vi "LS Durability One Hour Main (RT).vi"() -> ()   [LabVIEW 2013]
uses:
  Type Defs/App Config.ctl
  Type Defs/Controller Names.ctl
  SubVIs/Data Logger/Data Log Init.ctl
  Controls/Alarm Config.ctl
  Controls/Alarm Definition.ctl
  Controls/Alarm Profile Config.ctl
  Type Defs/Controller List.ctl
  Controls/Tank CMDs.ctl
  Controls/Controller Config.ctl
  Controls/Pump Data.ctl
  Controls/Tank Data.ctl
  Controls/HMI Cluster.ctl
  Controls/HMI Header.ctl
  Controls/HMI Tog Buttons.ctl
  Controls/HMI Mom Buttons.ctl
  Type Defs/LS Data.ctl
  Type Defs/Sequence States.ctl
  Controls/App Global Mode.ctl
  Controls/RPi HMI Mode.ctl
  Controls/Email Mode.ctl
  Type Defs/Pump Data Mode.ctl
  SubVIs/Watlow Modbus/Modbus Mode.ctl
  SubVIs/Watlow Modbus/Modbus Variable.ctl
  Controls/HMI Global Mode.ctl
  <vilib>/FPGAPlugInAG/sbRIO-9626/niLvFpga_Open_sbRIO-9626.vi
  <vilib>/Utility/error.llb/Error Cluster From Error Code.vi
  <vilib>/rvi/errors/niLvFpgaAdjustHostInterfaceError.vi
  <vilib>/Utility/file.llb/Write To Spreadsheet File (string).vi
  <vilib>/rvi/interface/nirviOpenFPGA/nirviOpenFPGA.xnode
  Controls/FPGA_OneHour_Reference.ctl
  FPGA Bitfiles/LSDurabilityMain_Alternate.lvbitx
  <vilib>/rvi/interface/nirviReadWriteControl/nirviReadWriteControl.xnode
  <vilib>/Utility/config.llb/NI_LVConfig.lvlib
  Controls/Power Supply Global Mode.ctl
  SubVIs/Data Logger/Data Logger Mode.ctl
  SubVIs/Data Logger/Data Log Start.ctl
  <vilib>/rvi/errors/niLvFpgaMergeErrorWithErrorCode.vi
  NiFpgaLv.dll
panel:
  in  "Data File Name:":string
  in  "pb.Run Profile":bool
  in  "Bank 2":T1={"7"=TRUE, "8"=TRUE, "9"=TRUE, "10"=TRUE, "11"=TRUE, "12"=TRUE}
  in  "Bank 1":T2={"1"=TRUE, "2"=TRUE, "3"=TRUE, "4"=TRUE, "5"=TRUE, "6"=TRUE} caption="Present"
  out "Email Alarms Disabled":bool
  out "Recording":bool
  in  "Disable Alarm Email":bool
  in  "Temp Tolerance":dbl=3.0 min=0.0 max=999999.0 step=1.0
  in  "Thermocouple":enum16{"2 TC/2 Tanks", "1 TC/1 Tank"}(ring)
  out "ADC Errors":i32
  in  "pb.Tare Pressure":bool
  in  "Data Log Enabled":bool=TRUE
  in  "RPMhyst":fxp<+,25,6>=1.0
  in  "pb.FuelChange":bool
  in  "Controller Type:":T3
  in  "Target Pressure:":dbl
  in  "Target Voltage:":dbl
  in  "Tank 1 Fuel Type:":string
  in  "Tank 2 Fuel Type:":string
  in  "Stagger Time (ms):":i32
  out "Current Step:":i32=2
  out "Step Time Left:":dbl=0.21101045608520508
  out "Cycles Completed:":u32=17
  in  "pb.Cycle Reset":bool
  in  "Serial Numbers":T4
  out "Read Inputs (ms)":u32
  out "Update Screen (ms)":u32
  out "Run Step (ms)":u32
  in  "Fuel Change Tab":enum32{"Page 1", "Page 2"}(tab)
  in  "pb.Fuel Change OK":bool
  in  "Reset Tab":enum32{"Page 1", "Page 2"}(tab)
  in  "pb.Reset OK":bool
  in  "pb.Reset Cancel":bool
  in  "Save As Tab":enum32{"Page 1", "Page 2"}(tab)
  in  "New Profile Name:":string
  in  "pb.Save As OK":bool
  in  "pb.Save As Cancel":bool
  in  "Alarm Tab":enum32{"Page 1", "Page 2"}(tab)
  out "Alarm Message":string
  in  "pb.Alarm OK":bool
  in  "Set Time Tab":enum32{"Page 1", "Page 2"}(tab)
  in  "pb.Set Time OK":bool
  in  "pb.Set Time Cancel":bool
  in  "New Time":dbl format="%<%H:%M:%S>t"
  in  "Pump Timers Tab":enum32{"Page 1", "Page 2"}(tab)=enum."Page 2"
  in  "Stop Time Enable":bool
  in  "Stop Time:":dbl format="%<%H:%M:%S>t"
  in  "pb.Time Reset All":bool
  out "Elapsed Time:":dbl[](array[numeric]) format="%<%H:%M:%S>t"
  in  "pb.Resets":bool[](array[boolean])=[FALSE, FALSE, FALSE, FALSE, FALSE, FALSE]
  in  "pb.Sets":bool[](array[boolean])=[FALSE, FALSE, FALSE, FALSE, FALSE, FALSE]
  in  "LS Serial Numbers":T5 caption="Serial Numbers"
  out "CPU Usage:":dbl=7.74131899555212 format="%.1f"
  in  "Live Data Tab":enum32{"Page 1", "Page 2", "Page 3"}(tab)=enum."Page 2"
  in  "Controller\nCMD":dbl[](array[numeric])=[0.0, 0.0, 0.0, 0.0, 0.0, 0.0] format="%#.2f"
  out "Speed":dbl[](array[numeric]) caption="Speed\n(RPM)" format="%#.0f"
  out "ControllerCurrent":dbl[](array[numeric])=[0.015201568603515625, 0.00335693359375, 0.003021240234375, 0.12260055541992188, 0.06085968017578125, 0.052234649658203125] caption="Controller\nCurrent\n(DC)" format="%.1f"
  out "PumpCurrent":dbl[](array[numeric])=[0.015201568603515625, 0.00335693359375, 0.003021240234375, 0.12260055541992188, 0.06085968017578125, 0.052234649658203125] caption="Pump\nCurrent\n(RMS)" format="%.1f"
  out "Flow":dbl[](array[numeric])=[0.0, 0.0, 0.0, 0.125, 0.0625, 0.0625] caption="Flow\n(L/H)" format="%#.0f"
  out "Pressure":dbl[](array[numeric])=[0.015201568603515625, 0.00335693359375, 0.003021240234375, 0.12260055541992188, 0.06085968017578125, 0.052234649658203125] caption="Pressure\n(kPa)" format="%#.0f"
  out "Ave. Speed":dbl=7.74131899555212 format="%.1f"
  out "Voltages":dbl[](array[numeric])=[0.015201568603515625, 0.00335693359375, 0.003021240234375, 0.12260055541992188, 0.06085968017578125, 0.052234649658203125] caption="Pump\nVoltage\n(V)" format="%.1f"
  in  "Reset Anomalies":bool
  in  "Reset Total Cycles":bool
  out "Anomalies (Last Cycle)":i32[](array[numeric]) caption="Anomalies\n(Last Cycle)" format="%#.0f"
  out "Anomalies/Cycle":i32[](array[numeric]) caption="Anomalies/\nCycle" format="%#.0f"
  out "Cycles":u32[](array[numeric]) format="%#.0f"
  out "Anomalies Total":i32[](array[numeric]) caption="Anomalies\nTotal" format="%#.0f"
  out "Steps":u32[](array[numeric]) format="%#.0f"
  out "Total Cycles":u32[](array[numeric]) caption="Total\nCycles" format="%#.0f"
  in  "Reset Opens":bool
  out "Opens":i32[](array[numeric]) format="%#.0f"
  in  "App Config":T6={"Location"="Tanks 162-163", "Profiles Path"=path "c:/Profiles", "Current Profile"="", "CA Number"="", "Cycles Completed"=0, "Controller Type:"=enum."Kuhnke", "Stagger Time (ms)"=0, "Tank 1 Fuel"="", "Tank 2 Fuel"="", "Serial Numbers"={"Position 1 SN"="", "Position 2 SN"="", "Poaition 3 SN"="", "Position 4 SN"="", "Position 5 SN"="", "Position 6 SN"=""}, "Pumps Present"={"Pump 1"=FALSE, "Pump 2"=FALSE, "Pump 3"=FALSE, "Pump 4"=FALSE, "Pump 5"=FALSE, "Pump 6"=FALSE}, "VoltCtrlRef"="", "VoltageSelect"=FALSE, "Watlow Present"=TRUE, "Temp 1"=0.0, "Temp 2"=0.0, "V_Run PI?"=FALSE, "Voltage Limits"={"V_Step"=1e-05, "V_CmdMax"=0.0, "V_CmdMin"=0.0}, "Voltage Far PI"={"V_FarSlew"=10.0, "V_FarKp"=0.0, "V_FarKi"=0.0}, "Voltage Mid PI"={"V_MidSlew"=10.0, "V_MidKp"=0.0, "V_MidKi"=0.0}, "Voltage Close PI"={"V_CloseSlew"=10.0, "V_CloseKp"=0.0, "V_CloseKi"=0.0}, "Voltage Scale"={"V_FFm"=0.0, "V_FFb"=0.0}, "Voltage Cutoffs"={"V_MidCutoff"=0.0, "V_CloseCutoff"=0.0}, "Pressure Scale"={"Pres_FFm"=1e-05, "Pres_FFb"=0.0}, "Temp Format"=0, "Temp Tolerance"=0.0, "Target Voltage"=0.0, "Target Pressure"=0.0, "Data Log Init"={"Data Path"=path "u:/Data", "Data Log Rate (S/s)"=1, "AKLH Rate (Hours/S)"=0.1, "Sync Time Offset (min)"=180, "IP Last 3"=0, "WebDAV IP"="10.31.176.36"}, "Email Handler IP"="10.30.189.34", "ADC Check"=FALSE, "3 Pump Tank"=TRUE, "Cycle Threshold:"=3.0, "Cycle Pts to Avg:"=3, "Anomaly Threshold:"=3.0, "Normal Steps:"=3, "Step Threshold:"=3.0} {"Step Threshold:" min=0.0 max=999999.0 step=1.0; "Normal Steps:" max=999999 step=1; "Anomaly Threshold:" min=0.0 max=999999.0 step=1.0; "Cycle Pts to Avg:" max=999999 step=1; "Cycle Threshold:" min=0.0 max=999999.0 step=1.0}
  in  "Monitoring Tab":enum32{"Page 1", "Page 2"}(tab)
  out "Avg Press:":dbl=7.74131899555212
  in  "pb.E Stop":bool
  in  "Ignition Relay":T8
  in  "Power Relay":T8
  out "Temp2":dbl caption="Tank 2 Temp (C):" format="%.1f"
  out "Temp1":dbl caption="Tank 1 Temp (C):" format="%.1f"
  out "PS Actual (V):":dbl format="%.2f"
  in  "Power Supply Cmd:":dbl min=0.0 max=20.0 format="%#.2f"
  in  "PressureCMD":dbl caption="Pressure Cmd:" min=0.0 max=825.0 format="%#.2f"
  in  "Pumps Present":T8={"Pump 1"=TRUE, "Pump 2"=TRUE, "Pump 3"=TRUE, "Pump 4"=TRUE, "Pump 5"=TRUE, "Pump 6"=TRUE}
  in  "Tank 1 Temp Cmd:":dbl caption="deg C"
  in  "Tank 2 Temp Cmd:":dbl caption="deg C"
  in  "Title Tab":enum32{"Page 1", "Page 2"}(tab)
  in  "Title":string="LS Durability ONE HOUR Test, v1.4"
  out "Time/Date":string
  in  "Login":bool
  in  "pb.Stop Profile":bool
  in  "Main Tab":T9(tab)
  in  "Recording\nFrequency (Hz): 2":i32=2000
  in  "Recording\nDuration (s): 2":i32=3600
  in  "Record Constant":bool
  in  "Detection Mode:":u16(ring) items=["Anomalies", "Opens"]
  in  "Record During Profile":bool
  in  "Recording\nFrequency (Hz):":i32=1000
  in  "Recording\nDuration (s):":i32=10
  in  "Interval Between\nRecordings (s):":i32=600
  in  "LS Power (Freq):":dbl=4.1 min=0.1
  in  "LS Power (Duty):":dbl=1.64
  in  "Bank 2 Power State:":u16(ring) items=["0 - Off", "1 - On", "2 - Pulsing"]
  in  "Bank 1 Power State:":u16(ring) items=["0 - Off", "1 - On", "2 - Pulsing"]
  in  "CA Number:":string
  in  "Profile Name:":string(combo)="test"
  in  "pb.Save As":bool
  out "Location:":string
  in  "Profile:":string[][](table)=[["1", "2.0", "0.0", "0.0", "0.0", "67.6", "67.6", "67.6"], ["2", "1.0", "0.0", "0.0", "0.0", "10.0", "10.0", "10.0"]]
  out "Step:":i32=1
  out "Time:":i32=1
  out "Recording":bool
  out "Waveform Chart":dbl(graph)
  in  "Pause":bool
  in  "Position":i32=1 min=1 max=12 step=1
  in  "Subtract Noise":bool
  in  "Anomaly Threshold:":dbl=3.0 min=0.0 max=999999.0 step=1.0
  in  "Normal Steps:":u32=3 max=999999 step=1
  in  "Step Threshold:":dbl=3.0 min=0.0 max=999999.0 step=1.0
  in  "Cycle Pts to Avg:":i32=3 min=0 max=999999 step=1
  in  "Cycle Threshold:":dbl=3.0 min=0.0 max=999999.0 step=1.0
  in  "Note Tab":enum32{"Page 1", "Page 2"}(tab)
  in  "Stop Profile Note":string
  in  "pb.Note OK":bool
  in  "pb.Note Cancel":bool
  in  "Second Step Check":bool
  in  "Alarm Config":T10
  in  "WebDAV Push":bool
  in  "Concat Data":bool
  in  "Cutoffs":cluster{"Mid Range":dbl, "Close Range":dbl} {"Close Range" min=-100000.0 max=100000.0 step=1e-05 format="%#.5f"; "Mid Range" min=-100000.0 max=100000.0 step=1e-05 format="%#.5f"}
  in  "Mid PI":cluster{"Slew Rate":dbl, "Kp":dbl, "Ki":dbl}={"Slew Rate"=10.0, "Kp"=0.0, "Ki"=0.0} {"Ki" min=-100000.0 max=100000.0 step=1e-05 format="%#.5f"; "Kp" min=-100000.0 max=100000.0 step=1e-05 format="%#.5f"; "Slew Rate" min=0.0 max=1000000.0 step=0.01 format="%#.5f"}
  in  "Close PI":cluster{"Slew Rate":dbl, "Kp":dbl, "Ki":dbl}={"Slew Rate"=10.0, "Kp"=0.0, "Ki"=0.0} {"Ki" min=-100000.0 max=100000.0 step=1e-05 format="%#.5f"; "Kp" min=-100000.0 max=100000.0 step=1e-05 format="%#.5f"; "Slew Rate" min=0.0 max=1000000.0 step=0.01 format="%#.5f"}
  in  "Pressure Scale":cluster{"M":dbl, "B":dbl}={"M"=1e-05, "B"=0.0} {"B" min=-100000.0 max=100000.0 step=1e-05 format="%#.5f"; "M" min=-100000.0 max=100000.0 step=1e-05 format="%#.5f"}
  in  "Closed Loop Voltage":bool
  in  "Voltage Limits":cluster{"Step":dbl, "Max":dbl, "Min":dbl}={"Step"=1e-05, "Max"=0.0, "Min"=0.0} {"Min" min=0.0 max=10.0 step=1e-05 format="%#.5f"; "Max" min=0.0 max=10.0 step=1e-05 format="%#.5f"; "Step" min=0.0 max=100.0 step=1e-05 format="%#.5f"}
  in  "Far PI":cluster{"Slew Rate":dbl, "Kp":dbl, "Ki":dbl}={"Slew Rate"=10.0, "Kp"=0.0, "Ki"=0.0} {"Ki" min=-100000.0 max=100000.0 step=1e-05 format="%#.5f"; "Kp" min=-100000.0 max=100000.0 step=1e-05 format="%#.5f"; "Slew Rate" min=0.0 max=1000000.0 step=0.01 format="%#.5f"}
  in  "Voltage Scale":cluster{"M":dbl, "B":dbl} {"B" min=-100000.0 max=100000.0 step=1e-05 format="%#.5f"; "M" min=-100000.0 max=100000.0 step=1e-05 format="%#.5f"}
  # "Fuel Change was logged."
  # "Are you sure you want to reset?"
  # "Enter a new elapsed time."
  # "Pump Timers"
  # "Live Data"
  # "Level Sensor Monitor"
  # "Level Sensor Monitor"
  # "Manual Control"
  # "V"
  # "kPa"
  # "degC"
  # "degC"
  # "Data file note as to reason for stopping profile:"
  # "Voltage Control"
  # "Pressure Control"
  # "Data Server"
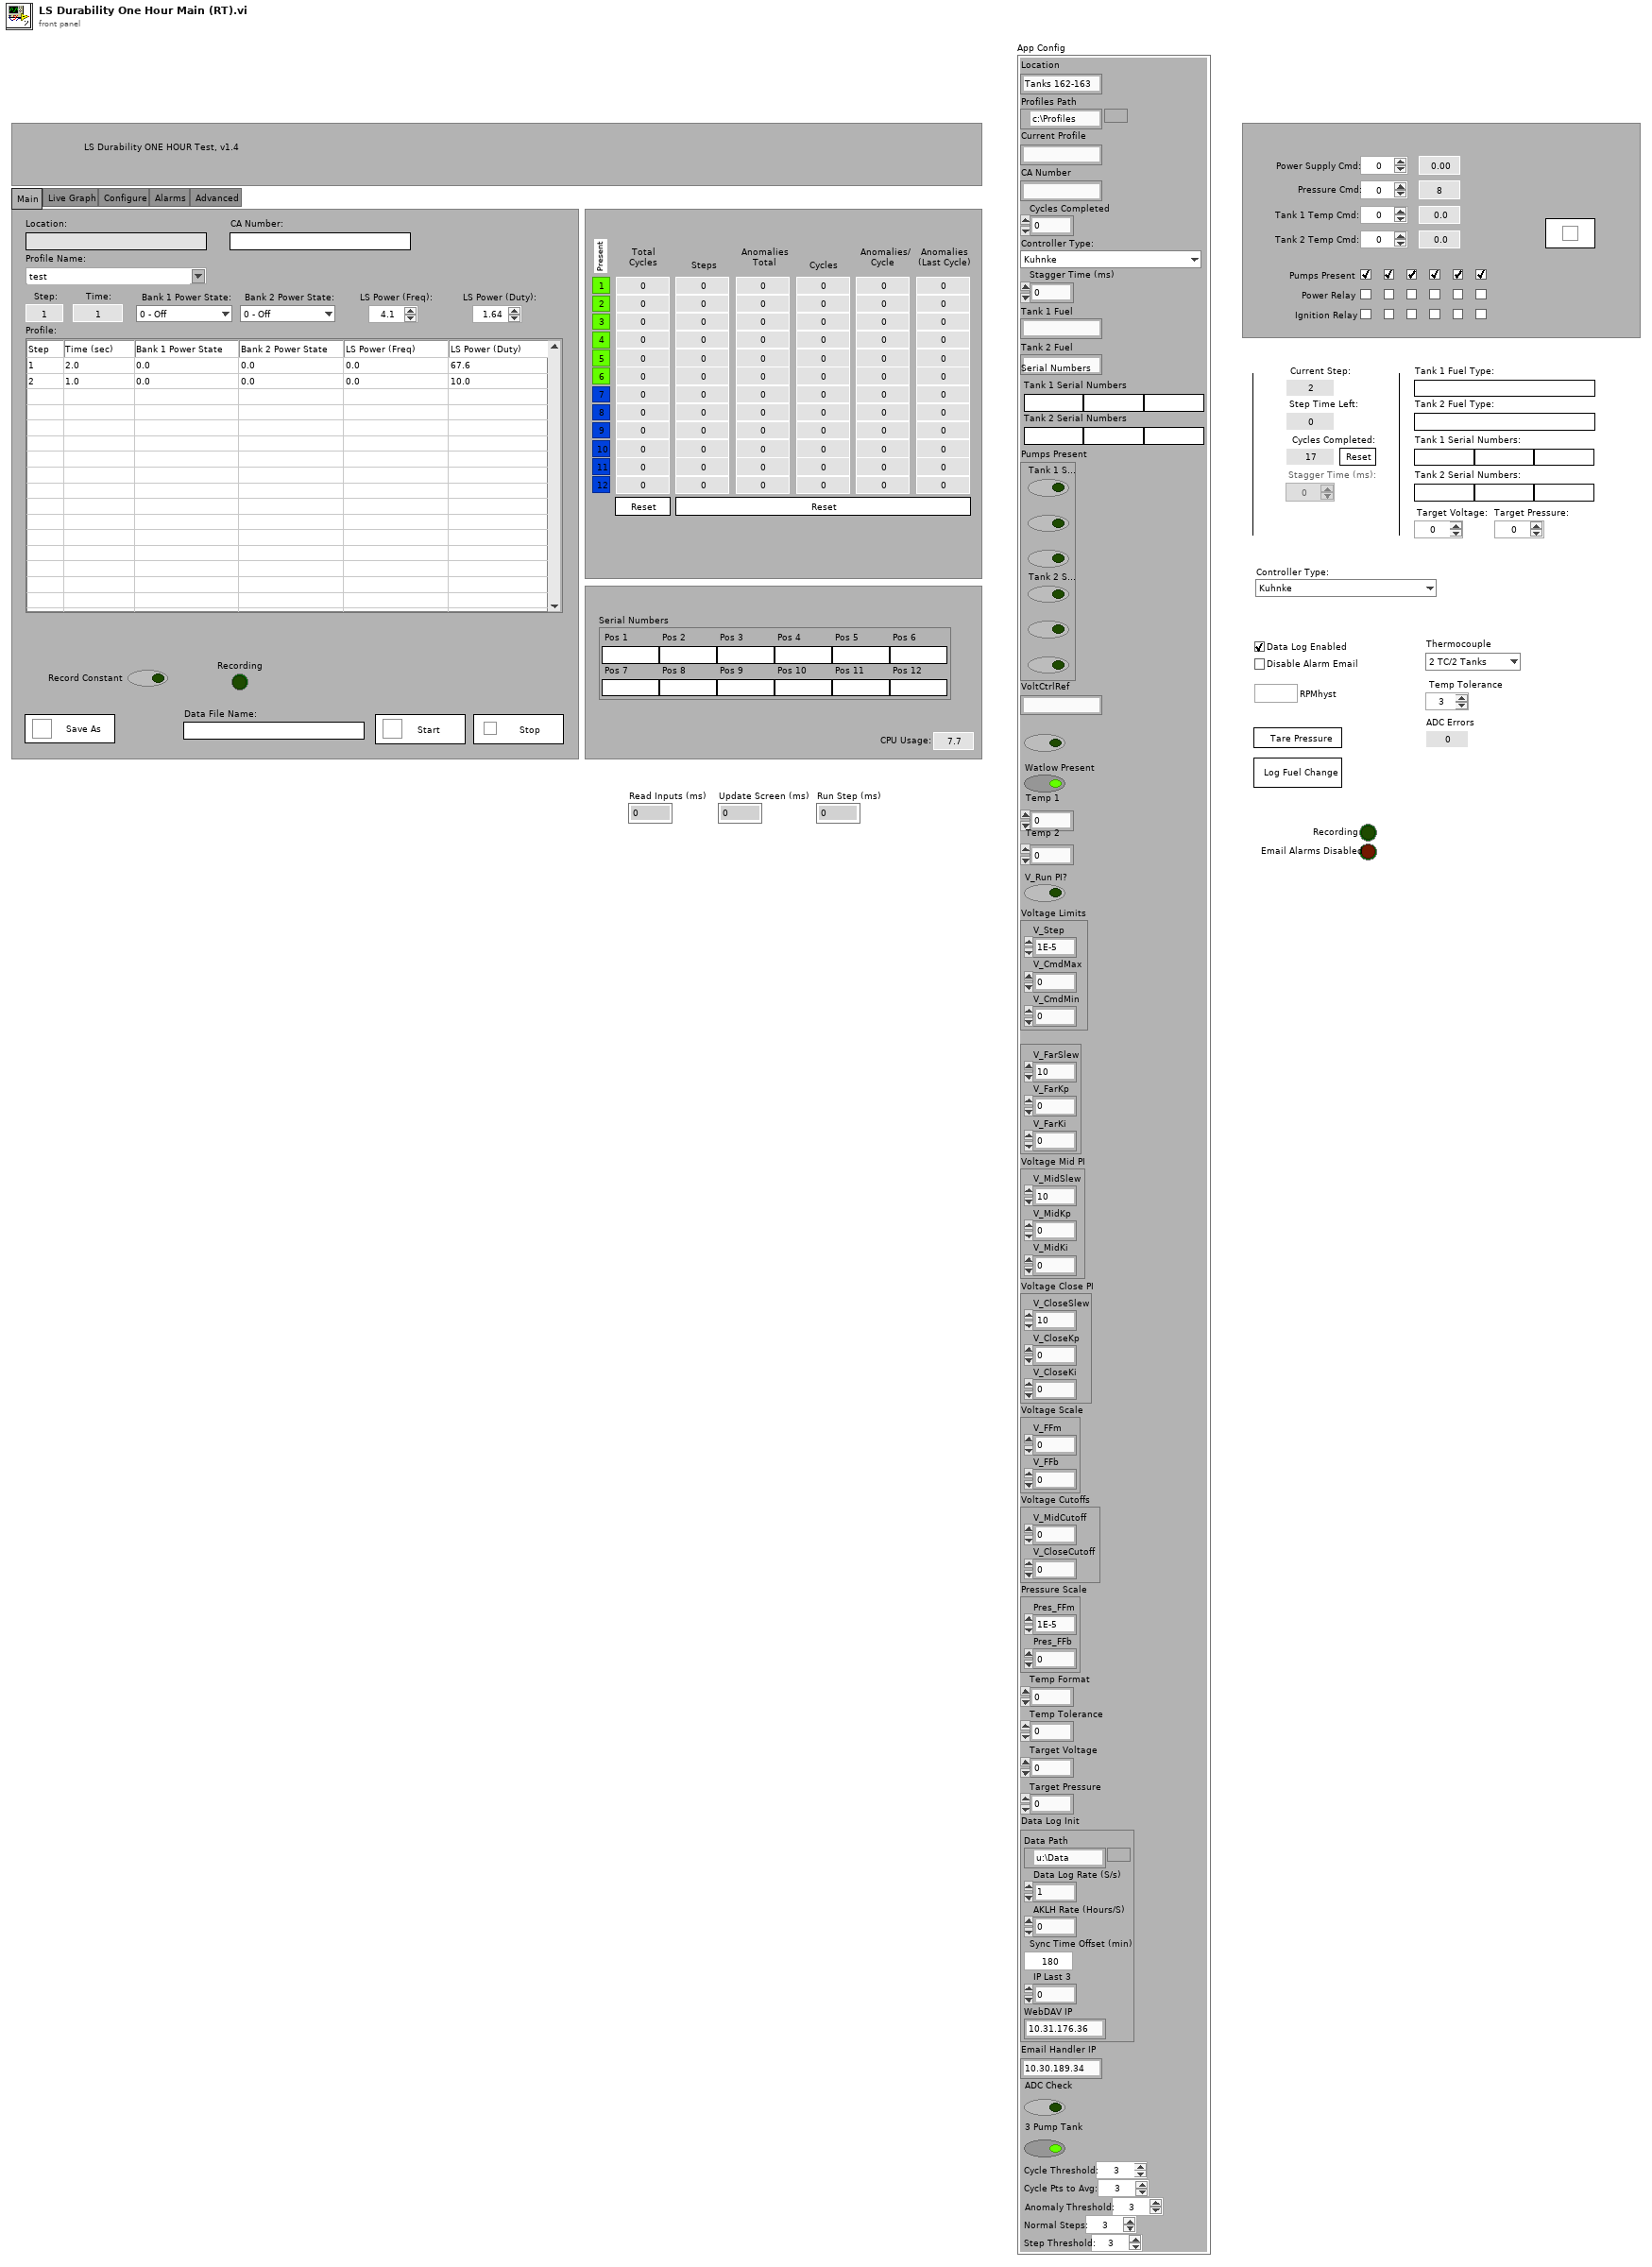
[diagram p1: front panel]
types:
  T1 = cluster{"7":bool, "8":bool, "9":bool, "10":bool, "11":bool, "12":bool}
  T2 = cluster{"1":bool, "2":bool, "3":bool, "4":bool, "5":bool, "6":bool}
  T3 = typedef "Controller Names.ctl" = enum16{"Kuhnke", "Helbako BLDC", "Conti", "Hella BLDC OL PWM", "Hella BLDC Turbine OL PWM", "Hella BLDC Pressure", "Helbako (old)", "TI PWM", "PSA", "Hella Gas", "Hella Diesel", "8 Comm", "10 Comm", "8 Comm Hella", "10 Comm Hella", "8 Comm Omron", "10 Comm Omron", "8 Comm Nissan", "10 Comm Nissan"}
  T4 = cluster{"Position 1 SN":string, "Position 2 SN":string, "Position 3 SN":string, "Position 4 SN":string, "Position 5 SN":string, "Position 6 SN":string}
  T5 = cluster{"Pos 1":string, "Pos 2":string, "Pos 3":string, "Pos 4":string, "Pos 5":string, "Pos 6":string, "Pos 7":string, "Pos 8":string, "Pos 9":string, "Pos 10":string, "Pos 11":string, "Pos 12":string}
  T6 = typedef "App Config.ctl" = cluster{"Location":string, "Profiles Path":path, "Current Profile":string, "CA Number":string, "Cycles Completed":u32, "Controller Type:":T3, "Stagger Time (ms)":i32, "Tank 1 Fuel":string, "Tank 2 Fuel":string, "Serial Numbers":cluster{"Position 1 SN":string, "Position 2 SN":string, "Poaition 3 SN":string, "Position 4 SN":string, "Position 5 SN":string, "Position 6 SN":string}, "Pumps Present":cluster{"Pump 1":bool, "Pump 2":bool, "Pump 3":bool, "Pump 4":bool, "Pump 5":bool, "Pump 6":bool}, "VoltCtrlRef":string, "VoltageSelect":bool, "Watlow Present":bool, "Temp 1":dbl, "Temp 2":dbl, "V_Run PI?":bool, "Voltage Limits":cluster{"V_Step":dbl, "V_CmdMax":dbl, "V_CmdMin":dbl}, "Voltage Far PI":cluster{"V_FarSlew":dbl, "V_FarKp":dbl, "V_FarKi":dbl}, "Voltage Mid PI":cluster{"V_MidSlew":dbl, "V_MidKp":dbl, "V_MidKi":dbl}, "Voltage Close PI":cluster{"V_CloseSlew":dbl, "V_CloseKp":dbl, "V_CloseKi":dbl}, "Voltage Scale":cluster{"V_FFm":dbl, "V_FFb":dbl}, "Voltage Cutoffs":cluster{"V_MidCutoff":dbl, "V_CloseCutoff":dbl}, "Pressure Scale":cluster{"Pres_FFm":dbl, "Pres_FFb":dbl}, "Temp Format":i32, "Temp Tolerance":dbl, "Target Voltage":dbl, "Target Pressure":dbl, "Data Log Init":T7, "Email Handler IP":string, "ADC Check":bool, "3 Pump Tank":bool, "Cycle Threshold:":dbl, "Cycle Pts to Avg:":i32, "Anomaly Threshold:":dbl, "Normal Steps:":u32, "Step Threshold:":dbl}
  T7 = typedef "Data Log Init.ctl" = cluster{"Data Path":path, "Data Log Rate (S/s)":u32, "AKLH Rate (Hours/S)":dbl, "Sync Time Offset (min)":i32, "IP Last 3":i32, "WebDAV IP":string}
  T8 = cluster{"Pump 1":bool, "Pump 2":bool, "Pump 3":bool, "Pump 4":bool, "Pump 5":bool, "Pump 6":bool}
  T9 = enum32{"Main", "Live Graph", "Configure", "Alarms", "Advanced"}
  T10 = typedef "Alarm Config.ctl" = cluster{"Alarms:":T11[], "Profile Sync:":T12}
  T11 = typedef "Alarm Definition.ctl" = cluster{"Description:":string, "Enabled:":bool, "Data Index:":i32, "Data Type:":string, "Low Limit:":dbl, "High Limit:":dbl, "Trip Time:":u32, "Profile Sync:":bool}
  T12 = typedef "Alarm Profile Config.ctl" = cluster{"Trip Time:":u32, "Consecutive Trips:":i32}
  T13 = cluster{"LS Power (Freq):":dbl, "LS Power (Duty):":dbl, "Bank 1 Present":cluster{"1":bool, "2":bool, "3":bool, "4":bool, "5":bool, "6":bool}, "Bank 2 Present":cluster{"7":bool, "8":bool, "9":bool, "10":bool, "11":bool, "12":bool}, "Data File Name:":string, "Record Bursts":bool, "RecInterval(s)":i32, "RecDuration(s)":i32, "RecFrequeny (Hz)":i32, "DetectionMode":i32, "Serial Numbers":string[], "Record Constant":bool, "2nd Step Check":bool, "Bias Resistances":dbl[], "Voltage(T)/Resistance(F)":bool}
  T14 = cluster{"LS Power (Freq):":dbl, "LS Power (Duty):":dbl, "Bank 1 Present":cluster{"1":bool, "2":bool, "3":bool, "4":bool, "5":bool, "6":bool}, "Bank 2 Present":cluster{"7":bool, "8":bool, "9":bool, "10":bool, "11":bool, "12":bool}, "Data File Name:":string, "Record Bursts":bool, "RecInterval(s)":i32, "RecDuration(s)":i32, "RecFrequeny (Hz)":i32, "DetectionMode":i32, "Serial Numbers":string[], "Record Constant":bool, "2nd Step Check":bool}
  T15 = typedef "Sequence States.ctl" = enum16{"Main", "Init Files", "Init", "Unused", "Save As", "Start Profile", "Check Step Time", "Alarm", "Alarm Dismiss", "Run Step", "Stop Profile", "Cycle Reset", "Time Reset", "Time Reset All", "Time Set", "Tare CTs", "Save Profile", "Open Profile", "Get Profiles", "Update Screen", "Update Controls", "Save App Config", "Write Outputs", "Disable Background", "Enable Background", "Get/Release Control", "Log Fuel Change", "Fuel Change Popup", "Read Inputs", "Remote Timer Reset", "Controller Change", "Get Alarms", "Init Alarms", "Save Alarms", "Voltage Selection", "Set Watlow Temp 1", "Set Watlow Temp 2", "Get Pressure", "Write Tare Pressure", "Adjust Controls", "Reinit ADC", "Write Initial Times", "Write Pumps Present", "HMI Command", "Save Pump Times", "Check Pump Stop Time", "Save LS App Config", "Init Data File", "Reset LS Cycles", "Reset Anomalies", "Reset Opens", "Save LS Data", "Save LS Test Data", "Check Serial Numbers", "Main Tab", "Allow Data Note"}
  T16 = typedef "LS Data.ctl" = cluster{"Total Cycles":u32[], "Steps":u32[], "Anomalies Total":i32[], "Cycles":u32[], "Anomalies/Cycle":i32[], "Anomalies (Last Cycle)":i32[], "Opens":i32[]}
  T17 = typedef "HMI Cluster.ctl" = cluster{"Error":errorcluster, "COM Ref":refnum<visa-resource-name>, "Pump Data":T18, "Tank Data":cluster{"PS Actual (V):":dbl, "Temp1":dbl, "Temp2":dbl}, "Power Relays":cluster{"Pump 1":bool, "Pump 2":bool, "Pump 3":bool, "Pump 4":bool, "Pump 5":bool, "Pump 6":bool}, "Pump CMDs":dbl[], "HMI Header":T19, "Tank CMDs":T20, "HMI Tog Buttons":T21, "In Test":bool, "HMI Command":bool, "HMI Mom Buttons":T22, "Controller Config":T23, "Alarm":bool, "Alarm Message 1":string, "Alarm Message 2":string, "Recording":bool, "Serial Numbers":string[], "Pumps Present":bool[]}
  T18 = typedef "Pump Data.ctl" = cluster{"Voltages":dbl[], "PumpCurrent":dbl[], "Speed":dbl[], "ControllerCurrent":dbl[], "Pressure":dbl[], "Flow":dbl[], "Elapsed Time (Display)":dbl[], "Avg Pressure":dbl, "Avg Speed":dbl, "Elapsed Time":dbl[]}
  T19 = typedef "HMI Header.ctl" = cluster{"Line 1":string, "Line 2":string, "Line 3":string, "Line 4":string}
  T20 = typedef "Tank CMDs.ctl" = cluster{"PS CMD":dbl, "Press CMD":dbl, "Temp 1 CMD":dbl, "Temp 2 CMD":dbl}
  T21 = typedef "HMI Tog Buttons.ctl" = cluster{"Start Test":bool, "Toggle Spare 1":bool, "Toggle Spare 2":bool, "Toggle Spare 3":bool, "Toggle Spare 4":bool, "Toggle Spare 5":bool}
  T22 = typedef "HMI Mom Buttons.ctl" = cluster{"Stop":bool, "Reset Timers":bool, "Log Fuel Change":bool, "Alarm Dismiss":bool}
  T23 = typedef "Controller Config.ctl" = cluster{"Controller Name":T3, "CommSeg":i32, "PWM?":bool, "Frequency":i32, "Low Command":dbl, "High Command":dbl, "Stop Command":dbl, "Command Step":dbl, "Solenoid Stop?":bool, "Controller?":bool, "Invert PWM":bool}
  T24 = typedef "Tank Data.ctl" = cluster{"PS Actual (V):":dbl, "Temp1":dbl, "Temp2":dbl}
  T25 = typedef "Controller List.ctl" = cluster{"Controller Name":T3, "CommSeg":i32, "PWM?":bool, "Frequency":i32, "Low Command":dbl, "High Command":dbl, "Stop Command":dbl, "Command Step":dbl, "Solenoid Stop?":bool, "Controller?":bool, "Invert PWM":bool}[]
  T26 = cluster{"Error":errorcluster, "Profile":string[][], "App Config":T6, "Profiles":string[], "Current Step":i32, "Step Time Left":dbl, "Run Profile":bool, "Step Start Time":dbl, "Step Time":dbl, " # of Steps":i32, "Screen Timer":u32, "Last Profile Time":dbl, "Controller CMDs":dbl[], "Client?":bool, "pb.Run Profile":bool, "pb.Resets":bool[], "pb.Sets":bool[], "Initial Times":dbl[], "Pressure Offsets":dbl[], "Login":bool, "Stagger Counter":i32, "New Step":bool, "Inputs Timer":u32, "Tank Data":T24, "Voltage Enable":bool, "Power Relay":cluster{"Pump 1":bool, "Pump 2":bool, "Pump 3":bool, "Pump 4":bool, "Pump 5":bool, "Pump 6":bool}, "Ignition Relay":cluster{"Pump 1":bool, "Pump 2":bool, "Pump 3":bool, "Pump 4":bool, "Pump 5":bool, "Pump 6":bool}, "Controller List":T25, "Alarm Config":T10, "Alarm Config Path":path, "Trip Counters":i32[], "Previous Times":u32[], "Alarm Message 1":string, "Alarm Message 2":string, "Prev ON Times":u32[], "CalArray":dbl[][], "Tank CMDs":T20, "Controller Config":T23, "Fuel Log Path":path, "Pump Data":T18, "Alarm Latch":bool, "Time/Date":string, "Recording":bool, "HMI":T17, "WebDAV Push":bool, "Email Alarms Disabled":bool, "Concat Data":bool, "LS Data":T16, "Main Tab":enum32{"Main", "Live Graph", "Configure", "Alarms", "Advanced"}, "LS App Config":cluster{"LS Power (Freq):":dbl, "LS Power (Duty):":dbl, "Bank 1 Present":cluster{"1":bool, "2":bool, "3":bool, "4":bool, "5":bool, "6":bool}, "Bank 2 Present":cluster{"7":bool, "8":bool, "9":bool, "10":bool, "11":bool, "12":bool}, "Data File Name:":string, "Record Bursts":bool, "RecInterval(s)":i32, "RecDuration(s)":i32, "RecFrequeny (Hz)":i32, "DetectionMode":i32, "Serial Numbers":string[], "Record Constant":bool, "2nd Step Check":bool, "Bias Resistances":dbl[], "Voltage(T)/Resistance(F)":bool}, "Bank 1 State:":u16, "Bank 2 State:":u16, "LS Data Filepath":path, "Initial LS Data":T16, "day of month":i32}
  T27 = typedef "FPGA_OneHour_Reference.ctl" = refnum<k20>
  T28 = typedef "App Global Mode.ctl" = enum16{"Read", "Write Client", "Write Login"}
  T29 = typedef "Data Logger Mode.ctl" = enum16{"Init", "Main", "Start", "Stop"}
  T30 = cluster{"Running?":bool, "Profile Record":bool, "RecordInterval":i32, "RecordDuration":i32, "RecordFreq":i32, "Data Filepath":path, "Hr Record":bool, "Serial Numbers":string[]}
  T31 = enum8{"Enabled", "Disabled", "Disabled and Grayed Out"}
  T32 = enum16{"open", "replace", "create", "open or create", "replace or create", "replace or create with confirmation"}
  T33 = typedef "Data Log Start.ctl" = cluster{"App Config":T6, "Profile":string[][], "Controller Type":string, "Tank CMDs":T20}
  T34 = typedef "Power Supply Global Mode.ctl" = enum16{"Write Setpoint", "Write FreezePID", "Read"}
  T35 = typedef "RPi HMI Mode.ctl" = enum16{"Init", "Write Data", "Read from RPi", "Write to RPi"}
  T36 = typedef "Email Mode.ctl" = enum16{"Trigger Email", "Send Email"}
  T37 = typedef "Pump Data Mode.ctl" = enum16{"Read", "Write Data", "Write Cal", "Write Watlow Data", "Write Pressure Offsets", "Write Initial Times", "Write Pumps Present"}
  T38 = typedef "Modbus Variable.ctl" = enum16{"Temperature", "Setpoint"}
  T39 = typedef "Modbus Mode.ctl" = enum16{"Init", "Tank 1 Write", "Tank 2 Write", "Tank 1 Read", "Tank 2 Read"}
  T40 = typedef "HMI Global Mode.ctl" = enum16{"Read", "Write Cluster", "Reset Cmd"}
  T41 = cluster{"Position 1 SN":string, "Position 2 SN":string, "Poaition 3 SN":string, "Position 4 SN":string, "Position 5 SN":string, "Position 6 SN":string}
  T42 = cluster{"V_Step":dbl, "V_CmdMax":dbl, "V_CmdMin":dbl}
  T43 = cluster{"V_FarSlew":dbl, "V_FarKp":dbl, "V_FarKi":dbl}
  T44 = cluster{"V_MidSlew":dbl, "V_MidKp":dbl, "V_MidKi":dbl}
  T45 = cluster{"V_CloseSlew":dbl, "V_CloseKp":dbl, "V_CloseKi":dbl}
  T46 = typedef "LVDateTimeRec.ctl" = cluster{"fractional second":dbl, "second":i32, "minute":i32, "hour":i32, "day of month":i32, "month":i32, "year":i32, "day of week":i32, "day of year":i32, "DST":i32}
  T47 = typedef "NI_LVConfig.lvlib/Config Data RefNum.ctl" = refnum<k1>
  T48 = typedef "FPGA_Reference.ctl" = refnum<k20>
  T49 = cluster{"Serial Numbers[0]":string, "Serial Numbers[1]":string, "Serial Numbers[2]":string, "Serial Numbers[3]":string, "Serial Numbers[4]":string, "Serial Numbers[5]":string, "Serial Numbers[6]":string, "Serial Numbers[7]":string, "Serial Numbers[8]":string, "Serial Numbers[9]":string, "Serial Numbers[10]":string, "Serial Numbers[11]":string}
  T50 = cluster{"Controller Name":T3, "CommSeg":i32, "PWM?":bool, "Frequency":i32, "Low Command":dbl, "High Command":dbl, "Stop Command":dbl, "Command Step":dbl, "Solenoid Stop?":bool, "Controller?":bool, "Invert PWM":bool}
  T51 = cluster{"[0]":bool, "[1]":bool, "[2]":bool, "[3]":bool, "[4]":bool, "[5]":bool}
  T52 = cluster{"[0]":string, "[1]":string, "[2]":string, "[3]":string, "[4]":string, "[5]":string, "[6]":string, "[7]":string, "[8]":string, "[9]":string, "[10]":string, "[11]":string}
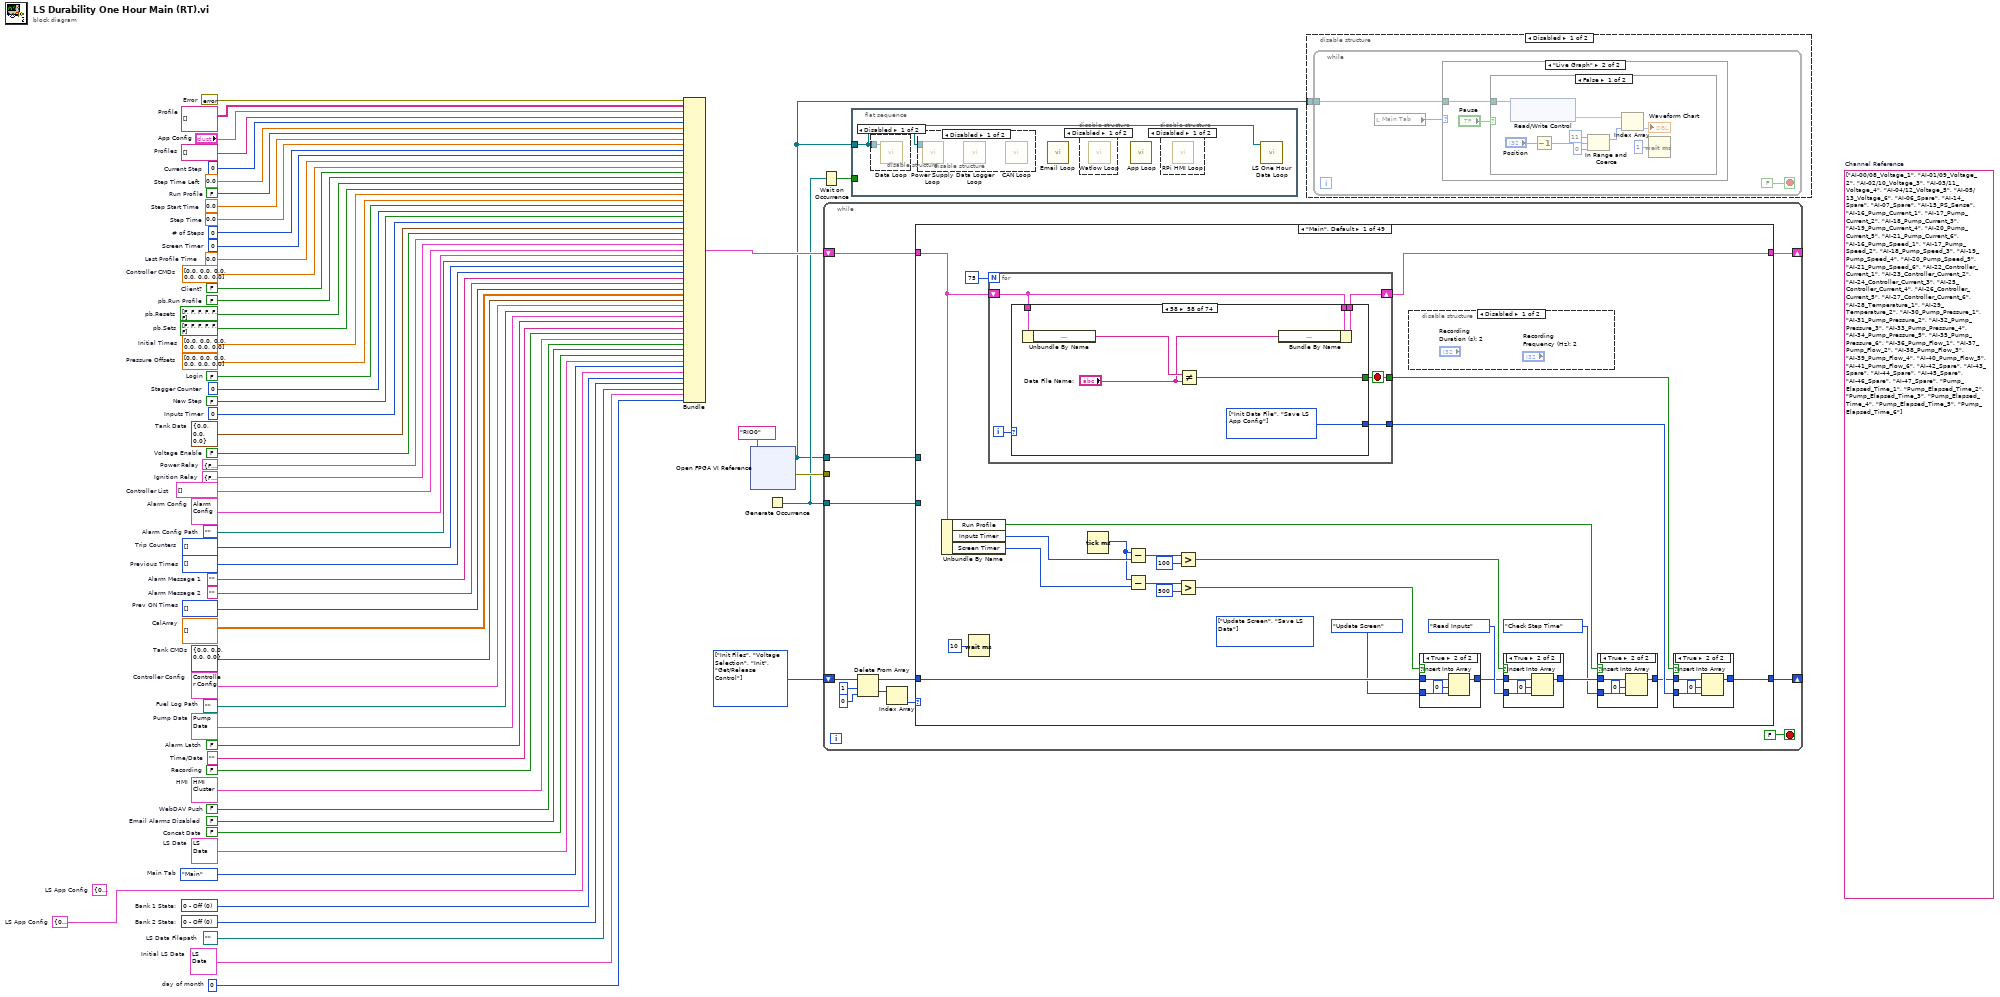
[diagram p0: block diagram]
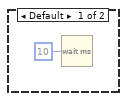
[diagram p2: hidden frame]
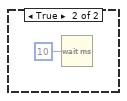
[diagram p3: hidden frame]
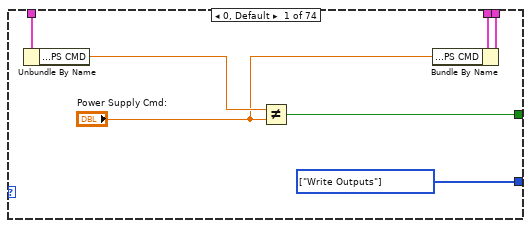
[diagram p14: hidden frame]
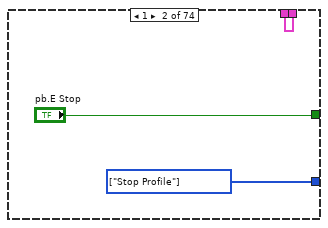
[diagram p15: hidden frame]
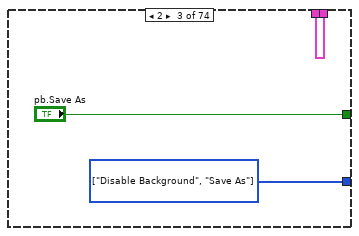
[diagram p16: hidden frame]
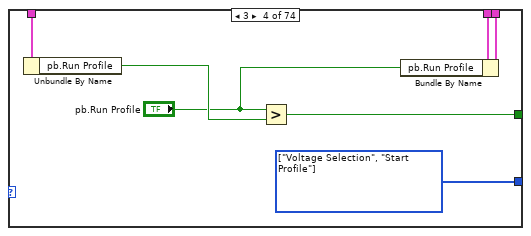
[diagram p17: hidden frame]
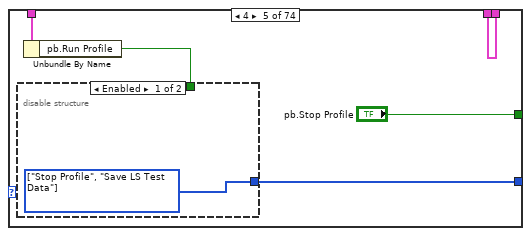
[diagram p18: hidden frame]
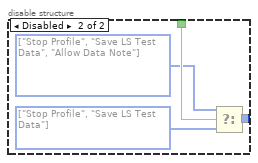
[diagram p19: hidden frame]
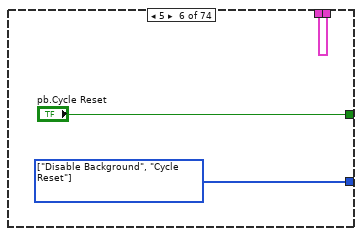
[diagram p20: hidden frame]
diagram:
  w1 = T13 {"LS Power (Freq):"=0.0, "LS Power (Duty):"=0.0, "Bank 1 Present"={"1"=TRUE, "2"=TRUE, "3"=TRUE, "4"=TRUE, "5"=TRUE, "6"=TRUE}, "Bank 2 Present"={"7"=TRUE, "8"=TRUE, "9"=TRUE, "10"=TRUE, "11"=TRUE, "12"=TRUE}, "Data File Name:"="", "Record Bursts"=FALSE, "RecInterval(s)"=600, "RecDuration(s)"=10, "RecFrequeny (Hz)"=1000, "DetectionMode"=0, "Serial Numbers"=["", "", "", "", "", "", "", "", "", "", "", ""], "Record Constant"=FALSE, "2nd Step Check"=FALSE, "Bias Resistances"=[681.0, 681.0, 681.0, 681.0, 681.0, 681.0, 681.0, 681.0, 681.0, 681.0, 681.0, 681.0], "Voltage(T)/Resistance(F)"=TRUE}  # LS App Config
  (unwired) T14 {"LS Power (Freq):"=0.0, "LS Power (Duty):"=0.0, "Bank 1 Present"={"1"=TRUE, "2"=TRUE, "3"=TRUE, "4"=TRUE, "5"=TRUE, "6"=TRUE}, "Bank 2 Present"={"7"=TRUE, "8"=TRUE, "9"=TRUE, "10"=TRUE, "11"=TRUE, "12"=TRUE}, "Data File Name:"="", "Record Bursts"=FALSE, "RecInterval(s)"=600, "RecDuration(s)"=10, "RecFrequeny (Hz)"=1000, "DetectionMode"=0, "Serial Numbers"=["", "", "", "", "", "", "", "", "", "", "", ""], "Record Constant"=FALSE, "2nd Step Check"=FALSE}  # LS App Config
  w2 = 0  # day of month
  (unwired) string[] ["AI-00/08_Voltage_1", "AI-01/09_Voltage_2", "AI-02/10_Voltage_3", "AI-03/11_Voltage_4", "AI-04/12_Voltage_5", "AI-05/13_Voltage_6", "AI-06_Spare", "AI-14_Spare", "AI-07_Spare", "AI-15_PS_Sense", "AI-16_Pump_Current_1", "AI-17_Pump_Current_2", "AI-18_Pump_Current_3", "AI-19_Pump_Current_4", "AI-20_Pump_Current_5", "AI-21_Pump_Current_6", "AI-16_Pump_Speed_1", "AI-17_Pump_Speed_2", "AI-18_Pump_Speed_3", "AI-19_Pump_Speed_4", "AI-20_Pump_Speed_5", "AI-21_Pump_Speed_6", "AI-22_Controller_Current_1", "AI-23_Controller_Current_2", "AI-24_Controller_Current_3", "AI-25_Controller_Current_4", "AI-26_Controller_Current_5", "AI-27_Controller_Current_6", "AI-28_Temperature_1", "AI-29_Temperature_2", "AI-30_Pump_Pressure_1", "AI-31_Pump_Pressure_2", "AI-32_Pump_Pressure_3", "AI-33_Pump_Pressure_4", "AI-34_Pump_Pressure_5", "AI-35_Pump_Pressure_6", "AI-36_Pump_Flow_1", "AI-37_Pump_Flow_2", "AI-38_Pump_Flow_3", "AI-39_Pump_Flow_4", "AI-40_Pump_Flow_5", "AI-41_Pump_Flow_6", "AI-42_Spare", "AI-43_Spare", "AI-44_Spare", "AI-45_Spare", "AI-46_Spare", "AI-47_Spare", "Pump_Elapsed_Time_1", "Pump_Elapsed_Time_2", "Pump_Elapsed_Time_3", "Pump_Elapsed_Time_4", "Pump_Elapsed_Time_5", "Pump_Elapsed_Time_6"]  # Channel Reference
  w8 = T15[] [enum."Init Files", enum."Voltage Selection", enum."Init", enum."Get/Release Control"] items=["Main", "Init Files", "Init", "Unused", "Save As", "Start Profile", "Check Step Time", "Alarm", "Alarm Dismiss", "Run Step", "Stop Profile", "Cycle Reset", "Time Reset", "Time Reset All", "Time Set", "Tare CTs", "Save Profile", "Open Profile", "Get Profiles", "Update Screen", "Update Controls", "Save App Config", "Write Outputs", "Disable Background", "Enable Background", "Get/Release Control", "Log Fuel Change", "Fuel Change Popup", "Read Inputs", "Remote Timer Reset", "Controller Change", "Get Alarms", "Init Alarms", "Save Alarms", "Voltage Selection", "Set Watlow Temp 1", "Set Watlow Temp 2", "Get Pressure", "Write Tare Pressure", "Adjust Controls", "Reinit ADC", "Write Initial Times", "Write Pumps Present", "HMI Command", "Save Pump Times", "Check Pump Stop Time", "Save LS App Config", "Init Data File", "Reset LS Cycles", "Reset Anomalies", "Reset Opens", "Save LS Data", "Save LS Test Data", "Check Serial Numbers", "Main Tab", "Allow Data Note"]
  w9 = T16 {"Total Cycles"=[0, 0, 0, 0, 0, 0, 0, 0, 0, 0, 0, 0], "Steps"=[0, 0, 0, 0, 0, 0, 0, 0, 0, 0, 0, 0], "Anomalies Total"=[0, 0, 0, 0, 0, 0, 0, 0, 0, 0, 0, 0], "Cycles"=[0, 0, 0, 0, 0, 0, 0, 0, 0, 0, 0, 0], "Anomalies/Cycle"=[0, 0, 0, 0, 0, 0, 0, 0, 0, 0, 0, 0], "Anomalies (Last Cycle)"=[0, 0, 0, 0, 0, 0, 0, 0, 0, 0, 0, 0], "Opens"=[0, 0, 0, 0, 0, 0, 0, 0, 0, 0, 0, 0]}  # Initial LS Data
  w10 = path ""  # LS Data Filepath
  w12 = u16 0 items=["0 - Off", "1 - On", "2 - Pulsing"]  # Bank 1 State:
  w11 = u16 0 items=["0 - Off", "1 - On", "2 - Pulsing"]  # Bank 2 State:
  w13 = T9."Main"  # Main Tab
  w14 = T16 {"Total Cycles"=[0, 0, 0, 0, 0, 0, 0, 0, 0, 0, 0, 0], "Steps"=[0, 0, 0, 0, 0, 0, 0, 0, 0, 0, 0, 0], "Anomalies Total"=[0, 0, 0, 0, 0, 0, 0, 0, 0, 0, 0, 0], "Cycles"=[0, 0, 0, 0, 0, 0, 0, 0, 0, 0, 0, 0], "Anomalies/Cycle"=[0, 0, 0, 0, 0, 0, 0, 0, 0, 0, 0, 0], "Anomalies (Last Cycle)"=[0, 0, 0, 0, 0, 0, 0, 0, 0, 0, 0, 0], "Opens"=[]}  # LS Data
  w15 = FALSE  # Concat Data
  w16 = FALSE  # Email Alarms Disabled
  w17 = FALSE  # WebDAV Push
  w18 = T17 {"Error"={"status"=FALSE, "code"=0, "source"=""}, "COM Ref"="", "Pump Data"={"Voltages"=[], "PumpCurrent"=[], "Speed"=[], "ControllerCurrent"=[], "Pressure"=[], "Flow"=[], "Elapsed Time (Display)"=[], "Avg Pressure"=0.0, "Avg Speed"=0.0, "Elapsed Time"=[]}, "Tank Data"={"PS Actual (V):"=0.0, "Temp1"=0.0, "Temp2"=0.0}, "Power Relays"={"Pump 1"=FALSE, "Pump 2"=FALSE, "Pump 3"=FALSE, "Pump 4"=FALSE, "Pump 5"=FALSE, "Pump 6"=FALSE}, "Pump CMDs"=[], "HMI Header"={"Line 1"="", "Line 2"="", "Line 3"="", "Line 4"=""}, "Tank CMDs"={"PS CMD"=0.0, "Press CMD"=0.0, "Temp 1 CMD"=0.0, "Temp 2 CMD"=0.0}, "HMI Tog Buttons"={"Start Test"=FALSE, "Toggle Spare 1"=FALSE, "Toggle Spare 2"=FALSE, "Toggle Spare 3"=FALSE, "Toggle Spare 4"=FALSE, "Toggle Spare 5"=FALSE}, "In Test"=FALSE, "HMI Command"=FALSE, "HMI Mom Buttons"={"Stop"=FALSE, "Reset Timers"=FALSE, "Log Fuel Change"=FALSE, "Alarm Dismiss"=FALSE}, "Controller Config"={"Controller Name"=enum."Kuhnke", "CommSeg"=0, "PWM?"=FALSE, "Frequency"=0, "Low Command"=0.0, "High Command"=0.0, "Stop Command"=0.0, "Command Step"=0.0, "Solenoid Stop?"=FALSE, "Controller?"=FALSE, "Invert PWM"=FALSE}, "Alarm"=FALSE, "Alarm Message 1"="", "Alarm Message 2"="", "Recording"=FALSE, "Serial Numbers"=[], "Pumps Present"=[]}  # HMI
  w19 = T24 {"PS Actual (V):"=0.0, "Temp1"=0.0, "Temp2"=0.0}  # Tank Data
  w20 = FALSE  # Recording
  w21 = ""  # Time/Date
  w22 = ""  # Alarm Message 2
  w23 = FALSE  # Alarm Latch
  w24 = T18 {"Voltages"=[0.015201568603515625, 0.00335693359375, 0.003021240234375, 0.12260055541992188, 0.06085968017578125, 0.052234649658203125], "PumpCurrent"=[0.015201568603515625, 0.00335693359375, 0.003021240234375, 0.12260055541992188, 0.06085968017578125, 0.052234649658203125], "Speed"=[0.0, 0.0, 0.0, 0.0, 0.0, 0.0], "ControllerCurrent"=[0.015201568603515625, 0.00335693359375, 0.003021240234375, 0.12260055541992188, 0.06085968017578125, 0.052234649658203125], "Pressure"=[0.015201568603515625, 0.00335693359375, 0.003021240234375, 0.12260055541992188, 0.06085968017578125, 0.052234649658203125], "Flow"=[0.0, 0.0, 0.0, 0.125, 0.0625, 0.0625], "Elapsed Time (Display)"=[7.1, 7.1, 7.1, 458133.45, 458138.85000000003, 458126.75], "Avg Pressure"=0.0, "Avg Speed"=0.0, "Elapsed Time"=[]}  # Pump Data
  w25 = path ""  # Fuel Log Path
  w26 = T23 {"Controller Name"=enum."Kuhnke", "CommSeg"=0, "PWM?"=FALSE, "Frequency"=0, "Low Command"=0.0, "High Command"=0.0, "Stop Command"=0.0, "Command Step"=0.0, "Solenoid Stop?"=FALSE, "Controller?"=FALSE, "Invert PWM"=FALSE}  # Controller Config
  w27 = T20 {"PS CMD"=0.0, "Press CMD"=0.0, "Temp 1 CMD"=0.0, "Temp 2 CMD"=0.0}  # Tank CMDs
  w28 = dbl[][] []  # CalArray
  w29 = u32[] []  # Prev ON Times
  w30 = ""  # Alarm Message 1
  w31 = u32[] []  # Previous Times
  w32 = i32[] []  # Trip Counters
  w33 = path ""  # Alarm Config Path
  w34 = T10 {"Alarms:"=[{"Description:"="", "Enabled:"=FALSE, "Data Index:"=0, "Data Type:"="", "Low Limit:"=0.0, "High Limit:"=0.0, "Trip Time:"=0, "Profile Sync:"=FALSE}, {"Description:"="", "Enabled:"=FALSE, "Data Index:"=0, "Data Type:"="", "Low Limit:"=0.0, "High Limit:"=0.0, "Trip Time:"=0, "Profile Sync:"=FALSE}, {"Description:"="", "Enabled:"=FALSE, "Data Index:"=0, "Data Type:"="", "Low Limit:"=0.0, "High Limit:"=0.0, "Trip Time:"=0, "Profile Sync:"=FALSE}, {"Description:"="", "Enabled:"=FALSE, "Data Index:"=0, "Data Type:"="", "Low Limit:"=0.0, "High Limit:"=0.0, "Trip Time:"=0, "Profile Sync:"=FALSE}, {"Description:"="", "Enabled:"=FALSE, "Data Index:"=0, "Data Type:"="", "Low Limit:"=0.0, "High Limit:"=0.0, "Trip Time:"=0, "Profile Sync:"=FALSE}, {"Description:"="", "Enabled:"=FALSE, "Data Index:"=0, "Data Type:"="", "Low Limit:"=0.0, "High Limit:"=0.0, "Trip Time:"=0, "Profile Sync:"=FALSE}, {"Description:"="", "Enabled:"=FALSE, "Data Index:"=0, "Data Type:"="", "Low Limit:"=0.0, "High Limit:"=0.0, "Trip Time:"=0, "Profile Sync:"=FALSE}, {"Description:"="", "Enabled:"=FALSE, "Data Index:"=0, "Data Type:"="", "Low Limit:"=0.0, "High Limit:"=0.0, "Trip Time:"=0, "Profile Sync:"=FALSE}], "Profile Sync:"={"Trip Time:"=0, "Consecutive Trips:"=0}}  # Alarm Config
  w35 = T25 []  # Controller List
  w36 = T8 {"Pump 1"=FALSE, "Pump 2"=FALSE, "Pump 3"=FALSE, "Pump 4"=FALSE, "Pump 5"=FALSE, "Pump 6"=FALSE}  # Ignition Relay
  w37 = T8 {"Pump 1"=FALSE, "Pump 2"=FALSE, "Pump 3"=FALSE, "Pump 4"=FALSE, "Pump 5"=FALSE, "Pump 6"=FALSE}  # Power Relay
  w38 = FALSE  # Voltage Enable
  w39 = u32 0  # Inputs Timer
  w40 = dbl[] [0.0, 0.0, 0.0, 0.0, 0.0, 0.0]  # Pressure Offsets
  w42 = FALSE  # New Step
  w43 = 0  # Stagger Counter
  w44 = FALSE  # Login
  w45 = dbl[] [0.0, 0.0, 0.0, 0.0, 0.0, 0.0]  # Initial Times
  w46 = bool[] [FALSE, FALSE, FALSE, FALSE, FALSE, FALSE]  # pb.Sets
  w47 = bool[] [FALSE, FALSE, FALSE, FALSE, FALSE, FALSE]  # pb.Resets
  w48 = FALSE  # pb.Run Profile
  w49 = FALSE  # Client?
  w50 = dbl[] [0.0, 0.0, 0.0, 0.0, 0.0, 0.0]  # Controller CMDs
  w51 = 0.0  # Last Profile Time
  w52 = u32 0  # Screen Timer
  w53 = 0  # # of Steps
  w54 = 0.0  # Step Time
  w55 = 0.0  # Step Start Time
  w56 = FALSE  # Run Profile
  w58 = 0  # Current Step
  w57 = 0.0  # Step Time Left
  w59 = string[] []  # Profiles
  w61 = string[][] []  # Profile
  w62 = errorcluster {"status"=FALSE, "code"=0, "source"=""}  # Error
  n1 = Bundle("Error"=w62, "Profile"=w61, "App Config"="App Config", "Profiles"=w59, "Current Step"=w58, "Step Time Left"=w57, "Run Profile"=w56, "Step Start Time"=w55, "Step Time"=w54, "# of Steps"=w53, "Screen Timer"=w52, "Last Profile Time"=w51, "Controller CMDs"=w50, "Client?"=w49, "pb.Run Profile"=w48, "pb.Resets"=w47, "pb.Sets"=w46, "Initial Times"=w45, "Pressure Offsets"=w40, "Login"=w44, "Stagger Counter"=w43, "New Step"=w42, "Inputs Timer"=w39, "Tank Data"=w19, "Voltage Enable"=w38, "Power Relay"=w37, "Ignition Relay"=w36, "Controller List"=w35, "Alarm Config"=w34, "Alarm Config Path"=w33, "Trip Counters"=w32, "Previous Times"=w31, "Alarm Message 1"=w30, "Alarm Message 2"=w22, "Prev ON Times"=w29, "CalArray"=w28, "Tank CMDs"=w27, "Controller Config"=w26, "Fuel Log Path"=w25, "Pump Data"=w24, "Alarm Latch"=w23, "Time/Date"=w21, "Recording"=w20, "HMI"=w18, "WebDAV Push"=w17, "Email Alarms Disabled"=w16, "Concat Data"=w15, "LS Data"=w14, "Main Tab"=w13, "LS App Config"=w1, "Bank 1 State:"=w12, "Bank 2 State:"=w11, "LS Data Filepath"=w10, "Initial LS Data"=w9, "day of month"=w2) -> (w41:T26)  [unwired: 1 in]
  n2 = xnode "Open FPGA VI Reference"("resource name"=tag "RIO0") -> ("FPGA VI Reference Out"=w3:T27, "error out"=w7:errorcluster)  [unwired: 1 in]
  n3 = Generate Occurrence() -> (w5:refnum<k4>)
  n4 = Wait on Occurrence(2:w5) -> (0:w4:bool)  [unwired: 2 in]
  n5 = while {
    shift-right: [w71] -> _
    shift-left: w8 -> [w69]
    shift-right: [w72] -> _
    shift-left: w41 -> [w73]
    tunnel: w3 -> [w70]
    tunnel: w5 -> [w64]
    tunnel: w7 -> [_]
    stop <- FALSE stop-if-true
    n6 = Delete From Array(array=w69, length=1, index=0 ("length")) -> (deleted portion=w65:T15[], array with subset deleted=w68:T15[])
    n7 = Index Array(array=w65) -> (element=w63:T15)  [unwired: 1 in]
    n8 = case shown="\"Main\", Default" w63 {
      selector: w63 -> [_ _ _ _ _ _ _ _ _ _ _ _ _ _ _ _ _ _ _ _ _ _ _ _ _ w1529 _ _ _ _ _ _ _ _ _ w1787 _ _ _ _ _ _ _ _ _ _ _ _ _]
      tunnel: [w79 w689 w821 w859 w866 w888 w908 w916 w931 w945 w980 w1018 w1066 w1128 w1222 w1280 w1341 w1376 w1400 w1421 w1445 w1474 w1504 w1512 w1517 w1532 w1604 w1630 w1642 w1679 w1691 w1702 w1705 w1715 w1772 w1792 w1810 w1824 w1833 w1842 w1850 w1855 w1872 w1900 w1945 w1959 w2018 w2025 w2033] -> w72
      tunnel: w73 -> [w98 w690 w820 w859 w867 w889 w908 w917 w932 w946 w958 w1019 w1067 w1129 w1247 w1281 w1341 w1376 w1406 w1422 w1445 w1474 w1504 w1512 w1517 w1530 w1604 w1631 w1641 w1677 w1691 w1702 w1705 w1716 w1772 w1792 w1809 w1824 w1833 w1842 w1850 w1856 w1873 w1901 w1945 w1959 w2019 w2025 w2033]
      tunnel: [w92 w673 w804 w858 w863 w892 w909 w910 w921 w941 w973 w996 w1045 w1115 w1217 w1305 w1354 w1372 w1409 w1416 w1446 w1473 w1505 w1511 w1515 w1527 w1610 w1632 w1636 w1673 w1690 w1701 w1706 w1713 w1771 w1793 w1813 w1825 w1834 w1841 w1845 w1864 w1869 w1902 w1944 w1955 w2017 w2026 w2038] -> w71
      tunnel: w70 -> [_ _ w758 _ _ _ _ _ _ _ _ _ _ w1086 w1198 _ _ _ _ _ _ _ _ _ w1516 w1531 _ _ w1640 w1678 _ _ _ w1717 _ _ _ _ _ w1836 _ _ _ _ _ _ _ _ _]
      tunnel: w68 -> [w86 w671 w807 w858 w862 w892 w909 w911 w922 w941 w974 w1000 w1062 w1116 w1232 w1304 w1353 w1373 w1410 w1417 w1446 w1473 w1505 w1511 w1515 w1528 w1611 w1633 w1637 w1672 w1690 w1701 w1707 w1714 w1771 w1793 w1814 w1825 w1834 w1841 w1846 w1865 w1881 w1902 w1944 w1955 w2017 w2026 w2039]
      tunnel: w64 -> [_ _ w816 _ _ _ _ _ _ _ _ _ _ _ _ _ _ _ _ _ _ _ _ _ _ _ _ _ _ _ _ _ _ _ _ _ _ _ _ _ _ _ _ _ _ _ _ _ _]
      frame "Main", Default {
        (unwired) T15[] [enum."Update Screen", enum."Save LS Data"] items=["Main", "Init Files", "Init", "Unused", "Save As", "Start Profile", "Check Step Time", "Alarm", "Alarm Dismiss", "Run Step", "Stop Profile", "Cycle Reset", "Time Reset", "Time Reset All", "Time Set", "Tare CTs", "Save Profile", "Open Profile", "Get Profiles", "Update Screen", "Update Controls", "Save App Config", "Write Outputs", "Disable Background", "Enable Background", "Get/Release Control", "Log Fuel Change", "Fuel Change Popup", "Read Inputs", "Remote Timer Reset", "Controller Change", "Get Alarms", "Init Alarms", "Save Alarms", "Voltage Selection", "Set Watlow Temp 1", "Set Watlow Temp 2", "Get Pressure", "Write Tare Pressure", "Adjust Controls", "Reinit ADC", "Write Initial Times", "Write Pumps Present", "HMI Command", "Save Pump Times", "Check Pump Stop Time", "Save LS App Config", "Init Data File", "Reset LS Cycles", "Reset Anomalies", "Reset Opens", "Save LS Data", "Save LS Test Data", "Check Serial Numbers", "Main Tab", "Allow Data Note"]
        n9 = Unbundle By Name(w98) -> ("Run Profile"=w78:bool, "Inputs Timer"=w85:u32, "Screen Timer"=w84:u32)
        n10 = Wait (ms)(milliseconds to wait=u32 10) -> ()  [unwired: 1 out]
        n11 = for {
          N: 75 -> [_]
          shift-right: [w123] -> w79
          shift-left: w98 -> [w122]
          tunnel: [w121] -> w94
          tunnel: [w120] -> w93
          i -> [w119]
          stop <- w120 stop-if-true
          n12 = case shown="58" w119 {
            tunnel: w122 -> [w130 w132 w134 w143 w148 w154 w162 w169 w177 w184 w192 w200 w208 w215 w218 w219 w227 w235 w242 w250 w251 w259 w266 w273 w281 w285 w291 w307 w315 w322 w326 w329 w336 w345 w354 w363 w372 w381 w390 w399 w407 w414 w421 w428 w431 w438 w444 w449 w456 w463 w470 w477 w491 w499 w506 w515 w524 w531 w538 w545 w552 w559 w566 w580 w587 w594 w597 w600 w603 w611 w618 w625 w631 w638]
            tunnel: [w129 w132 w134 w142 w148 w154 w161 w168 w176 w183 w191 w199 w207 w214 w218 w219 w226 w234 w241 w249 w251 w258 w265 w272 w280 w284 w290 w306 w314 w321 w326 w329 w335 w344 w353 w362 w371 w380 w389 w398 w406 w413 w420 w427 w431 w437 w443 w448 w455 w462 w469 w476 w490 w498 w505 w514 w523 w530 w537 w544 w551 w558 w565 w579 w586 w593 w597 w600 w603 w610 w617 w624 w631 w637] -> w123
            tunnel: w122 -> [w128 _ _ w141 w146 _ w159 w166 w175 w182 w190 w198 w206 w213 _ _ w224 w232 w239 w248 _ w257 w264 w271 w279 w286 w293 w308 w316 w323 _ _ w337 w346 w355 w364 w373 w382 w391 w400 w408 w415 w419 w426 _ w439 _ _ w454 w461 w468 w475 w492 w500 w507 w516 w525 w532 w539 w546 w553 w560 w567 w581 w588 w595 _ _ _ w609 w619 w626 _ w636]
            tunnel: [w127 w133 w135 w140 w144 w156 w157 w164 w172 w178 w189 w196 w202 w210 w217 w221 w223 w231 w238 w247 w253 w260 w267 w274 w278 w288 w298 w310 w317 w324 w327 w330 w332 w342 w347 w356 w365 w374 w383 w396 w404 w411 w422 w429 w433 w440 w445 w450 w457 w464 w471 w478 w487 w497 w504 w513 w522 w529 w536 w543 w550 w557 w564 w578 w585 w592 w598 w601 w604 w606 w614 w621 w629 w632] -> w121
            tunnel: [w124 "pb.E Stop" "pb.Save As" w137 "pb.Stop Profile" "pb.Cycle Reset" w160 w167 w173 w180 w185 w194 w204 w211 FALSE ("pb.Tare Pressure") "pb.Time Reset All" w225 w233 w240 w244 "pb.FuelChange" w254 w263 w268 w275 w287 w294 w309 w311 w318 "pb.Alarm OK" "pb.Tare Pressure" w333 w338 w348 w358 w367 w375 w385 w393 w403 w409 w417 w424 w430 w434 FALSE ("HMI Command") FALSE ("HMI Command") w453 w460 w467 w474 w486 w494 w502 w508 w518 w527 w534 w541 w548 w555 w562 w573 w582 w590 "Reset Total Cycles" "Reset Anomalies" "Reset Opens" w607 w616 w623 FALSE ("Reset Opens") w635] -> w120
            frame 0, Default {
              w127 = T15[] [enum."Write Outputs"] items=["Main", "Init Files", "Init", "Unused", "Save As", "Start Profile", "Check Step Time", "Alarm", "Alarm Dismiss", "Run Step", "Stop Profile", "Cycle Reset", "Time Reset", "Time Reset All", "Time Set", "Tare CTs", "Save Profile", "Open Profile", "Get Profiles", "Update Screen", "Update Controls", "Save App Config", "Write Outputs", "Disable Background", "Enable Background", "Get/Release Control", "Log Fuel Change", "Fuel Change Popup", "Read Inputs", "Remote Timer Reset", "Controller Change", "Get Alarms", "Init Alarms", "Save Alarms", "Voltage Selection", "Set Watlow Temp 1", "Set Watlow Temp 2", "Get Pressure", "Write Tare Pressure", "Adjust Controls", "Reinit ADC", "Write Initial Times", "Write Pumps Present", "HMI Command", "Save Pump Times", "Check Pump Stop Time", "Save LS App Config", "Init Data File", "Reset LS Cycles", "Reset Anomalies", "Reset Opens", "Save LS Data", "Save LS Test Data", "Check Serial Numbers", "Main Tab", "Allow Data Note"]
              n13 = Unbundle By Name(w128) -> ("Tank CMDs.PS CMD"=w126:dbl)
              n14 = Not Equal?(x=w126, y="Power Supply Cmd:") -> (x != y?=w124:bool)
              n15 = Bundle By Name(cluster=w130, "Tank CMDs.PS CMD"="Power Supply Cmd:") -> (w129:T26)
            }
            frame 1 {
              w133 = T15[] [enum."Stop Profile"] items=["Main", "Init Files", "Init", "Unused", "Save As", "Start Profile", "Check Step Time", "Alarm", "Alarm Dismiss", "Run Step", "Stop Profile", "Cycle Reset", "Time Reset", "Time Reset All", "Time Set", "Tare CTs", "Save Profile", "Open Profile", "Get Profiles", "Update Screen", "Update Controls", "Save App Config", "Write Outputs", "Disable Background", "Enable Background", "Get/Release Control", "Log Fuel Change", "Fuel Change Popup", "Read Inputs", "Remote Timer Reset", "Controller Change", "Get Alarms", "Init Alarms", "Save Alarms", "Voltage Selection", "Set Watlow Temp 1", "Set Watlow Temp 2", "Get Pressure", "Write Tare Pressure", "Adjust Controls", "Reinit ADC", "Write Initial Times", "Write Pumps Present", "HMI Command", "Save Pump Times", "Check Pump Stop Time", "Save LS App Config", "Init Data File", "Reset LS Cycles", "Reset Anomalies", "Reset Opens", "Save LS Data", "Save LS Test Data", "Check Serial Numbers", "Main Tab", "Allow Data Note"]
            }
            frame 2 {
              w135 = T15[] [enum."Disable Background", enum."Save As"] items=["Main", "Init Files", "Init", "Unused", "Save As", "Start Profile", "Check Step Time", "Alarm", "Alarm Dismiss", "Run Step", "Stop Profile", "Cycle Reset", "Time Reset", "Time Reset All", "Time Set", "Tare CTs", "Save Profile", "Open Profile", "Get Profiles", "Update Screen", "Update Controls", "Save App Config", "Write Outputs", "Disable Background", "Enable Background", "Get/Release Control", "Log Fuel Change", "Fuel Change Popup", "Read Inputs", "Remote Timer Reset", "Controller Change", "Get Alarms", "Init Alarms", "Save Alarms", "Voltage Selection", "Set Watlow Temp 1", "Set Watlow Temp 2", "Get Pressure", "Write Tare Pressure", "Adjust Controls", "Reinit ADC", "Write Initial Times", "Write Pumps Present", "HMI Command", "Save Pump Times", "Check Pump Stop Time", "Save LS App Config", "Init Data File", "Reset LS Cycles", "Reset Anomalies", "Reset Opens", "Save LS Data", "Save LS Test Data", "Check Serial Numbers", "Main Tab", "Allow Data Note"]
            }
            frame 3 {
              w140 = T15[] [enum."Voltage Selection", enum."Start Profile"] items=["Main", "Init Files", "Init", "Unused", "Save As", "Start Profile", "Check Step Time", "Alarm", "Alarm Dismiss", "Run Step", "Stop Profile", "Cycle Reset", "Time Reset", "Time Reset All", "Time Set", "Tare CTs", "Save Profile", "Open Profile", "Get Profiles", "Update Screen", "Update Controls", "Save App Config", "Write Outputs", "Disable Background", "Enable Background", "Get/Release Control", "Log Fuel Change", "Fuel Change Popup", "Read Inputs", "Remote Timer Reset", "Controller Change", "Get Alarms", "Init Alarms", "Save Alarms", "Voltage Selection", "Set Watlow Temp 1", "Set Watlow Temp 2", "Get Pressure", "Write Tare Pressure", "Adjust Controls", "Reinit ADC", "Write Initial Times", "Write Pumps Present", "HMI Command", "Save Pump Times", "Check Pump Stop Time", "Save LS App Config", "Init Data File", "Reset LS Cycles", "Reset Anomalies", "Reset Opens", "Save LS Data", "Save LS Test Data", "Check Serial Numbers", "Main Tab", "Allow Data Note"]
              n16 = Unbundle By Name(w141) -> ("pb.Run Profile"=w139:bool)
              n17 = Greater?(x="pb.Run Profile", y=w139) -> (0:w137:bool)
              n18 = Bundle By Name(cluster=w143, "pb.Run Profile"="pb.Run Profile") -> (w142:T26)
            }
            frame 4 {
              n19 = Unbundle By Name(w146) -> ("pb.Run Profile"=w145:bool)
              n20 = disable-structure shown="Enabled" {
                disable-tunnel: w145 -> [_ w153]
                disable-tunnel: [w149 w151] -> w144
                frame Enabled {
                  w149 = T15[] [enum."Stop Profile", enum."Save LS Test Data"] items=["Main", "Init Files", "Init", "Unused", "Save As", "Start Profile", "Check Step Time", "Alarm", "Alarm Dismiss", "Run Step", "Stop Profile", "Cycle Reset", "Time Reset", "Time Reset All", "Time Set", "Tare CTs", "Save Profile", "Open Profile", "Get Profiles", "Update Screen", "Update Controls", "Save App Config", "Write Outputs", "Disable Background", "Enable Background", "Get/Release Control", "Log Fuel Change", "Fuel Change Popup", "Read Inputs", "Remote Timer Reset", "Controller Change", "Get Alarms", "Init Alarms", "Save Alarms", "Voltage Selection", "Set Watlow Temp 1", "Set Watlow Temp 2", "Get Pressure", "Write Tare Pressure", "Adjust Controls", "Reinit ADC", "Write Initial Times", "Write Pumps Present", "HMI Command", "Save Pump Times", "Check Pump Stop Time", "Save LS App Config", "Init Data File", "Reset LS Cycles", "Reset Anomalies", "Reset Opens", "Save LS Data", "Save LS Test Data", "Check Serial Numbers", "Main Tab", "Allow Data Note"]
                }
                frame Disabled {
                  w150 = T15[] [enum."Stop Profile", enum."Save LS Test Data"] items=["Main", "Init Files", "Init", "Unused", "Save As", "Start Profile", "Check Step Time", "Alarm", "Alarm Dismiss", "Run Step", "Stop Profile", "Cycle Reset", "Time Reset", "Time Reset All", "Time Set", "Tare CTs", "Save Profile", "Open Profile", "Get Profiles", "Update Screen", "Update Controls", "Save App Config", "Write Outputs", "Disable Background", "Enable Background", "Get/Release Control", "Log Fuel Change", "Fuel Change Popup", "Read Inputs", "Remote Timer Reset", "Controller Change", "Get Alarms", "Init Alarms", "Save Alarms", "Voltage Selection", "Set Watlow Temp 1", "Set Watlow Temp 2", "Get Pressure", "Write Tare Pressure", "Adjust Controls", "Reinit ADC", "Write Initial Times", "Write Pumps Present", "HMI Command", "Save Pump Times", "Check Pump Stop Time", "Save LS App Config", "Init Data File", "Reset LS Cycles", "Reset Anomalies", "Reset Opens", "Save LS Data", "Save LS Test Data", "Check Serial Numbers", "Main Tab", "Allow Data Note"]
                  w152 = T15[] [enum."Stop Profile", enum."Save LS Test Data", enum."Allow Data Note"] items=["Main", "Init Files", "Init", "Unused", "Save As", "Start Profile", "Check Step Time", "Alarm", "Alarm Dismiss", "Run Step", "Stop Profile", "Cycle Reset", "Time Reset", "Time Reset All", "Time Set", "Tare CTs", "Save Profile", "Open Profile", "Get Profiles", "Update Screen", "Update Controls", "Save App Config", "Write Outputs", "Disable Background", "Enable Background", "Get/Release Control", "Log Fuel Change", "Fuel Change Popup", "Read Inputs", "Remote Timer Reset", "Controller Change", "Get Alarms", "Init Alarms", "Save Alarms", "Voltage Selection", "Set Watlow Temp 1", "Set Watlow Temp 2", "Get Pressure", "Write Tare Pressure", "Adjust Controls", "Reinit ADC", "Write Initial Times", "Write Pumps Present", "HMI Command", "Save Pump Times", "Check Pump Stop Time", "Save LS App Config", "Init Data File", "Reset LS Cycles", "Reset Anomalies", "Reset Opens", "Save LS Data", "Save LS Test Data", "Check Serial Numbers", "Main Tab", "Allow Data Note"]
                  n21 = Select(t=w152, s=w153, f=w150) -> (s? t:f=w151:T15[])
                }
              }
            }
            frame 5 {
              w156 = T15[] [enum."Disable Background", enum."Cycle Reset"] items=["Main", "Init Files", "Init", "Unused", "Save As", "Start Profile", "Check Step Time", "Alarm", "Alarm Dismiss", "Run Step", "Stop Profile", "Cycle Reset", "Time Reset", "Time Reset All", "Time Set", "Tare CTs", "Save Profile", "Open Profile", "Get Profiles", "Update Screen", "Update Controls", "Save App Config", "Write Outputs", "Disable Background", "Enable Background", "Get/Release Control", "Log Fuel Change", "Fuel Change Popup", "Read Inputs", "Remote Timer Reset", "Controller Change", "Get Alarms", "Init Alarms", "Save Alarms", "Voltage Selection", "Set Watlow Temp 1", "Set Watlow Temp 2", "Get Pressure", "Write Tare Pressure", "Adjust Controls", "Reinit ADC", "Write Initial Times", "Write Pumps Present", "HMI Command", "Save Pump Times", "Check Pump Stop Time", "Save LS App Config", "Init Data File", "Reset LS Cycles", "Reset Anomalies", "Reset Opens", "Save LS Data", "Save LS Test Data", "Check Serial Numbers", "Main Tab", "Allow Data Note"]
            }
            frame 6 {
              w157 = T15[] [enum."Disable Background", enum."Time Reset", enum."Update Controls"] items=["Main", "Init Files", "Init", "Unused", "Save As", "Start Profile", "Check Step Time", "Alarm", "Alarm Dismiss", "Run Step", "Stop Profile", "Cycle Reset", "Time Reset", "Time Reset All", "Time Set", "Tare CTs", "Save Profile", "Open Profile", "Get Profiles", "Update Screen", "Update Controls", "Save App Config", "Write Outputs", "Disable Background", "Enable Background", "Get/Release Control", "Log Fuel Change", "Fuel Change Popup", "Read Inputs", "Remote Timer Reset", "Controller Change", "Get Alarms", "Init Alarms", "Save Alarms", "Voltage Selection", "Set Watlow Temp 1", "Set Watlow Temp 2", "Get Pressure", "Write Tare Pressure", "Adjust Controls", "Reinit ADC", "Write Initial Times", "Write Pumps Present", "HMI Command", "Save Pump Times", "Check Pump Stop Time", "Save LS App Config", "Init Data File", "Reset LS Cycles", "Reset Anomalies", "Reset Opens", "Save LS Data", "Save LS Test Data", "Check Serial Numbers", "Main Tab", "Allow Data Note"]
              n22 = Unbundle By Name(w159) -> ("pb.Resets"=w163:bool[])
              n23 = Greater?(x="pb.Resets", y=w163) -> (0:w160:bool)
              n24 = Bundle By Name(cluster=w162, "pb.Resets"="pb.Resets") -> (w161:T26)
            }
            frame 7 {
              w164 = T15[] [enum."Disable Background", enum."Time Set", enum."Update Controls"] items=["Main", "Init Files", "Init", "Unused", "Save As", "Start Profile", "Check Step Time", "Alarm", "Alarm Dismiss", "Run Step", "Stop Profile", "Cycle Reset", "Time Reset", "Time Reset All", "Time Set", "Tare CTs", "Save Profile", "Open Profile", "Get Profiles", "Update Screen", "Update Controls", "Save App Config", "Write Outputs", "Disable Background", "Enable Background", "Get/Release Control", "Log Fuel Change", "Fuel Change Popup", "Read Inputs", "Remote Timer Reset", "Controller Change", "Get Alarms", "Init Alarms", "Save Alarms", "Voltage Selection", "Set Watlow Temp 1", "Set Watlow Temp 2", "Get Pressure", "Write Tare Pressure", "Adjust Controls", "Reinit ADC", "Write Initial Times", "Write Pumps Present", "HMI Command", "Save Pump Times", "Check Pump Stop Time", "Save LS App Config", "Init Data File", "Reset LS Cycles", "Reset Anomalies", "Reset Opens", "Save LS Data", "Save LS Test Data", "Check Serial Numbers", "Main Tab", "Allow Data Note"]
              n25 = Unbundle By Name(w166) -> ("pb.Sets"=w170:bool[])
              n26 = Greater?(x="pb.Sets", y=w170) -> (0:w167:bool)
              n27 = Bundle By Name(cluster=w169, "pb.Sets"="pb.Sets") -> (w168:T26)
            }
            frame 8 {
              w172 = T15[] [enum."Save Profile", enum."Update Controls"] items=["Main", "Init Files", "Init", "Unused", "Save As", "Start Profile", "Check Step Time", "Alarm", "Alarm Dismiss", "Run Step", "Stop Profile", "Cycle Reset", "Time Reset", "Time Reset All", "Time Set", "Tare CTs", "Save Profile", "Open Profile", "Get Profiles", "Update Screen", "Update Controls", "Save App Config", "Write Outputs", "Disable Background", "Enable Background", "Get/Release Control", "Log Fuel Change", "Fuel Change Popup", "Read Inputs", "Remote Timer Reset", "Controller Change", "Get Alarms", "Init Alarms", "Save Alarms", "Voltage Selection", "Set Watlow Temp 1", "Set Watlow Temp 2", "Get Pressure", "Write Tare Pressure", "Adjust Controls", "Reinit ADC", "Write Initial Times", "Write Pumps Present", "HMI Command", "Save Pump Times", "Check Pump Stop Time", "Save LS App Config", "Init Data File", "Reset LS Cycles", "Reset Anomalies", "Reset Opens", "Save LS Data", "Save LS Test Data", "Check Serial Numbers", "Main Tab", "Allow Data Note"]
              n28 = Unbundle By Name(w175) -> ("Profile"=w174:string[][])
              n29 = Not Equal?(x=w174, y="Profile:") -> (x != y?=w173:bool)
              n30 = Bundle By Name(cluster=w177, "Profile"="Profile:") -> (w176:T26)
            }
            frame 9 {
              w178 = T15[] [enum."Open Profile", enum."Update Controls"] items=["Main", "Init Files", "Init", "Unused", "Save As", "Start Profile", "Check Step Time", "Alarm", "Alarm Dismiss", "Run Step", "Stop Profile", "Cycle Reset", "Time Reset", "Time Reset All", "Time Set", "Tare CTs", "Save Profile", "Open Profile", "Get Profiles", "Update Screen", "Update Controls", "Save App Config", "Write Outputs", "Disable Background", "Enable Background", "Get/Release Control", "Log Fuel Change", "Fuel Change Popup", "Read Inputs", "Remote Timer Reset", "Controller Change", "Get Alarms", "Init Alarms", "Save Alarms", "Voltage Selection", "Set Watlow Temp 1", "Set Watlow Temp 2", "Get Pressure", "Write Tare Pressure", "Adjust Controls", "Reinit ADC", "Write Initial Times", "Write Pumps Present", "HMI Command", "Save Pump Times", "Check Pump Stop Time", "Save LS App Config", "Init Data File", "Reset LS Cycles", "Reset Anomalies", "Reset Opens", "Save LS Data", "Save LS Test Data", "Check Serial Numbers", "Main Tab", "Allow Data Note"]
              n31 = Unbundle By Name(w182) -> ("App Config.Current Profile"=w181:string)
              n32 = Not Equal?(x=w181, y="Profile Name:") -> (x != y?=w180:bool)
              n33 = Bundle By Name(cluster=w184, "App Config.Current Profile"="Profile Name:") -> (w183:T26)
            }
            frame 10 {
              w189 = T15[] [enum."Write Outputs"] items=["Main", "Init Files", "Init", "Unused", "Save As", "Start Profile", "Check Step Time", "Alarm", "Alarm Dismiss", "Run Step", "Stop Profile", "Cycle Reset", "Time Reset", "Time Reset All", "Time Set", "Tare CTs", "Save Profile", "Open Profile", "Get Profiles", "Update Screen", "Update Controls", "Save App Config", "Write Outputs", "Disable Background", "Enable Background", "Get/Release Control", "Log Fuel Change", "Fuel Change Popup", "Read Inputs", "Remote Timer Reset", "Controller Change", "Get Alarms", "Init Alarms", "Save Alarms", "Voltage Selection", "Set Watlow Temp 1", "Set Watlow Temp 2", "Get Pressure", "Write Tare Pressure", "Adjust Controls", "Reinit ADC", "Write Initial Times", "Write Pumps Present", "HMI Command", "Save Pump Times", "Check Pump Stop Time", "Save LS App Config", "Init Data File", "Reset LS Cycles", "Reset Anomalies", "Reset Opens", "Save LS Data", "Save LS Test Data", "Check Serial Numbers", "Main Tab", "Allow Data Note"]
              n34 = Unbundle By Name(w190) -> ("Controller CMDs"=w188:dbl[])
              n35 = Not Equal?(x="Controller\nCMD", y=w188) -> (x != y?=w186:bool[])
              n36 = Or Array Elements(Boolean array=w186) -> (logical OR=w185:bool)
              n37 = Bundle By Name(cluster=w192, "Controller CMDs"="Controller\nCMD") -> (w191:T26)
            }
            frame 11 {
              w196 = T15[] [enum."Get/Release Control"] items=["Main", "Init Files", "Init", "Unused", "Save As", "Start Profile", "Check Step Time", "Alarm", "Alarm Dismiss", "Run Step", "Stop Profile", "Cycle Reset", "Time Reset", "Time Reset All", "Time Set", "Tare CTs", "Save Profile", "Open Profile", "Get Profiles", "Update Screen", "Update Controls", "Save App Config", "Write Outputs", "Disable Background", "Enable Background", "Get/Release Control", "Log Fuel Change", "Fuel Change Popup", "Read Inputs", "Remote Timer Reset", "Controller Change", "Get Alarms", "Init Alarms", "Save Alarms", "Voltage Selection", "Set Watlow Temp 1", "Set Watlow Temp 2", "Get Pressure", "Write Tare Pressure", "Adjust Controls", "Reinit ADC", "Write Initial Times", "Write Pumps Present", "HMI Command", "Save Pump Times", "Check Pump Stop Time", "Save LS App Config", "Init Data File", "Reset LS Cycles", "Reset Anomalies", "Reset Opens", "Save LS Data", "Save LS Test Data", "Check Serial Numbers", "Main Tab", "Allow Data Note"]
              n38 = Unbundle By Name(w198) -> ("Client?"=w195:bool, "Profiles"=w197:string[])
              n39 = call "App Global.vi"() -> ("Client? OUT"=w193:bool)  [unwired: 9 in, 2 out]
              n40 = Greater?(x=w193, y=w195) -> (0:w194:bool)
              n41 = case shown="True" w194 {
                tunnel: w197 -> [_ w201]
                frame False {
                }
                frame True {
                  n42 = property on="Profile Name:" class="CmbBox"("Strings[]"=w201) -> ()  [unwired: 2 in, 2 out]
                }
              }
              n43 = Bundle By Name(cluster=w200, "Client?"=w193) -> (w199:T26)
            }
            frame 13 {
              w202 = T15[] [enum."Init Data File", enum."Save LS App Config", enum."Save App Config"] items=["Main", "Init Files", "Init", "Unused", "Save As", "Start Profile", "Check Step Time", "Alarm", "Alarm Dismiss", "Run Step", "Stop Profile", "Cycle Reset", "Time Reset", "Time Reset All", "Time Set", "Tare CTs", "Save Profile", "Open Profile", "Get Profiles", "Update Screen", "Update Controls", "Save App Config", "Write Outputs", "Disable Background", "Enable Background", "Get/Release Control", "Log Fuel Change", "Fuel Change Popup", "Read Inputs", "Remote Timer Reset", "Controller Change", "Get Alarms", "Init Alarms", "Save Alarms", "Voltage Selection", "Set Watlow Temp 1", "Set Watlow Temp 2", "Get Pressure", "Write Tare Pressure", "Adjust Controls", "Reinit ADC", "Write Initial Times", "Write Pumps Present", "HMI Command", "Save Pump Times", "Check Pump Stop Time", "Save LS App Config", "Init Data File", "Reset LS Cycles", "Reset Anomalies", "Reset Opens", "Save LS Data", "Save LS Test Data", "Check Serial Numbers", "Main Tab", "Allow Data Note"]
              n44 = Unbundle By Name(w206) -> ("App Config.CA Number"=w205:string)
              n45 = Not Equal?(x=w205, y="CA Number:") -> (x != y?=w204:bool)
              n46 = Bundle By Name(cluster=w208, "App Config.CA Number"="CA Number:") -> (w207:T26)
            }
            frame 14 {
              w210 = T15[] [enum."Save App Config", enum."Controller Change", enum."Write Outputs"] items=["Main", "Init Files", "Init", "Unused", "Save As", "Start Profile", "Check Step Time", "Alarm", "Alarm Dismiss", "Run Step", "Stop Profile", "Cycle Reset", "Time Reset", "Time Reset All", "Time Set", "Tare CTs", "Save Profile", "Open Profile", "Get Profiles", "Update Screen", "Update Controls", "Save App Config", "Write Outputs", "Disable Background", "Enable Background", "Get/Release Control", "Log Fuel Change", "Fuel Change Popup", "Read Inputs", "Remote Timer Reset", "Controller Change", "Get Alarms", "Init Alarms", "Save Alarms", "Voltage Selection", "Set Watlow Temp 1", "Set Watlow Temp 2", "Get Pressure", "Write Tare Pressure", "Adjust Controls", "Reinit ADC", "Write Initial Times", "Write Pumps Present", "HMI Command", "Save Pump Times", "Check Pump Stop Time", "Save LS App Config", "Init Data File", "Reset LS Cycles", "Reset Anomalies", "Reset Opens", "Save LS Data", "Save LS Test Data", "Check Serial Numbers", "Main Tab", "Allow Data Note"]
              n47 = Unbundle By Name(w213) -> ("App Config.Controller Type:"=w212:T3)
              n48 = Not Equal?(x=w212, y="Controller Type:") -> (x != y?=w211:bool)
              n49 = Bundle By Name(cluster=w215, "App Config.Controller Type:"="Controller Type:") -> (w214:T26)
            }
            frame 15 {
              w217 = T15[] [] items=["Main", "Init Files", "Init", "Unused", "Save As", "Start Profile", "Check Step Time", "Alarm", "Alarm Dismiss", "Run Step", "Stop Profile", "Cycle Reset", "Time Reset", "Time Reset All", "Time Set", "Tare CTs", "Save Profile", "Open Profile", "Get Profiles", "Update Screen", "Update Controls", "Save App Config", "Write Outputs", "Disable Background", "Enable Background", "Get/Release Control", "Log Fuel Change", "Fuel Change Popup", "Read Inputs", "Remote Timer Reset", "Controller Change", "Get Alarms", "Init Alarms", "Save Alarms", "Voltage Selection", "Set Watlow Temp 1", "Set Watlow Temp 2", "Get Pressure", "Write Tare Pressure", "Adjust Controls", "Reinit ADC", "Write Initial Times", "Write Pumps Present", "HMI Command", "Save Pump Times", "Check Pump Stop Time", "Save LS App Config", "Init Data File", "Reset LS Cycles", "Reset Anomalies", "Reset Opens", "Save LS Data", "Save LS Test Data", "Check Serial Numbers", "Main Tab", "Allow Data Note"]
            }
            frame 16 {
              w221 = T15[] [enum."Disable Background", enum."Time Reset All", enum."Update Controls"] items=["Main", "Init Files", "Init", "Unused", "Save As", "Start Profile", "Check Step Time", "Alarm", "Alarm Dismiss", "Run Step", "Stop Profile", "Cycle Reset", "Time Reset", "Time Reset All", "Time Set", "Tare CTs", "Save Profile", "Open Profile", "Get Profiles", "Update Screen", "Update Controls", "Save App Config", "Write Outputs", "Disable Background", "Enable Background", "Get/Release Control", "Log Fuel Change", "Fuel Change Popup", "Read Inputs", "Remote Timer Reset", "Controller Change", "Get Alarms", "Init Alarms", "Save Alarms", "Voltage Selection", "Set Watlow Temp 1", "Set Watlow Temp 2", "Get Pressure", "Write Tare Pressure", "Adjust Controls", "Reinit ADC", "Write Initial Times", "Write Pumps Present", "HMI Command", "Save Pump Times", "Check Pump Stop Time", "Save LS App Config", "Init Data File", "Reset LS Cycles", "Reset Anomalies", "Reset Opens", "Save LS Data", "Save LS Test Data", "Check Serial Numbers", "Main Tab", "Allow Data Note"]
            }
            frame 17 {
              w223 = T15[] [enum."Save App Config", enum."Write Pumps Present"] items=["Main", "Init Files", "Init", "Unused", "Save As", "Start Profile", "Check Step Time", "Alarm", "Alarm Dismiss", "Run Step", "Stop Profile", "Cycle Reset", "Time Reset", "Time Reset All", "Time Set", "Tare CTs", "Save Profile", "Open Profile", "Get Profiles", "Update Screen", "Update Controls", "Save App Config", "Write Outputs", "Disable Background", "Enable Background", "Get/Release Control", "Log Fuel Change", "Fuel Change Popup", "Read Inputs", "Remote Timer Reset", "Controller Change", "Get Alarms", "Init Alarms", "Save Alarms", "Voltage Selection", "Set Watlow Temp 1", "Set Watlow Temp 2", "Get Pressure", "Write Tare Pressure", "Adjust Controls", "Reinit ADC", "Write Initial Times", "Write Pumps Present", "HMI Command", "Save Pump Times", "Check Pump Stop Time", "Save LS App Config", "Init Data File", "Reset LS Cycles", "Reset Anomalies", "Reset Opens", "Save LS Data", "Save LS Test Data", "Check Serial Numbers", "Main Tab", "Allow Data Note"]
              n50 = Unbundle By Name(w224) -> ("App Config.Pumps Present"=w228:T8)
              n51 = Not Equal?(x="Pumps Present", y=w228) -> (x != y?=w225:bool)
              n52 = Bundle By Name(cluster=w227, "App Config.Pumps Present"="Pumps Present") -> (w226:T26)
            }
            frame 18 {
              w231 = T15[] [enum."Get/Release Control"] items=["Main", "Init Files", "Init", "Unused", "Save As", "Start Profile", "Check Step Time", "Alarm", "Alarm Dismiss", "Run Step", "Stop Profile", "Cycle Reset", "Time Reset", "Time Reset All", "Time Set", "Tare CTs", "Save Profile", "Open Profile", "Get Profiles", "Update Screen", "Update Controls", "Save App Config", "Write Outputs", "Disable Background", "Enable Background", "Get/Release Control", "Log Fuel Change", "Fuel Change Popup", "Read Inputs", "Remote Timer Reset", "Controller Change", "Get Alarms", "Init Alarms", "Save Alarms", "Voltage Selection", "Set Watlow Temp 1", "Set Watlow Temp 2", "Get Pressure", "Write Tare Pressure", "Adjust Controls", "Reinit ADC", "Write Initial Times", "Write Pumps Present", "HMI Command", "Save Pump Times", "Check Pump Stop Time", "Save LS App Config", "Init Data File", "Reset LS Cycles", "Reset Anomalies", "Reset Opens", "Save LS Data", "Save LS Test Data", "Check Serial Numbers", "Main Tab", "Allow Data Note"]
              n53 = Unbundle By Name(w232) -> ("Login"=w236:bool)
              n54 = call "App Global.vi"("Mode"=App_Global_Mode."Write Login", "Login"="Login") -> ()  [unwired: 7 in, 3 out]
              n55 = Not Equal?(x="Login", y=w236) -> (x != y?=w233:bool)
              n56 = Bundle By Name(cluster=w235, "Login"="Login") -> (w234:T26)
            }
            frame 19 {
              w238 = T15[] [enum."Save App Config"] items=["Main", "Init Files", "Init", "Unused", "Save As", "Start Profile", "Check Step Time", "Alarm", "Alarm Dismiss", "Run Step", "Stop Profile", "Cycle Reset", "Time Reset", "Time Reset All", "Time Set", "Tare CTs", "Save Profile", "Open Profile", "Get Profiles", "Update Screen", "Update Controls", "Save App Config", "Write Outputs", "Disable Background", "Enable Background", "Get/Release Control", "Log Fuel Change", "Fuel Change Popup", "Read Inputs", "Remote Timer Reset", "Controller Change", "Get Alarms", "Init Alarms", "Save Alarms", "Voltage Selection", "Set Watlow Temp 1", "Set Watlow Temp 2", "Get Pressure", "Write Tare Pressure", "Adjust Controls", "Reinit ADC", "Write Initial Times", "Write Pumps Present", "HMI Command", "Save Pump Times", "Check Pump Stop Time", "Save LS App Config", "Init Data File", "Reset LS Cycles", "Reset Anomalies", "Reset Opens", "Save LS Data", "Save LS Test Data", "Check Serial Numbers", "Main Tab", "Allow Data Note"]
              n57 = Unbundle By Name(w239) -> ("App Config.Stagger Time (ms)"=w243:i32)
              n58 = Not Equal?(x="Stagger Time (ms):", y=w243) -> (x != y?=w240:bool)
              n59 = Bundle By Name(cluster=w242, "App Config.Stagger Time (ms)"="Stagger Time (ms):") -> (w241:T26)
            }
            frame 20 {
              w247 = T15[] [enum."Write Outputs"] items=["Main", "Init Files", "Init", "Unused", "Save As", "Start Profile", "Check Step Time", "Alarm", "Alarm Dismiss", "Run Step", "Stop Profile", "Cycle Reset", "Time Reset", "Time Reset All", "Time Set", "Tare CTs", "Save Profile", "Open Profile", "Get Profiles", "Update Screen", "Update Controls", "Save App Config", "Write Outputs", "Disable Background", "Enable Background", "Get/Release Control", "Log Fuel Change", "Fuel Change Popup", "Read Inputs", "Remote Timer Reset", "Controller Change", "Get Alarms", "Init Alarms", "Save Alarms", "Voltage Selection", "Set Watlow Temp 1", "Set Watlow Temp 2", "Get Pressure", "Write Tare Pressure", "Adjust Controls", "Reinit ADC", "Write Initial Times", "Write Pumps Present", "HMI Command", "Save Pump Times", "Check Pump Stop Time", "Save LS App Config", "Init Data File", "Reset LS Cycles", "Reset Anomalies", "Reset Opens", "Save LS Data", "Save LS Test Data", "Check Serial Numbers", "Main Tab", "Allow Data Note"]
              n60 = Unbundle By Name(w248) -> ("Tank CMDs.Press CMD"=w246:dbl)
              n61 = Not Equal?(x="PressureCMD", y=w246) -> (x != y?=w244:bool)
              n62 = Bundle By Name(cluster=w250, "Tank CMDs.Press CMD"="PressureCMD") -> (w249:T26)
            }
            frame 21 {
              w253 = T15[] [enum."Disable Background", enum."Log Fuel Change", enum."Fuel Change Popup"] items=["Main", "Init Files", "Init", "Unused", "Save As", "Start Profile", "Check Step Time", "Alarm", "Alarm Dismiss", "Run Step", "Stop Profile", "Cycle Reset", "Time Reset", "Time Reset All", "Time Set", "Tare CTs", "Save Profile", "Open Profile", "Get Profiles", "Update Screen", "Update Controls", "Save App Config", "Write Outputs", "Disable Background", "Enable Background", "Get/Release Control", "Log Fuel Change", "Fuel Change Popup", "Read Inputs", "Remote Timer Reset", "Controller Change", "Get Alarms", "Init Alarms", "Save Alarms", "Voltage Selection", "Set Watlow Temp 1", "Set Watlow Temp 2", "Get Pressure", "Write Tare Pressure", "Adjust Controls", "Reinit ADC", "Write Initial Times", "Write Pumps Present", "HMI Command", "Save Pump Times", "Check Pump Stop Time", "Save LS App Config", "Init Data File", "Reset LS Cycles", "Reset Anomalies", "Reset Opens", "Save LS Data", "Save LS Test Data", "Check Serial Numbers", "Main Tab", "Allow Data Note"]
            }
            frame 22 {
              w260 = T15[] [enum."Save App Config"] items=["Main", "Init Files", "Init", "Unused", "Save As", "Start Profile", "Check Step Time", "Alarm", "Alarm Dismiss", "Run Step", "Stop Profile", "Cycle Reset", "Time Reset", "Time Reset All", "Time Set", "Tare CTs", "Save Profile", "Open Profile", "Get Profiles", "Update Screen", "Update Controls", "Save App Config", "Write Outputs", "Disable Background", "Enable Background", "Get/Release Control", "Log Fuel Change", "Fuel Change Popup", "Read Inputs", "Remote Timer Reset", "Controller Change", "Get Alarms", "Init Alarms", "Save Alarms", "Voltage Selection", "Set Watlow Temp 1", "Set Watlow Temp 2", "Get Pressure", "Write Tare Pressure", "Adjust Controls", "Reinit ADC", "Write Initial Times", "Write Pumps Present", "HMI Command", "Save Pump Times", "Check Pump Stop Time", "Save LS App Config", "Init Data File", "Reset LS Cycles", "Reset Anomalies", "Reset Opens", "Save LS Data", "Save LS Test Data", "Check Serial Numbers", "Main Tab", "Allow Data Note"]
              n63 = Unbundle By Name(w257) -> ("App Config.Tank 1 Fuel"=w256:string)
              n64 = Not Equal?(x=w256, y="Tank 1 Fuel Type:") -> (x != y?=w254:bool)
              n65 = Bundle By Name(cluster=w259, "App Config.Tank 1 Fuel"="Tank 1 Fuel Type:") -> (w258:T26)
            }
            frame 23 {
              w267 = T15[] [enum."Save App Config"] items=["Main", "Init Files", "Init", "Unused", "Save As", "Start Profile", "Check Step Time", "Alarm", "Alarm Dismiss", "Run Step", "Stop Profile", "Cycle Reset", "Time Reset", "Time Reset All", "Time Set", "Tare CTs", "Save Profile", "Open Profile", "Get Profiles", "Update Screen", "Update Controls", "Save App Config", "Write Outputs", "Disable Background", "Enable Background", "Get/Release Control", "Log Fuel Change", "Fuel Change Popup", "Read Inputs", "Remote Timer Reset", "Controller Change", "Get Alarms", "Init Alarms", "Save Alarms", "Voltage Selection", "Set Watlow Temp 1", "Set Watlow Temp 2", "Get Pressure", "Write Tare Pressure", "Adjust Controls", "Reinit ADC", "Write Initial Times", "Write Pumps Present", "HMI Command", "Save Pump Times", "Check Pump Stop Time", "Save LS App Config", "Init Data File", "Reset LS Cycles", "Reset Anomalies", "Reset Opens", "Save LS Data", "Save LS Test Data", "Check Serial Numbers", "Main Tab", "Allow Data Note"]
              n66 = Unbundle By Name(w264) -> ("App Config.Tank 2 Fuel"=w262:string)
              n67 = Not Equal?(x=w262, y="Tank 2 Fuel Type:") -> (x != y?=w263:bool)
              n68 = Bundle By Name(cluster=w266, "App Config.Tank 2 Fuel"="Tank 2 Fuel Type:") -> (w265:T26)
            }
            frame 24 {
              w274 = T15[] [enum."Save App Config"] items=["Main", "Init Files", "Init", "Unused", "Save As", "Start Profile", "Check Step Time", "Alarm", "Alarm Dismiss", "Run Step", "Stop Profile", "Cycle Reset", "Time Reset", "Time Reset All", "Time Set", "Tare CTs", "Save Profile", "Open Profile", "Get Profiles", "Update Screen", "Update Controls", "Save App Config", "Write Outputs", "Disable Background", "Enable Background", "Get/Release Control", "Log Fuel Change", "Fuel Change Popup", "Read Inputs", "Remote Timer Reset", "Controller Change", "Get Alarms", "Init Alarms", "Save Alarms", "Voltage Selection", "Set Watlow Temp 1", "Set Watlow Temp 2", "Get Pressure", "Write Tare Pressure", "Adjust Controls", "Reinit ADC", "Write Initial Times", "Write Pumps Present", "HMI Command", "Save Pump Times", "Check Pump Stop Time", "Save LS App Config", "Init Data File", "Reset LS Cycles", "Reset Anomalies", "Reset Opens", "Save LS Data", "Save LS Test Data", "Check Serial Numbers", "Main Tab", "Allow Data Note"]
              n69 = Unbundle By Name(w271) -> ("App Config.Serial Numbers"=w270:T41)
              n70 = Not Equal?(x=w270, y="Serial Numbers") -> (x != y?=w268:bool)
              n71 = Bundle By Name(cluster=w273, "App Config.Serial Numbers"="Serial Numbers") -> (w272:T26)
            }
            frame 25 {
              w278 = T15[] [enum."Write Pumps Present", enum."Save App Config"] items=["Main", "Init Files", "Init", "Unused", "Save As", "Start Profile", "Check Step Time", "Alarm", "Alarm Dismiss", "Run Step", "Stop Profile", "Cycle Reset", "Time Reset", "Time Reset All", "Time Set", "Tare CTs", "Save Profile", "Open Profile", "Get Profiles", "Update Screen", "Update Controls", "Save App Config", "Write Outputs", "Disable Background", "Enable Background", "Get/Release Control", "Log Fuel Change", "Fuel Change Popup", "Read Inputs", "Remote Timer Reset", "Controller Change", "Get Alarms", "Init Alarms", "Save Alarms", "Voltage Selection", "Set Watlow Temp 1", "Set Watlow Temp 2", "Get Pressure", "Write Tare Pressure", "Adjust Controls", "Reinit ADC", "Write Initial Times", "Write Pumps Present", "HMI Command", "Save Pump Times", "Check Pump Stop Time", "Save LS App Config", "Init Data File", "Reset LS Cycles", "Reset Anomalies", "Reset Opens", "Save LS Data", "Save LS Test Data", "Check Serial Numbers", "Main Tab", "Allow Data Note"]
              n72 = Unbundle By Name(w279) -> ("Power Relay"=w277:T8)
              n73 = Not Equal?(x="Power Relay", y=w277) -> (x != y?=w275:bool)
              n74 = Bundle By Name(cluster=w281, "Power Relay"="Power Relay") -> (w280:T26)
            }
            frame 26 {
              w288 = T15[] [enum."Write Pumps Present", enum."Save App Config"] items=["Main", "Init Files", "Init", "Unused", "Save As", "Start Profile", "Check Step Time", "Alarm", "Alarm Dismiss", "Run Step", "Stop Profile", "Cycle Reset", "Time Reset", "Time Reset All", "Time Set", "Tare CTs", "Save Profile", "Open Profile", "Get Profiles", "Update Screen", "Update Controls", "Save App Config", "Write Outputs", "Disable Background", "Enable Background", "Get/Release Control", "Log Fuel Change", "Fuel Change Popup", "Read Inputs", "Remote Timer Reset", "Controller Change", "Get Alarms", "Init Alarms", "Save Alarms", "Voltage Selection", "Set Watlow Temp 1", "Set Watlow Temp 2", "Get Pressure", "Write Tare Pressure", "Adjust Controls", "Reinit ADC", "Write Initial Times", "Write Pumps Present", "HMI Command", "Save Pump Times", "Check Pump Stop Time", "Save LS App Config", "Init Data File", "Reset LS Cycles", "Reset Anomalies", "Reset Opens", "Save LS Data", "Save LS Test Data", "Check Serial Numbers", "Main Tab", "Allow Data Note"]
              n75 = Unbundle By Name(w286) -> ("Ignition Relay"=w283:T8)
              n76 = Not Equal?(x="Ignition Relay", y=w283) -> (x != y?=w287:bool)
              n77 = Bundle By Name(cluster=w285, "Ignition Relay"="Ignition Relay") -> (w284:T26)
            }
            frame 27 {
              n78 = Unbundle By Name(w293) -> ("HMI.HMI Mom Buttons"=w292:T22)
              n79 = Cluster To Array(cluster=w292) -> (array=w297:bool[])
              n80 = Search 1D Array(1D array=w297, element=TRUE) -> (index of element=w295:i32)  [unwired: 1 in]
              n81 = case shown="1" w295 {
                tunnel: [w299 w300 w301 w302 w303] -> w298
                frame -1, Default {
                  w299 = T15[] [] items=["Main", "Init Files", "Init", "Unused", "Save As", "Start Profile", "Check Step Time", "Alarm", "Alarm Dismiss", "Run Step", "Stop Profile", "Cycle Reset", "Time Reset", "Time Reset All", "Time Set", "Tare CTs", "Save Profile", "Open Profile", "Get Profiles", "Update Screen", "Update Controls", "Save App Config", "Write Outputs", "Disable Background", "Enable Background", "Get/Release Control", "Log Fuel Change", "Fuel Change Popup", "Read Inputs", "Remote Timer Reset", "Controller Change", "Get Alarms", "Init Alarms", "Save Alarms", "Voltage Selection", "Set Watlow Temp 1", "Set Watlow Temp 2", "Get Pressure", "Write Tare Pressure", "Adjust Controls", "Reinit ADC", "Write Initial Times", "Write Pumps Present", "HMI Command", "Save Pump Times", "Check Pump Stop Time", "Save LS App Config", "Init Data File", "Reset LS Cycles", "Reset Anomalies", "Reset Opens", "Save LS Data", "Save LS Test Data", "Check Serial Numbers", "Main Tab", "Allow Data Note"]
                }
                frame 0 {
                  w300 = T15[] [enum."Stop Profile"] items=["Main", "Init Files", "Init", "Unused", "Save As", "Start Profile", "Check Step Time", "Alarm", "Alarm Dismiss", "Run Step", "Stop Profile", "Cycle Reset", "Time Reset", "Time Reset All", "Time Set", "Tare CTs", "Save Profile", "Open Profile", "Get Profiles", "Update Screen", "Update Controls", "Save App Config", "Write Outputs", "Disable Background", "Enable Background", "Get/Release Control", "Log Fuel Change", "Fuel Change Popup", "Read Inputs", "Remote Timer Reset", "Controller Change", "Get Alarms", "Init Alarms", "Save Alarms", "Voltage Selection", "Set Watlow Temp 1", "Set Watlow Temp 2", "Get Pressure", "Write Tare Pressure", "Adjust Controls", "Reinit ADC", "Write Initial Times", "Write Pumps Present", "HMI Command", "Save Pump Times", "Check Pump Stop Time", "Save LS App Config", "Init Data File", "Reset LS Cycles", "Reset Anomalies", "Reset Opens", "Save LS Data", "Save LS Test Data", "Check Serial Numbers", "Main Tab", "Allow Data Note"]
                }
                frame 1 {
                  w301 = T15[] [enum."Remote Timer Reset"] items=["Main", "Init Files", "Init", "Unused", "Save As", "Start Profile", "Check Step Time", "Alarm", "Alarm Dismiss", "Run Step", "Stop Profile", "Cycle Reset", "Time Reset", "Time Reset All", "Time Set", "Tare CTs", "Save Profile", "Open Profile", "Get Profiles", "Update Screen", "Update Controls", "Save App Config", "Write Outputs", "Disable Background", "Enable Background", "Get/Release Control", "Log Fuel Change", "Fuel Change Popup", "Read Inputs", "Remote Timer Reset", "Controller Change", "Get Alarms", "Init Alarms", "Save Alarms", "Voltage Selection", "Set Watlow Temp 1", "Set Watlow Temp 2", "Get Pressure", "Write Tare Pressure", "Adjust Controls", "Reinit ADC", "Write Initial Times", "Write Pumps Present", "HMI Command", "Save Pump Times", "Check Pump Stop Time", "Save LS App Config", "Init Data File", "Reset LS Cycles", "Reset Anomalies", "Reset Opens", "Save LS Data", "Save LS Test Data", "Check Serial Numbers", "Main Tab", "Allow Data Note"]
                }
                frame 2 {
                  w302 = T15[] [enum."Log Fuel Change"] items=["Main", "Init Files", "Init", "Unused", "Save As", "Start Profile", "Check Step Time", "Alarm", "Alarm Dismiss", "Run Step", "Stop Profile", "Cycle Reset", "Time Reset", "Time Reset All", "Time Set", "Tare CTs", "Save Profile", "Open Profile", "Get Profiles", "Update Screen", "Update Controls", "Save App Config", "Write Outputs", "Disable Background", "Enable Background", "Get/Release Control", "Log Fuel Change", "Fuel Change Popup", "Read Inputs", "Remote Timer Reset", "Controller Change", "Get Alarms", "Init Alarms", "Save Alarms", "Voltage Selection", "Set Watlow Temp 1", "Set Watlow Temp 2", "Get Pressure", "Write Tare Pressure", "Adjust Controls", "Reinit ADC", "Write Initial Times", "Write Pumps Present", "HMI Command", "Save Pump Times", "Check Pump Stop Time", "Save LS App Config", "Init Data File", "Reset LS Cycles", "Reset Anomalies", "Reset Opens", "Save LS Data", "Save LS Test Data", "Check Serial Numbers", "Main Tab", "Allow Data Note"]
                }
                frame 3 {
                  w303 = T15[] [enum."Alarm Dismiss"] items=["Main", "Init Files", "Init", "Unused", "Save As", "Start Profile", "Check Step Time", "Alarm", "Alarm Dismiss", "Run Step", "Stop Profile", "Cycle Reset", "Time Reset", "Time Reset All", "Time Set", "Tare CTs", "Save Profile", "Open Profile", "Get Profiles", "Update Screen", "Update Controls", "Save App Config", "Write Outputs", "Disable Background", "Enable Background", "Get/Release Control", "Log Fuel Change", "Fuel Change Popup", "Read Inputs", "Remote Timer Reset", "Controller Change", "Get Alarms", "Init Alarms", "Save Alarms", "Voltage Selection", "Set Watlow Temp 1", "Set Watlow Temp 2", "Get Pressure", "Write Tare Pressure", "Adjust Controls", "Reinit ADC", "Write Initial Times", "Write Pumps Present", "HMI Command", "Save Pump Times", "Check Pump Stop Time", "Save LS App Config", "Init Data File", "Reset LS Cycles", "Reset Anomalies", "Reset Opens", "Save LS Data", "Save LS Test Data", "Check Serial Numbers", "Main Tab", "Allow Data Note"]
                }
              }
              n82 = Greater Or Equal To 0?(x=w295) -> (x >= 0?=w294:bool)
              n83 = Bundle By Name(cluster=w291, "HMI.HMI Mom Buttons"=T22 {"Stop"=FALSE, "Reset Timers"=FALSE, "Log Fuel Change"=FALSE, "Alarm Dismiss"=FALSE}) -> (w290:T26)
            }
            frame 28 {
              w310 = T15[] [enum."Save Alarms"] items=["Main", "Init Files", "Init", "Unused", "Save As", "Start Profile", "Check Step Time", "Alarm", "Alarm Dismiss", "Run Step", "Stop Profile", "Cycle Reset", "Time Reset", "Time Reset All", "Time Set", "Tare CTs", "Save Profile", "Open Profile", "Get Profiles", "Update Screen", "Update Controls", "Save App Config", "Write Outputs", "Disable Background", "Enable Background", "Get/Release Control", "Log Fuel Change", "Fuel Change Popup", "Read Inputs", "Remote Timer Reset", "Controller Change", "Get Alarms", "Init Alarms", "Save Alarms", "Voltage Selection", "Set Watlow Temp 1", "Set Watlow Temp 2", "Get Pressure", "Write Tare Pressure", "Adjust Controls", "Reinit ADC", "Write Initial Times", "Write Pumps Present", "HMI Command", "Save Pump Times", "Check Pump Stop Time", "Save LS App Config", "Init Data File", "Reset LS Cycles", "Reset Anomalies", "Reset Opens", "Save LS Data", "Save LS Test Data", "Check Serial Numbers", "Main Tab", "Allow Data Note"]
              n84 = Unbundle By Name(w308) -> ("Alarm Config"=w305:T10)
              n85 = Not Equal?(x="Alarm Config", y=w305) -> (x != y?=w309:bool)
              n86 = Bundle By Name(cluster=w307, "Alarm Config"="Alarm Config") -> (w306:T26)
            }
            frame 29 {
              w317 = T15[] [enum."Set Watlow Temp 1", enum."Save App Config"] items=["Main", "Init Files", "Init", "Unused", "Save As", "Start Profile", "Check Step Time", "Alarm", "Alarm Dismiss", "Run Step", "Stop Profile", "Cycle Reset", "Time Reset", "Time Reset All", "Time Set", "Tare CTs", "Save Profile", "Open Profile", "Get Profiles", "Update Screen", "Update Controls", "Save App Config", "Write Outputs", "Disable Background", "Enable Background", "Get/Release Control", "Log Fuel Change", "Fuel Change Popup", "Read Inputs", "Remote Timer Reset", "Controller Change", "Get Alarms", "Init Alarms", "Save Alarms", "Voltage Selection", "Set Watlow Temp 1", "Set Watlow Temp 2", "Get Pressure", "Write Tare Pressure", "Adjust Controls", "Reinit ADC", "Write Initial Times", "Write Pumps Present", "HMI Command", "Save Pump Times", "Check Pump Stop Time", "Save LS App Config", "Init Data File", "Reset LS Cycles", "Reset Anomalies", "Reset Opens", "Save LS Data", "Save LS Test Data", "Check Serial Numbers", "Main Tab", "Allow Data Note"]
              n87 = Unbundle By Name(w316) -> ("Tank CMDs.Temp 1 CMD"=w313:dbl)
              n88 = Not Equal?(x="Tank 1 Temp Cmd:", y=w313) -> (x != y?=w311:bool)
              n89 = Bundle By Name(cluster=w315, "Tank CMDs.Temp 1 CMD"="Tank 1 Temp Cmd:", "App Config.Temp 1"="Tank 1 Temp Cmd:") -> (w314:T26)
            }
            frame 30 {
              w324 = T15[] [enum."Set Watlow Temp 2", enum."Save App Config"] items=["Main", "Init Files", "Init", "Unused", "Save As", "Start Profile", "Check Step Time", "Alarm", "Alarm Dismiss", "Run Step", "Stop Profile", "Cycle Reset", "Time Reset", "Time Reset All", "Time Set", "Tare CTs", "Save Profile", "Open Profile", "Get Profiles", "Update Screen", "Update Controls", "Save App Config", "Write Outputs", "Disable Background", "Enable Background", "Get/Release Control", "Log Fuel Change", "Fuel Change Popup", "Read Inputs", "Remote Timer Reset", "Controller Change", "Get Alarms", "Init Alarms", "Save Alarms", "Voltage Selection", "Set Watlow Temp 1", "Set Watlow Temp 2", "Get Pressure", "Write Tare Pressure", "Adjust Controls", "Reinit ADC", "Write Initial Times", "Write Pumps Present", "HMI Command", "Save Pump Times", "Check Pump Stop Time", "Save LS App Config", "Init Data File", "Reset LS Cycles", "Reset Anomalies", "Reset Opens", "Save LS Data", "Save LS Test Data", "Check Serial Numbers", "Main Tab", "Allow Data Note"]
              n90 = Unbundle By Name(w323) -> ("Tank CMDs.Temp 2 CMD"=w320:dbl)
              n91 = Not Equal?(x="Tank 2 Temp Cmd:", y=w320) -> (x != y?=w318:bool)
              n92 = Bundle By Name(cluster=w322, "Tank CMDs.Temp 2 CMD"="Tank 2 Temp Cmd:", "App Config.Temp 2"="Tank 2 Temp Cmd:") -> (w321:T26)
            }
            frame 31 {
              w327 = T15[] [enum."Alarm Dismiss"] items=["Main", "Init Files", "Init", "Unused", "Save As", "Start Profile", "Check Step Time", "Alarm", "Alarm Dismiss", "Run Step", "Stop Profile", "Cycle Reset", "Time Reset", "Time Reset All", "Time Set", "Tare CTs", "Save Profile", "Open Profile", "Get Profiles", "Update Screen", "Update Controls", "Save App Config", "Write Outputs", "Disable Background", "Enable Background", "Get/Release Control", "Log Fuel Change", "Fuel Change Popup", "Read Inputs", "Remote Timer Reset", "Controller Change", "Get Alarms", "Init Alarms", "Save Alarms", "Voltage Selection", "Set Watlow Temp 1", "Set Watlow Temp 2", "Get Pressure", "Write Tare Pressure", "Adjust Controls", "Reinit ADC", "Write Initial Times", "Write Pumps Present", "HMI Command", "Save Pump Times", "Check Pump Stop Time", "Save LS App Config", "Init Data File", "Reset LS Cycles", "Reset Anomalies", "Reset Opens", "Save LS Data", "Save LS Test Data", "Check Serial Numbers", "Main Tab", "Allow Data Note"]
            }
            frame 32 {
              w330 = T15[] [enum."Get Pressure"] items=["Main", "Init Files", "Init", "Unused", "Save As", "Start Profile", "Check Step Time", "Alarm", "Alarm Dismiss", "Run Step", "Stop Profile", "Cycle Reset", "Time Reset", "Time Reset All", "Time Set", "Tare CTs", "Save Profile", "Open Profile", "Get Profiles", "Update Screen", "Update Controls", "Save App Config", "Write Outputs", "Disable Background", "Enable Background", "Get/Release Control", "Log Fuel Change", "Fuel Change Popup", "Read Inputs", "Remote Timer Reset", "Controller Change", "Get Alarms", "Init Alarms", "Save Alarms", "Voltage Selection", "Set Watlow Temp 1", "Set Watlow Temp 2", "Get Pressure", "Write Tare Pressure", "Adjust Controls", "Reinit ADC", "Write Initial Times", "Write Pumps Present", "HMI Command", "Save Pump Times", "Check Pump Stop Time", "Save LS App Config", "Init Data File", "Reset LS Cycles", "Reset Anomalies", "Reset Opens", "Save LS Data", "Save LS Test Data", "Check Serial Numbers", "Main Tab", "Allow Data Note"]
            }
            frame 33 {
              w332 = T15[] [enum."Save App Config"] items=["Main", "Init Files", "Init", "Unused", "Save As", "Start Profile", "Check Step Time", "Alarm", "Alarm Dismiss", "Run Step", "Stop Profile", "Cycle Reset", "Time Reset", "Time Reset All", "Time Set", "Tare CTs", "Save Profile", "Open Profile", "Get Profiles", "Update Screen", "Update Controls", "Save App Config", "Write Outputs", "Disable Background", "Enable Background", "Get/Release Control", "Log Fuel Change", "Fuel Change Popup", "Read Inputs", "Remote Timer Reset", "Controller Change", "Get Alarms", "Init Alarms", "Save Alarms", "Voltage Selection", "Set Watlow Temp 1", "Set Watlow Temp 2", "Get Pressure", "Write Tare Pressure", "Adjust Controls", "Reinit ADC", "Write Initial Times", "Write Pumps Present", "HMI Command", "Save Pump Times", "Check Pump Stop Time", "Save LS App Config", "Init Data File", "Reset LS Cycles", "Reset Anomalies", "Reset Opens", "Save LS Data", "Save LS Test Data", "Check Serial Numbers", "Main Tab", "Allow Data Note"]
              n93 = Unbundle By Name(w337) -> ("App Config.V_Run PI?"=w334:bool)
              n94 = Not Equal?(x="Closed Loop Voltage", y=w334) -> (x != y?=w333:bool)
              n95 = Bundle By Name(cluster=w336, "App Config.V_Run PI?"="Closed Loop Voltage") -> (w335:T26)
            }
            frame 34 {
              w342 = T15[] [enum."Adjust Controls", enum."Save App Config"] items=["Main", "Init Files", "Init", "Unused", "Save As", "Start Profile", "Check Step Time", "Alarm", "Alarm Dismiss", "Run Step", "Stop Profile", "Cycle Reset", "Time Reset", "Time Reset All", "Time Set", "Tare CTs", "Save Profile", "Open Profile", "Get Profiles", "Update Screen", "Update Controls", "Save App Config", "Write Outputs", "Disable Background", "Enable Background", "Get/Release Control", "Log Fuel Change", "Fuel Change Popup", "Read Inputs", "Remote Timer Reset", "Controller Change", "Get Alarms", "Init Alarms", "Save Alarms", "Voltage Selection", "Set Watlow Temp 1", "Set Watlow Temp 2", "Get Pressure", "Write Tare Pressure", "Adjust Controls", "Reinit ADC", "Write Initial Times", "Write Pumps Present", "HMI Command", "Save Pump Times", "Check Pump Stop Time", "Save LS App Config", "Init Data File", "Reset LS Cycles", "Reset Anomalies", "Reset Opens", "Save LS Data", "Save LS Test Data", "Check Serial Numbers", "Main Tab", "Allow Data Note"]
              n96 = Unbundle By Name(w346) -> ("App Config.Voltage Limits"=w343:T42)
              n97 = Not Equal?(x="Voltage Limits", y=w343) -> (x != y?=w339:cluster{bool, bool, bool})
              n98 = Cluster To Array(cluster=w339) -> (array=w340:bool[])
              n99 = Or Array Elements(Boolean array=w340) -> (logical OR=w338:bool)
              n100 = Bundle By Name(cluster=w345, "App Config.Voltage Limits"="Voltage Limits") -> (w344:T26)
            }
            frame 35 {
              w347 = T15[] [enum."Adjust Controls", enum."Save App Config"] items=["Main", "Init Files", "Init", "Unused", "Save As", "Start Profile", "Check Step Time", "Alarm", "Alarm Dismiss", "Run Step", "Stop Profile", "Cycle Reset", "Time Reset", "Time Reset All", "Time Set", "Tare CTs", "Save Profile", "Open Profile", "Get Profiles", "Update Screen", "Update Controls", "Save App Config", "Write Outputs", "Disable Background", "Enable Background", "Get/Release Control", "Log Fuel Change", "Fuel Change Popup", "Read Inputs", "Remote Timer Reset", "Controller Change", "Get Alarms", "Init Alarms", "Save Alarms", "Voltage Selection", "Set Watlow Temp 1", "Set Watlow Temp 2", "Get Pressure", "Write Tare Pressure", "Adjust Controls", "Reinit ADC", "Write Initial Times", "Write Pumps Present", "HMI Command", "Save Pump Times", "Check Pump Stop Time", "Save LS App Config", "Init Data File", "Reset LS Cycles", "Reset Anomalies", "Reset Opens", "Save LS Data", "Save LS Test Data", "Check Serial Numbers", "Main Tab", "Allow Data Note"]
              n101 = Unbundle By Name(w355) -> ("App Config.Voltage Far PI"=w352:T43)
              n102 = Not Equal?(x="Far PI", y=w352) -> (x != y?=w349:cluster{bool, bool, bool})
              n103 = Cluster To Array(cluster=w349) -> (array=w350:bool[])
              n104 = Or Array Elements(Boolean array=w350) -> (logical OR=w348:bool)
              n105 = Bundle By Name(cluster=w354, "App Config.Voltage Far PI"="Far PI") -> (w353:T26)
            }
            frame 36 {
              w356 = T15[] [enum."Adjust Controls", enum."Save App Config"] items=["Main", "Init Files", "Init", "Unused", "Save As", "Start Profile", "Check Step Time", "Alarm", "Alarm Dismiss", "Run Step", "Stop Profile", "Cycle Reset", "Time Reset", "Time Reset All", "Time Set", "Tare CTs", "Save Profile", "Open Profile", "Get Profiles", "Update Screen", "Update Controls", "Save App Config", "Write Outputs", "Disable Background", "Enable Background", "Get/Release Control", "Log Fuel Change", "Fuel Change Popup", "Read Inputs", "Remote Timer Reset", "Controller Change", "Get Alarms", "Init Alarms", "Save Alarms", "Voltage Selection", "Set Watlow Temp 1", "Set Watlow Temp 2", "Get Pressure", "Write Tare Pressure", "Adjust Controls", "Reinit ADC", "Write Initial Times", "Write Pumps Present", "HMI Command", "Save Pump Times", "Check Pump Stop Time", "Save LS App Config", "Init Data File", "Reset LS Cycles", "Reset Anomalies", "Reset Opens", "Save LS Data", "Save LS Test Data", "Check Serial Numbers", "Main Tab", "Allow Data Note"]
              n106 = Unbundle By Name(w364) -> ("App Config.Voltage Mid PI"=w361:T44)
              n107 = Not Equal?(x="Mid PI", y=w361) -> (x != y?=w359:cluster{bool, bool, bool})
              n108 = Cluster To Array(cluster=w359) -> (array=w360:bool[])
              n109 = Or Array Elements(Boolean array=w360) -> (logical OR=w358:bool)
              n110 = Bundle By Name(cluster=w363, "App Config.Voltage Mid PI"="Mid PI") -> (w362:T26)
            }
            frame 37 {
              w365 = T15[] [enum."Adjust Controls", enum."Save App Config"] items=["Main", "Init Files", "Init", "Unused", "Save As", "Start Profile", "Check Step Time", "Alarm", "Alarm Dismiss", "Run Step", "Stop Profile", "Cycle Reset", "Time Reset", "Time Reset All", "Time Set", "Tare CTs", "Save Profile", "Open Profile", "Get Profiles", "Update Screen", "Update Controls", "Save App Config", "Write Outputs", "Disable Background", "Enable Background", "Get/Release Control", "Log Fuel Change", "Fuel Change Popup", "Read Inputs", "Remote Timer Reset", "Controller Change", "Get Alarms", "Init Alarms", "Save Alarms", "Voltage Selection", "Set Watlow Temp 1", "Set Watlow Temp 2", "Get Pressure", "Write Tare Pressure", "Adjust Controls", "Reinit ADC", "Write Initial Times", "Write Pumps Present", "HMI Command", "Save Pump Times", "Check Pump Stop Time", "Save LS App Config", "Init Data File", "Reset LS Cycles", "Reset Anomalies", "Reset Opens", "Save LS Data", "Save LS Test Data", "Check Serial Numbers", "Main Tab", "Allow Data Note"]
              n111 = Unbundle By Name(w373) -> ("App Config.Voltage Close PI"=w370:T45)
              n112 = Not Equal?(x="Close PI", y=w370) -> (x != y?=w368:cluster{bool, bool, bool})
              n113 = Cluster To Array(cluster=w368) -> (array=w369:bool[])
              n114 = Or Array Elements(Boolean array=w369) -> (logical OR=w367:bool)
              n115 = Bundle By Name(cluster=w372, "App Config.Voltage Close PI"="Close PI") -> (w371:T26)
            }
            frame 38 {
              w374 = T15[] [enum."Adjust Controls", enum."Save App Config"] items=["Main", "Init Files", "Init", "Unused", "Save As", "Start Profile", "Check Step Time", "Alarm", "Alarm Dismiss", "Run Step", "Stop Profile", "Cycle Reset", "Time Reset", "Time Reset All", "Time Set", "Tare CTs", "Save Profile", "Open Profile", "Get Profiles", "Update Screen", "Update Controls", "Save App Config", "Write Outputs", "Disable Background", "Enable Background", "Get/Release Control", "Log Fuel Change", "Fuel Change Popup", "Read Inputs", "Remote Timer Reset", "Controller Change", "Get Alarms", "Init Alarms", "Save Alarms", "Voltage Selection", "Set Watlow Temp 1", "Set Watlow Temp 2", "Get Pressure", "Write Tare Pressure", "Adjust Controls", "Reinit ADC", "Write Initial Times", "Write Pumps Present", "HMI Command", "Save Pump Times", "Check Pump Stop Time", "Save LS App Config", "Init Data File", "Reset LS Cycles", "Reset Anomalies", "Reset Opens", "Save LS Data", "Save LS Test Data", "Check Serial Numbers", "Main Tab", "Allow Data Note"]
              n116 = Unbundle By Name(w382) -> ("App Config.Voltage Scale"=w379:cluster{"V_FFm":dbl, "V_FFb":dbl})
              n117 = Not Equal?(x="Voltage Scale", y=w379) -> (x != y?=w377:cluster{bool, bool})
              n118 = Cluster To Array(cluster=w377) -> (array=w376:bool[])
              n119 = Or Array Elements(Boolean array=w376) -> (logical OR=w375:bool)
              n120 = Bundle By Name(cluster=w381, "App Config.Voltage Scale"="Voltage Scale") -> (w380:T26)
            }
            frame 39 {
              w383 = T15[] [enum."Adjust Controls", enum."Save App Config"] items=["Main", "Init Files", "Init", "Unused", "Save As", "Start Profile", "Check Step Time", "Alarm", "Alarm Dismiss", "Run Step", "Stop Profile", "Cycle Reset", "Time Reset", "Time Reset All", "Time Set", "Tare CTs", "Save Profile", "Open Profile", "Get Profiles", "Update Screen", "Update Controls", "Save App Config", "Write Outputs", "Disable Background", "Enable Background", "Get/Release Control", "Log Fuel Change", "Fuel Change Popup", "Read Inputs", "Remote Timer Reset", "Controller Change", "Get Alarms", "Init Alarms", "Save Alarms", "Voltage Selection", "Set Watlow Temp 1", "Set Watlow Temp 2", "Get Pressure", "Write Tare Pressure", "Adjust Controls", "Reinit ADC", "Write Initial Times", "Write Pumps Present", "HMI Command", "Save Pump Times", "Check Pump Stop Time", "Save LS App Config", "Init Data File", "Reset LS Cycles", "Reset Anomalies", "Reset Opens", "Save LS Data", "Save LS Test Data", "Check Serial Numbers", "Main Tab", "Allow Data Note"]
              n121 = Unbundle By Name(w391) -> ("App Config.Voltage Cutoffs"=w388:cluster{"V_MidCutoff":dbl, "V_CloseCutoff":dbl})
              n122 = Not Equal?(x="Cutoffs", y=w388) -> (x != y?=w387:cluster{bool, bool})
              n123 = Cluster To Array(cluster=w387) -> (array=w386:bool[])
              n124 = Or Array Elements(Boolean array=w386) -> (logical OR=w385:bool)
              n125 = Bundle By Name(cluster=w390, "App Config.Voltage Cutoffs"="Cutoffs") -> (w389:T26)
            }
            frame 40 {
              w396 = T15[] [enum."Save App Config"] items=["Main", "Init Files", "Init", "Unused", "Save As", "Start Profile", "Check Step Time", "Alarm", "Alarm Dismiss", "Run Step", "Stop Profile", "Cycle Reset", "Time Reset", "Time Reset All", "Time Set", "Tare CTs", "Save Profile", "Open Profile", "Get Profiles", "Update Screen", "Update Controls", "Save App Config", "Write Outputs", "Disable Background", "Enable Background", "Get/Release Control", "Log Fuel Change", "Fuel Change Popup", "Read Inputs", "Remote Timer Reset", "Controller Change", "Get Alarms", "Init Alarms", "Save Alarms", "Voltage Selection", "Set Watlow Temp 1", "Set Watlow Temp 2", "Get Pressure", "Write Tare Pressure", "Adjust Controls", "Reinit ADC", "Write Initial Times", "Write Pumps Present", "HMI Command", "Save Pump Times", "Check Pump Stop Time", "Save LS App Config", "Init Data File", "Reset LS Cycles", "Reset Anomalies", "Reset Opens", "Save LS Data", "Save LS Test Data", "Check Serial Numbers", "Main Tab", "Allow Data Note"]
              n126 = Unbundle By Name(w400) -> ("App Config.Pressure Scale"=w397:cluster{"Pres_FFm":dbl, "Pres_FFb":dbl})
              n127 = Not Equal?(x="Pressure Scale", y=w397) -> (x != y?=w395:cluster{bool, bool})
              n128 = Cluster To Array(cluster=w395) -> (array=w394:bool[])
              n129 = Or Array Elements(Boolean array=w394) -> (logical OR=w393:bool)
              n130 = Bundle By Name(cluster=w399, "App Config.Pressure Scale"="Pressure Scale") -> (w398:T26)
            }
            frame 41 {
              w404 = T15[] [enum."Save App Config"] items=["Main", "Init Files", "Init", "Unused", "Save As", "Start Profile", "Check Step Time", "Alarm", "Alarm Dismiss", "Run Step", "Stop Profile", "Cycle Reset", "Time Reset", "Time Reset All", "Time Set", "Tare CTs", "Save Profile", "Open Profile", "Get Profiles", "Update Screen", "Update Controls", "Save App Config", "Write Outputs", "Disable Background", "Enable Background", "Get/Release Control", "Log Fuel Change", "Fuel Change Popup", "Read Inputs", "Remote Timer Reset", "Controller Change", "Get Alarms", "Init Alarms", "Save Alarms", "Voltage Selection", "Set Watlow Temp 1", "Set Watlow Temp 2", "Get Pressure", "Write Tare Pressure", "Adjust Controls", "Reinit ADC", "Write Initial Times", "Write Pumps Present", "HMI Command", "Save Pump Times", "Check Pump Stop Time", "Save LS App Config", "Init Data File", "Reset LS Cycles", "Reset Anomalies", "Reset Opens", "Save LS Data", "Save LS Test Data", "Check Serial Numbers", "Main Tab", "Allow Data Note"]
              n131 = Unbundle By Name(w408) -> ("App Config.Temp Format"=w405:i32)
              n132 = To Long Integer(number="Thermocouple") -> (32bit integer=w401:i32)
              n133 = Not Equal?(x=w401, y=w405) -> (x != y?=w403:bool)
              n134 = Bundle By Name(cluster=w407, "App Config.Temp Format"=w401) -> (w406:T26)
            }
            frame 42 {
              w411 = T15[] [enum."Save App Config"] items=["Main", "Init Files", "Init", "Unused", "Save As", "Start Profile", "Check Step Time", "Alarm", "Alarm Dismiss", "Run Step", "Stop Profile", "Cycle Reset", "Time Reset", "Time Reset All", "Time Set", "Tare CTs", "Save Profile", "Open Profile", "Get Profiles", "Update Screen", "Update Controls", "Save App Config", "Write Outputs", "Disable Background", "Enable Background", "Get/Release Control", "Log Fuel Change", "Fuel Change Popup", "Read Inputs", "Remote Timer Reset", "Controller Change", "Get Alarms", "Init Alarms", "Save Alarms", "Voltage Selection", "Set Watlow Temp 1", "Set Watlow Temp 2", "Get Pressure", "Write Tare Pressure", "Adjust Controls", "Reinit ADC", "Write Initial Times", "Write Pumps Present", "HMI Command", "Save Pump Times", "Check Pump Stop Time", "Save LS App Config", "Init Data File", "Reset LS Cycles", "Reset Anomalies", "Reset Opens", "Save LS Data", "Save LS Test Data", "Check Serial Numbers", "Main Tab", "Allow Data Note"]
              n135 = Unbundle By Name(w415) -> ("App Config.Temp Tolerance"=w412:dbl)
              n136 = Not Equal?(x="Temp Tolerance", y=w412) -> (x != y?=w409:bool)
              n137 = Bundle By Name(cluster=w414, "App Config.Temp Tolerance"="Temp Tolerance") -> (w413:T26)
            }
            frame 43 {
              w422 = T15[] [enum."Save App Config"] items=["Main", "Init Files", "Init", "Unused", "Save As", "Start Profile", "Check Step Time", "Alarm", "Alarm Dismiss", "Run Step", "Stop Profile", "Cycle Reset", "Time Reset", "Time Reset All", "Time Set", "Tare CTs", "Save Profile", "Open Profile", "Get Profiles", "Update Screen", "Update Controls", "Save App Config", "Write Outputs", "Disable Background", "Enable Background", "Get/Release Control", "Log Fuel Change", "Fuel Change Popup", "Read Inputs", "Remote Timer Reset", "Controller Change", "Get Alarms", "Init Alarms", "Save Alarms", "Voltage Selection", "Set Watlow Temp 1", "Set Watlow Temp 2", "Get Pressure", "Write Tare Pressure", "Adjust Controls", "Reinit ADC", "Write Initial Times", "Write Pumps Present", "HMI Command", "Save Pump Times", "Check Pump Stop Time", "Save LS App Config", "Init Data File", "Reset LS Cycles", "Reset Anomalies", "Reset Opens", "Save LS Data", "Save LS Test Data", "Check Serial Numbers", "Main Tab", "Allow Data Note"]
              n138 = Unbundle By Name(w419) -> ("App Config.Target Voltage"=w418:dbl)
              n139 = Not Equal?(x=w418, y="Target Voltage:") -> (x != y?=w417:bool)
              n140 = Bundle By Name(cluster=w421, "App Config.Target Voltage"="Target Voltage:") -> (w420:T26)
            }
            frame 44 {
              w429 = T15[] [enum."Save App Config"] items=["Main", "Init Files", "Init", "Unused", "Save As", "Start Profile", "Check Step Time", "Alarm", "Alarm Dismiss", "Run Step", "Stop Profile", "Cycle Reset", "Time Reset", "Time Reset All", "Time Set", "Tare CTs", "Save Profile", "Open Profile", "Get Profiles", "Update Screen", "Update Controls", "Save App Config", "Write Outputs", "Disable Background", "Enable Background", "Get/Release Control", "Log Fuel Change", "Fuel Change Popup", "Read Inputs", "Remote Timer Reset", "Controller Change", "Get Alarms", "Init Alarms", "Save Alarms", "Voltage Selection", "Set Watlow Temp 1", "Set Watlow Temp 2", "Get Pressure", "Write Tare Pressure", "Adjust Controls", "Reinit ADC", "Write Initial Times", "Write Pumps Present", "HMI Command", "Save Pump Times", "Check Pump Stop Time", "Save LS App Config", "Init Data File", "Reset LS Cycles", "Reset Anomalies", "Reset Opens", "Save LS Data", "Save LS Test Data", "Check Serial Numbers", "Main Tab", "Allow Data Note"]
              n141 = Unbundle By Name(w426) -> ("App Config.Target Pressure"=w425:dbl)
              n142 = Not Equal?(x=w425, y="Target Pressure:") -> (x != y?=w424:bool)
              n143 = Bundle By Name(cluster=w428, "App Config.Target Pressure"="Target Pressure:") -> (w427:T26)
            }
            frame 45 {
              w433 = T15[] [enum."HMI Command"] items=["Main", "Init Files", "Init", "Unused", "Save As", "Start Profile", "Check Step Time", "Alarm", "Alarm Dismiss", "Run Step", "Stop Profile", "Cycle Reset", "Time Reset", "Time Reset All", "Time Set", "Tare CTs", "Save Profile", "Open Profile", "Get Profiles", "Update Screen", "Update Controls", "Save App Config", "Write Outputs", "Disable Background", "Enable Background", "Get/Release Control", "Log Fuel Change", "Fuel Change Popup", "Read Inputs", "Remote Timer Reset", "Controller Change", "Get Alarms", "Init Alarms", "Save Alarms", "Voltage Selection", "Set Watlow Temp 1", "Set Watlow Temp 2", "Get Pressure", "Write Tare Pressure", "Adjust Controls", "Reinit ADC", "Write Initial Times", "Write Pumps Present", "HMI Command", "Save Pump Times", "Check Pump Stop Time", "Save LS App Config", "Init Data File", "Reset LS Cycles", "Reset Anomalies", "Reset Opens", "Save LS Data", "Save LS Test Data", "Check Serial Numbers", "Main Tab", "Allow Data Note"]
              n144 = call "RPi HMI Global.vi"() -> ("HMI Cluster OUT"=w432:T17)  [unwired: 11 in]
              n145 = Unbundle By Name(w432) -> ("HMI Command"=w430:bool)
            }
            frame 46 {
              w440 = T15[] [enum."Update Controls"] items=["Main", "Init Files", "Init", "Unused", "Save As", "Start Profile", "Check Step Time", "Alarm", "Alarm Dismiss", "Run Step", "Stop Profile", "Cycle Reset", "Time Reset", "Time Reset All", "Time Set", "Tare CTs", "Save Profile", "Open Profile", "Get Profiles", "Update Screen", "Update Controls", "Save App Config", "Write Outputs", "Disable Background", "Enable Background", "Get/Release Control", "Log Fuel Change", "Fuel Change Popup", "Read Inputs", "Remote Timer Reset", "Controller Change", "Get Alarms", "Init Alarms", "Save Alarms", "Voltage Selection", "Set Watlow Temp 1", "Set Watlow Temp 2", "Get Pressure", "Write Tare Pressure", "Adjust Controls", "Reinit ADC", "Write Initial Times", "Write Pumps Present", "HMI Command", "Save Pump Times", "Check Pump Stop Time", "Save LS App Config", "Init Data File", "Reset LS Cycles", "Reset Anomalies", "Reset Opens", "Save LS Data", "Save LS Test Data", "Check Serial Numbers", "Main Tab", "Allow Data Note"]
              n146 = Unbundle By Name(w439) -> ("Email Alarms Disabled"=w436:bool)
              n147 = Greater?(x="Disable Alarm Email", y=w436) -> (0:w434:bool)
              n148 = Bundle By Name(cluster=w438, "Email Alarms Disabled"="Disable Alarm Email") -> (w437:T26)
            }
            frame 47 {
              w445 = T15[] [] items=["Main", "Init Files", "Init", "Unused", "Save As", "Start Profile", "Check Step Time", "Alarm", "Alarm Dismiss", "Run Step", "Stop Profile", "Cycle Reset", "Time Reset", "Time Reset All", "Time Set", "Tare CTs", "Save Profile", "Open Profile", "Get Profiles", "Update Screen", "Update Controls", "Save App Config", "Write Outputs", "Disable Background", "Enable Background", "Get/Release Control", "Log Fuel Change", "Fuel Change Popup", "Read Inputs", "Remote Timer Reset", "Controller Change", "Get Alarms", "Init Alarms", "Save Alarms", "Voltage Selection", "Set Watlow Temp 1", "Set Watlow Temp 2", "Get Pressure", "Write Tare Pressure", "Adjust Controls", "Reinit ADC", "Write Initial Times", "Write Pumps Present", "HMI Command", "Save Pump Times", "Check Pump Stop Time", "Save LS App Config", "Init Data File", "Reset LS Cycles", "Reset Anomalies", "Reset Opens", "Save LS Data", "Save LS Test Data", "Check Serial Numbers", "Main Tab", "Allow Data Note"]
              n149 = Bundle By Name(cluster=w444, "Concat Data"="Concat Data") -> (w443:T26)
            }
            frame 48 {
              w450 = T15[] [] items=["Main", "Init Files", "Init", "Unused", "Save As", "Start Profile", "Check Step Time", "Alarm", "Alarm Dismiss", "Run Step", "Stop Profile", "Cycle Reset", "Time Reset", "Time Reset All", "Time Set", "Tare CTs", "Save Profile", "Open Profile", "Get Profiles", "Update Screen", "Update Controls", "Save App Config", "Write Outputs", "Disable Background", "Enable Background", "Get/Release Control", "Log Fuel Change", "Fuel Change Popup", "Read Inputs", "Remote Timer Reset", "Controller Change", "Get Alarms", "Init Alarms", "Save Alarms", "Voltage Selection", "Set Watlow Temp 1", "Set Watlow Temp 2", "Get Pressure", "Write Tare Pressure", "Adjust Controls", "Reinit ADC", "Write Initial Times", "Write Pumps Present", "HMI Command", "Save Pump Times", "Check Pump Stop Time", "Save LS App Config", "Init Data File", "Reset LS Cycles", "Reset Anomalies", "Reset Opens", "Save LS Data", "Save LS Test Data", "Check Serial Numbers", "Main Tab", "Allow Data Note"]
              n150 = Bundle By Name(cluster=w449, "WebDAV Push"="WebDAV Push") -> (w448:T26)
            }
            frame 49 {
              w457 = T15[] [enum."Save App Config"] items=["Main", "Init Files", "Init", "Unused", "Save As", "Start Profile", "Check Step Time", "Alarm", "Alarm Dismiss", "Run Step", "Stop Profile", "Cycle Reset", "Time Reset", "Time Reset All", "Time Set", "Tare CTs", "Save Profile", "Open Profile", "Get Profiles", "Update Screen", "Update Controls", "Save App Config", "Write Outputs", "Disable Background", "Enable Background", "Get/Release Control", "Log Fuel Change", "Fuel Change Popup", "Read Inputs", "Remote Timer Reset", "Controller Change", "Get Alarms", "Init Alarms", "Save Alarms", "Voltage Selection", "Set Watlow Temp 1", "Set Watlow Temp 2", "Get Pressure", "Write Tare Pressure", "Adjust Controls", "Reinit ADC", "Write Initial Times", "Write Pumps Present", "HMI Command", "Save Pump Times", "Check Pump Stop Time", "Save LS App Config", "Init Data File", "Reset LS Cycles", "Reset Anomalies", "Reset Opens", "Save LS Data", "Save LS Test Data", "Check Serial Numbers", "Main Tab", "Allow Data Note"]
              n151 = Unbundle By Name(w454) -> ("App Config.Cycle Threshold:"=w452:dbl)
              n152 = Not Equal?(x=w452, y="Cycle Threshold:") -> (x != y?=w453:bool)
              n153 = Bundle By Name(cluster=w456, "App Config.Cycle Threshold:"="Cycle Threshold:") -> (w455:T26)
            }
            frame 50 {
              w464 = T15[] [enum."Save App Config"] items=["Main", "Init Files", "Init", "Unused", "Save As", "Start Profile", "Check Step Time", "Alarm", "Alarm Dismiss", "Run Step", "Stop Profile", "Cycle Reset", "Time Reset", "Time Reset All", "Time Set", "Tare CTs", "Save Profile", "Open Profile", "Get Profiles", "Update Screen", "Update Controls", "Save App Config", "Write Outputs", "Disable Background", "Enable Background", "Get/Release Control", "Log Fuel Change", "Fuel Change Popup", "Read Inputs", "Remote Timer Reset", "Controller Change", "Get Alarms", "Init Alarms", "Save Alarms", "Voltage Selection", "Set Watlow Temp 1", "Set Watlow Temp 2", "Get Pressure", "Write Tare Pressure", "Adjust Controls", "Reinit ADC", "Write Initial Times", "Write Pumps Present", "HMI Command", "Save Pump Times", "Check Pump Stop Time", "Save LS App Config", "Init Data File", "Reset LS Cycles", "Reset Anomalies", "Reset Opens", "Save LS Data", "Save LS Test Data", "Check Serial Numbers", "Main Tab", "Allow Data Note"]
              n154 = Unbundle By Name(w461) -> ("App Config.Cycle Pts to Avg:"=w459:i32)
              n155 = Not Equal?(x=w459, y="Cycle Pts to Avg:") -> (x != y?=w460:bool)
              n156 = Bundle By Name(cluster=w463, "App Config.Cycle Pts to Avg:"="Cycle Pts to Avg:") -> (w462:T26)
            }
            frame 51 {
              w471 = T15[] [enum."Save App Config", enum."Write Outputs"] items=["Main", "Init Files", "Init", "Unused", "Save As", "Start Profile", "Check Step Time", "Alarm", "Alarm Dismiss", "Run Step", "Stop Profile", "Cycle Reset", "Time Reset", "Time Reset All", "Time Set", "Tare CTs", "Save Profile", "Open Profile", "Get Profiles", "Update Screen", "Update Controls", "Save App Config", "Write Outputs", "Disable Background", "Enable Background", "Get/Release Control", "Log Fuel Change", "Fuel Change Popup", "Read Inputs", "Remote Timer Reset", "Controller Change", "Get Alarms", "Init Alarms", "Save Alarms", "Voltage Selection", "Set Watlow Temp 1", "Set Watlow Temp 2", "Get Pressure", "Write Tare Pressure", "Adjust Controls", "Reinit ADC", "Write Initial Times", "Write Pumps Present", "HMI Command", "Save Pump Times", "Check Pump Stop Time", "Save LS App Config", "Init Data File", "Reset LS Cycles", "Reset Anomalies", "Reset Opens", "Save LS Data", "Save LS Test Data", "Check Serial Numbers", "Main Tab", "Allow Data Note"]
              n157 = Unbundle By Name(w468) -> ("App Config.Step Threshold:"=w466:dbl)
              n158 = Not Equal?(x=w466, y="Step Threshold:") -> (x != y?=w467:bool)
              n159 = Bundle By Name(cluster=w470, "App Config.Step Threshold:"="Step Threshold:") -> (w469:T26)
            }
            frame 52 {
              w478 = T15[] [enum."Save App Config", enum."Write Outputs"] items=["Main", "Init Files", "Init", "Unused", "Save As", "Start Profile", "Check Step Time", "Alarm", "Alarm Dismiss", "Run Step", "Stop Profile", "Cycle Reset", "Time Reset", "Time Reset All", "Time Set", "Tare CTs", "Save Profile", "Open Profile", "Get Profiles", "Update Screen", "Update Controls", "Save App Config", "Write Outputs", "Disable Background", "Enable Background", "Get/Release Control", "Log Fuel Change", "Fuel Change Popup", "Read Inputs", "Remote Timer Reset", "Controller Change", "Get Alarms", "Init Alarms", "Save Alarms", "Voltage Selection", "Set Watlow Temp 1", "Set Watlow Temp 2", "Get Pressure", "Write Tare Pressure", "Adjust Controls", "Reinit ADC", "Write Initial Times", "Write Pumps Present", "HMI Command", "Save Pump Times", "Check Pump Stop Time", "Save LS App Config", "Init Data File", "Reset LS Cycles", "Reset Anomalies", "Reset Opens", "Save LS Data", "Save LS Test Data", "Check Serial Numbers", "Main Tab", "Allow Data Note"]
              n160 = Unbundle By Name(w475) -> ("App Config.Normal Steps:"=w473:u32)
              n161 = Not Equal?(x=w473, y="Normal Steps:") -> (x != y?=w474:bool)
              n162 = Bundle By Name(cluster=w477, "App Config.Normal Steps:"="Normal Steps:") -> (w476:T26)
            }
            frame 53 {
              w487 = T15[] [enum."Main Tab"] items=["Main", "Init Files", "Init", "Unused", "Save As", "Start Profile", "Check Step Time", "Alarm", "Alarm Dismiss", "Run Step", "Stop Profile", "Cycle Reset", "Time Reset", "Time Reset All", "Time Set", "Tare CTs", "Save Profile", "Open Profile", "Get Profiles", "Update Screen", "Update Controls", "Save App Config", "Write Outputs", "Disable Background", "Enable Background", "Get/Release Control", "Log Fuel Change", "Fuel Change Popup", "Read Inputs", "Remote Timer Reset", "Controller Change", "Get Alarms", "Init Alarms", "Save Alarms", "Voltage Selection", "Set Watlow Temp 1", "Set Watlow Temp 2", "Get Pressure", "Write Tare Pressure", "Adjust Controls", "Reinit ADC", "Write Initial Times", "Write Pumps Present", "HMI Command", "Save Pump Times", "Check Pump Stop Time", "Save LS App Config", "Init Data File", "Reset LS Cycles", "Reset Anomalies", "Reset Opens", "Save LS Data", "Save LS Test Data", "Check Serial Numbers", "Main Tab", "Allow Data Note"]
              n163 = Unbundle By Name(w492) -> ("Main Tab"=w489:T9)
              n164 = local read "Main Tab"() -> (w488:T9)
              n165 = local read "Position"() -> (w481:i32)
              n166 = local read "Pause"() -> (w483:bool)
              n167 = feedback-in #1(w481) -> ()
              n168 = feedback #1(w481) -> (w482:i32)
              n169 = feedback #2(w483) -> (w484:bool)
              n170 = feedback-in #2(w483) -> ()
              n171 = Not Equal?(x=w489, y=w488) -> (x != y?=w486:bool)
              n172 = Not Equal?(x=w482, y=w481) -> (x != y?=w480:bool)
              n173 = Greater?(x=w484, y=w483) -> (0:w479:bool)
              n174 = Compound Arithmetic op=OR(w486, w480, w479) -> (w485:bool)
              n175 = case shown="True" w485 {
                frame False {
                }
                frame True {
                  n176 = property on="Waveform Chart" class="WFChart (strict)"("History Data"=dbl[] []) -> ()  [unwired: 2 in, 2 out]
                }
              }
              n177 = Bundle By Name(cluster=w491, "Main Tab"=w488) -> (w490:T26)
            }
            frame 54 {
              w497 = T15[] [enum."Save LS App Config", enum."Write Outputs"] items=["Main", "Init Files", "Init", "Unused", "Save As", "Start Profile", "Check Step Time", "Alarm", "Alarm Dismiss", "Run Step", "Stop Profile", "Cycle Reset", "Time Reset", "Time Reset All", "Time Set", "Tare CTs", "Save Profile", "Open Profile", "Get Profiles", "Update Screen", "Update Controls", "Save App Config", "Write Outputs", "Disable Background", "Enable Background", "Get/Release Control", "Log Fuel Change", "Fuel Change Popup", "Read Inputs", "Remote Timer Reset", "Controller Change", "Get Alarms", "Init Alarms", "Save Alarms", "Voltage Selection", "Set Watlow Temp 1", "Set Watlow Temp 2", "Get Pressure", "Write Tare Pressure", "Adjust Controls", "Reinit ADC", "Write Initial Times", "Write Pumps Present", "HMI Command", "Save Pump Times", "Check Pump Stop Time", "Save LS App Config", "Init Data File", "Reset LS Cycles", "Reset Anomalies", "Reset Opens", "Save LS Data", "Save LS Test Data", "Check Serial Numbers", "Main Tab", "Allow Data Note"]
              n178 = Unbundle By Name(w500) -> ("LS App Config.LS Power (Freq):"=w496:dbl)
              n179 = Not Equal?(x=w496, y="LS Power (Freq):") -> (x != y?=w494:bool)
              n180 = Bundle By Name(cluster=w499, "LS App Config.LS Power (Freq):"="LS Power (Freq):") -> (w498:T26)
            }
            frame 55 {
              w504 = T15[] [enum."Save LS App Config", enum."Write Outputs"] items=["Main", "Init Files", "Init", "Unused", "Save As", "Start Profile", "Check Step Time", "Alarm", "Alarm Dismiss", "Run Step", "Stop Profile", "Cycle Reset", "Time Reset", "Time Reset All", "Time Set", "Tare CTs", "Save Profile", "Open Profile", "Get Profiles", "Update Screen", "Update Controls", "Save App Config", "Write Outputs", "Disable Background", "Enable Background", "Get/Release Control", "Log Fuel Change", "Fuel Change Popup", "Read Inputs", "Remote Timer Reset", "Controller Change", "Get Alarms", "Init Alarms", "Save Alarms", "Voltage Selection", "Set Watlow Temp 1", "Set Watlow Temp 2", "Get Pressure", "Write Tare Pressure", "Adjust Controls", "Reinit ADC", "Write Initial Times", "Write Pumps Present", "HMI Command", "Save Pump Times", "Check Pump Stop Time", "Save LS App Config", "Init Data File", "Reset LS Cycles", "Reset Anomalies", "Reset Opens", "Save LS Data", "Save LS Test Data", "Check Serial Numbers", "Main Tab", "Allow Data Note"]
              n181 = Unbundle By Name(w507) -> ("LS App Config.LS Power (Duty):"=w503:dbl)
              n182 = Not Equal?(x=w503, y="LS Power (Duty):") -> (x != y?=w502:bool)
              n183 = Bundle By Name(cluster=w506, "LS App Config.LS Power (Duty):"="LS Power (Duty):") -> (w505:T26)
            }
            frame 56 {
              w513 = T15[] [enum."Save LS App Config", enum."Write Outputs"] items=["Main", "Init Files", "Init", "Unused", "Save As", "Start Profile", "Check Step Time", "Alarm", "Alarm Dismiss", "Run Step", "Stop Profile", "Cycle Reset", "Time Reset", "Time Reset All", "Time Set", "Tare CTs", "Save Profile", "Open Profile", "Get Profiles", "Update Screen", "Update Controls", "Save App Config", "Write Outputs", "Disable Background", "Enable Background", "Get/Release Control", "Log Fuel Change", "Fuel Change Popup", "Read Inputs", "Remote Timer Reset", "Controller Change", "Get Alarms", "Init Alarms", "Save Alarms", "Voltage Selection", "Set Watlow Temp 1", "Set Watlow Temp 2", "Get Pressure", "Write Tare Pressure", "Adjust Controls", "Reinit ADC", "Write Initial Times", "Write Pumps Present", "HMI Command", "Save Pump Times", "Check Pump Stop Time", "Save LS App Config", "Init Data File", "Reset LS Cycles", "Reset Anomalies", "Reset Opens", "Save LS Data", "Save LS Test Data", "Check Serial Numbers", "Main Tab", "Allow Data Note"]
              n184 = Unbundle By Name(w516) -> ("LS App Config.Bank 1 Present"=w512:T2)
              n185 = Not Equal?(x=w512, y="Bank 1") -> (x != y?=w510:T2)
              n186 = Cluster To Array(cluster=w510) -> (array=w509:bool[])
              n187 = Or Array Elements(Boolean array=w509) -> (logical OR=w508:bool)
              n188 = Bundle By Name(cluster=w515, "LS App Config.Bank 1 Present"="Bank 1") -> (w514:T26)
            }
            frame 57 {
              w522 = T15[] [enum."Save LS App Config", enum."Write Outputs"] items=["Main", "Init Files", "Init", "Unused", "Save As", "Start Profile", "Check Step Time", "Alarm", "Alarm Dismiss", "Run Step", "Stop Profile", "Cycle Reset", "Time Reset", "Time Reset All", "Time Set", "Tare CTs", "Save Profile", "Open Profile", "Get Profiles", "Update Screen", "Update Controls", "Save App Config", "Write Outputs", "Disable Background", "Enable Background", "Get/Release Control", "Log Fuel Change", "Fuel Change Popup", "Read Inputs", "Remote Timer Reset", "Controller Change", "Get Alarms", "Init Alarms", "Save Alarms", "Voltage Selection", "Set Watlow Temp 1", "Set Watlow Temp 2", "Get Pressure", "Write Tare Pressure", "Adjust Controls", "Reinit ADC", "Write Initial Times", "Write Pumps Present", "HMI Command", "Save Pump Times", "Check Pump Stop Time", "Save LS App Config", "Init Data File", "Reset LS Cycles", "Reset Anomalies", "Reset Opens", "Save LS Data", "Save LS Test Data", "Check Serial Numbers", "Main Tab", "Allow Data Note"]
              n189 = Unbundle By Name(w525) -> ("LS App Config.Bank 2 Present"=w521:T1)
              n190 = Not Equal?(x=w521, y="Bank 2") -> (x != y?=w520:T1)
              n191 = Cluster To Array(cluster=w520) -> (array=w519:bool[])
              n192 = Or Array Elements(Boolean array=w519) -> (logical OR=w518:bool)
              n193 = Bundle By Name(cluster=w524, "LS App Config.Bank 2 Present"="Bank 2") -> (w523:T26)
            }
            frame 58 {
              w529 = T15[] [enum."Init Data File", enum."Save LS App Config"] items=["Main", "Init Files", "Init", "Unused", "Save As", "Start Profile", "Check Step Time", "Alarm", "Alarm Dismiss", "Run Step", "Stop Profile", "Cycle Reset", "Time Reset", "Time Reset All", "Time Set", "Tare CTs", "Save Profile", "Open Profile", "Get Profiles", "Update Screen", "Update Controls", "Save App Config", "Write Outputs", "Disable Background", "Enable Background", "Get/Release Control", "Log Fuel Change", "Fuel Change Popup", "Read Inputs", "Remote Timer Reset", "Controller Change", "Get Alarms", "Init Alarms", "Save Alarms", "Voltage Selection", "Set Watlow Temp 1", "Set Watlow Temp 2", "Get Pressure", "Write Tare Pressure", "Adjust Controls", "Reinit ADC", "Write Initial Times", "Write Pumps Present", "HMI Command", "Save Pump Times", "Check Pump Stop Time", "Save LS App Config", "Init Data File", "Reset LS Cycles", "Reset Anomalies", "Reset Opens", "Save LS Data", "Save LS Test Data", "Check Serial Numbers", "Main Tab", "Allow Data Note"]
              n194 = Unbundle By Name(w532) -> ("LS App Config.Data File Name:"=w528:string)
              n195 = Not Equal?(x=w528, y="Data File Name:") -> (x != y?=w527:bool)
              n196 = Bundle By Name(cluster=w531, "LS App Config.Data File Name:"="Data File Name:") -> (w530:T26)
            }
            frame 59 {
              w536 = T15[] [enum."Save LS App Config"] items=["Main", "Init Files", "Init", "Unused", "Save As", "Start Profile", "Check Step Time", "Alarm", "Alarm Dismiss", "Run Step", "Stop Profile", "Cycle Reset", "Time Reset", "Time Reset All", "Time Set", "Tare CTs", "Save Profile", "Open Profile", "Get Profiles", "Update Screen", "Update Controls", "Save App Config", "Write Outputs", "Disable Background", "Enable Background", "Get/Release Control", "Log Fuel Change", "Fuel Change Popup", "Read Inputs", "Remote Timer Reset", "Controller Change", "Get Alarms", "Init Alarms", "Save Alarms", "Voltage Selection", "Set Watlow Temp 1", "Set Watlow Temp 2", "Get Pressure", "Write Tare Pressure", "Adjust Controls", "Reinit ADC", "Write Initial Times", "Write Pumps Present", "HMI Command", "Save Pump Times", "Check Pump Stop Time", "Save LS App Config", "Init Data File", "Reset LS Cycles", "Reset Anomalies", "Reset Opens", "Save LS Data", "Save LS Test Data", "Check Serial Numbers", "Main Tab", "Allow Data Note"]
              n197 = Unbundle By Name(w539) -> ("LS App Config.Record Bursts"=w535:bool)
              n198 = Not Equal?(x=w535, y="Record During Profile") -> (x != y?=w534:bool)
              n199 = Bundle By Name(cluster=w538, "LS App Config.Record Bursts"="Record During Profile") -> (w537:T26)
            }
            frame 60 {
              w543 = T15[] [enum."Save LS App Config"] items=["Main", "Init Files", "Init", "Unused", "Save As", "Start Profile", "Check Step Time", "Alarm", "Alarm Dismiss", "Run Step", "Stop Profile", "Cycle Reset", "Time Reset", "Time Reset All", "Time Set", "Tare CTs", "Save Profile", "Open Profile", "Get Profiles", "Update Screen", "Update Controls", "Save App Config", "Write Outputs", "Disable Background", "Enable Background", "Get/Release Control", "Log Fuel Change", "Fuel Change Popup", "Read Inputs", "Remote Timer Reset", "Controller Change", "Get Alarms", "Init Alarms", "Save Alarms", "Voltage Selection", "Set Watlow Temp 1", "Set Watlow Temp 2", "Get Pressure", "Write Tare Pressure", "Adjust Controls", "Reinit ADC", "Write Initial Times", "Write Pumps Present", "HMI Command", "Save Pump Times", "Check Pump Stop Time", "Save LS App Config", "Init Data File", "Reset LS Cycles", "Reset Anomalies", "Reset Opens", "Save LS Data", "Save LS Test Data", "Check Serial Numbers", "Main Tab", "Allow Data Note"]
              n200 = Unbundle By Name(w546) -> ("LS App Config.RecInterval(s)"=w542:i32)
              n201 = Not Equal?(x=w542, y="Interval Between\nRecordings (s):") -> (x != y?=w541:bool)
              n202 = Bundle By Name(cluster=w545, "LS App Config.RecInterval(s)"="Interval Between\nRecordings (s):") -> (w544:T26)
            }
            frame 61 {
              w550 = T15[] [enum."Save LS App Config"] items=["Main", "Init Files", "Init", "Unused", "Save As", "Start Profile", "Check Step Time", "Alarm", "Alarm Dismiss", "Run Step", "Stop Profile", "Cycle Reset", "Time Reset", "Time Reset All", "Time Set", "Tare CTs", "Save Profile", "Open Profile", "Get Profiles", "Update Screen", "Update Controls", "Save App Config", "Write Outputs", "Disable Background", "Enable Background", "Get/Release Control", "Log Fuel Change", "Fuel Change Popup", "Read Inputs", "Remote Timer Reset", "Controller Change", "Get Alarms", "Init Alarms", "Save Alarms", "Voltage Selection", "Set Watlow Temp 1", "Set Watlow Temp 2", "Get Pressure", "Write Tare Pressure", "Adjust Controls", "Reinit ADC", "Write Initial Times", "Write Pumps Present", "HMI Command", "Save Pump Times", "Check Pump Stop Time", "Save LS App Config", "Init Data File", "Reset LS Cycles", "Reset Anomalies", "Reset Opens", "Save LS Data", "Save LS Test Data", "Check Serial Numbers", "Main Tab", "Allow Data Note"]
              n203 = Unbundle By Name(w553) -> ("LS App Config.RecDuration(s)"=w549:i32)
              n204 = Not Equal?(x=w549, y="Recording\nDuration (s):") -> (x != y?=w548:bool)
              n205 = Bundle By Name(cluster=w552, "LS App Config.RecDuration(s)"="Recording\nDuration (s):") -> (w551:T26)
            }
            frame 62 {
              w557 = T15[] [enum."Save LS App Config"] items=["Main", "Init Files", "Init", "Unused", "Save As", "Start Profile", "Check Step Time", "Alarm", "Alarm Dismiss", "Run Step", "Stop Profile", "Cycle Reset", "Time Reset", "Time Reset All", "Time Set", "Tare CTs", "Save Profile", "Open Profile", "Get Profiles", "Update Screen", "Update Controls", "Save App Config", "Write Outputs", "Disable Background", "Enable Background", "Get/Release Control", "Log Fuel Change", "Fuel Change Popup", "Read Inputs", "Remote Timer Reset", "Controller Change", "Get Alarms", "Init Alarms", "Save Alarms", "Voltage Selection", "Set Watlow Temp 1", "Set Watlow Temp 2", "Get Pressure", "Write Tare Pressure", "Adjust Controls", "Reinit ADC", "Write Initial Times", "Write Pumps Present", "HMI Command", "Save Pump Times", "Check Pump Stop Time", "Save LS App Config", "Init Data File", "Reset LS Cycles", "Reset Anomalies", "Reset Opens", "Save LS Data", "Save LS Test Data", "Check Serial Numbers", "Main Tab", "Allow Data Note"]
              n206 = Unbundle By Name(w560) -> ("LS App Config.RecFrequeny (Hz)"=w556:i32)
              n207 = Not Equal?(x=w556, y="Recording\nFrequency (Hz):") -> (x != y?=w555:bool)
              n208 = Bundle By Name(cluster=w559, "LS App Config.RecFrequeny (Hz)"="Recording\nFrequency (Hz):") -> (w558:T26)
            }
            frame 63 {
              w564 = T15[] [enum."Save LS App Config", enum."Write Outputs"] items=["Main", "Init Files", "Init", "Unused", "Save As", "Start Profile", "Check Step Time", "Alarm", "Alarm Dismiss", "Run Step", "Stop Profile", "Cycle Reset", "Time Reset", "Time Reset All", "Time Set", "Tare CTs", "Save Profile", "Open Profile", "Get Profiles", "Update Screen", "Update Controls", "Save App Config", "Write Outputs", "Disable Background", "Enable Background", "Get/Release Control", "Log Fuel Change", "Fuel Change Popup", "Read Inputs", "Remote Timer Reset", "Controller Change", "Get Alarms", "Init Alarms", "Save Alarms", "Voltage Selection", "Set Watlow Temp 1", "Set Watlow Temp 2", "Get Pressure", "Write Tare Pressure", "Adjust Controls", "Reinit ADC", "Write Initial Times", "Write Pumps Present", "HMI Command", "Save Pump Times", "Check Pump Stop Time", "Save LS App Config", "Init Data File", "Reset LS Cycles", "Reset Anomalies", "Reset Opens", "Save LS Data", "Save LS Test Data", "Check Serial Numbers", "Main Tab", "Allow Data Note"]
              # "Notice"
              n209 = disable-structure shown="Enabled" {
                disable-tunnel: ["Detection Mode:" u16 1 ("Detection Mode:")] -> w561
                frame Disabled {
                }
                frame Enabled {
                }
              }
              n210 = Unbundle By Name(w567) -> ("LS App Config.DetectionMode"=w563:i32)
              n211 = Not Equal?(x=w563, y=w561) -> (x != y?=w562:bool)
              n212 = case shown="True" w562 {
                tunnel: w561 -> [_ w570]
                frame False {
                }
                frame True {
                  n213 = case shown="1" w570 {
                    frame 0, Default {
                      n214 = local write "Live Data Tab"(enum32{"Page 1", "Page 2", "Page 3"}."Page 2" ("Live Data Tab")) -> ()
                    }
                    frame 1 {
                      n215 = local write "Live Data Tab"(enum32{"Page 1", "Page 2", "Page 3"}."Page 3" ("Live Data Tab")) -> ()
                    }
                  }
                }
              }
              n216 = Bundle By Name(cluster=w566, "LS App Config.DetectionMode"=w561) -> (w565:T26)
            }
            frame 64 {
              w578 = T15[] [enum."Check Serial Numbers", enum."Save LS App Config"] items=["Main", "Init Files", "Init", "Unused", "Save As", "Start Profile", "Check Step Time", "Alarm", "Alarm Dismiss", "Run Step", "Stop Profile", "Cycle Reset", "Time Reset", "Time Reset All", "Time Set", "Tare CTs", "Save Profile", "Open Profile", "Get Profiles", "Update Screen", "Update Controls", "Save App Config", "Write Outputs", "Disable Background", "Enable Background", "Get/Release Control", "Log Fuel Change", "Fuel Change Popup", "Read Inputs", "Remote Timer Reset", "Controller Change", "Get Alarms", "Init Alarms", "Save Alarms", "Voltage Selection", "Set Watlow Temp 1", "Set Watlow Temp 2", "Get Pressure", "Write Tare Pressure", "Adjust Controls", "Reinit ADC", "Write Initial Times", "Write Pumps Present", "HMI Command", "Save Pump Times", "Check Pump Stop Time", "Save LS App Config", "Init Data File", "Reset LS Cycles", "Reset Anomalies", "Reset Opens", "Save LS Data", "Save LS Test Data", "Check Serial Numbers", "Main Tab", "Allow Data Note"]
              n217 = Unbundle By Name(w581) -> ("LS App Config.Serial Numbers"=w577:string[])
              n218 = Cluster To Array(cluster="LS Serial Numbers") -> (array=w575:string[])
              n219 = Not Equal?(x=w577, y=w575) -> (x != y?=w574:bool[])
              n220 = Or Array Elements(Boolean array=w574) -> (logical OR=w573:bool)
              n221 = Bundle By Name(cluster=w580, "LS App Config.Serial Numbers"=w575) -> (w579:T26)
            }
            frame 65 {
              w585 = T15[] [enum."Write Outputs"] items=["Main", "Init Files", "Init", "Unused", "Save As", "Start Profile", "Check Step Time", "Alarm", "Alarm Dismiss", "Run Step", "Stop Profile", "Cycle Reset", "Time Reset", "Time Reset All", "Time Set", "Tare CTs", "Save Profile", "Open Profile", "Get Profiles", "Update Screen", "Update Controls", "Save App Config", "Write Outputs", "Disable Background", "Enable Background", "Get/Release Control", "Log Fuel Change", "Fuel Change Popup", "Read Inputs", "Remote Timer Reset", "Controller Change", "Get Alarms", "Init Alarms", "Save Alarms", "Voltage Selection", "Set Watlow Temp 1", "Set Watlow Temp 2", "Get Pressure", "Write Tare Pressure", "Adjust Controls", "Reinit ADC", "Write Initial Times", "Write Pumps Present", "HMI Command", "Save Pump Times", "Check Pump Stop Time", "Save LS App Config", "Init Data File", "Reset LS Cycles", "Reset Anomalies", "Reset Opens", "Save LS Data", "Save LS Test Data", "Check Serial Numbers", "Main Tab", "Allow Data Note"]
              n222 = Unbundle By Name(w588) -> ("Bank 1 State:"=w584:u16)
              n223 = Not Equal?(x=w584, y="Bank 1 Power State:") -> (x != y?=w582:bool)
              n224 = Bundle By Name(cluster=w587, "Bank 1 State:"="Bank 1 Power State:") -> (w586:T26)
            }
            frame 66 {
              w592 = T15[] [enum."Write Outputs"] items=["Main", "Init Files", "Init", "Unused", "Save As", "Start Profile", "Check Step Time", "Alarm", "Alarm Dismiss", "Run Step", "Stop Profile", "Cycle Reset", "Time Reset", "Time Reset All", "Time Set", "Tare CTs", "Save Profile", "Open Profile", "Get Profiles", "Update Screen", "Update Controls", "Save App Config", "Write Outputs", "Disable Background", "Enable Background", "Get/Release Control", "Log Fuel Change", "Fuel Change Popup", "Read Inputs", "Remote Timer Reset", "Controller Change", "Get Alarms", "Init Alarms", "Save Alarms", "Voltage Selection", "Set Watlow Temp 1", "Set Watlow Temp 2", "Get Pressure", "Write Tare Pressure", "Adjust Controls", "Reinit ADC", "Write Initial Times", "Write Pumps Present", "HMI Command", "Save Pump Times", "Check Pump Stop Time", "Save LS App Config", "Init Data File", "Reset LS Cycles", "Reset Anomalies", "Reset Opens", "Save LS Data", "Save LS Test Data", "Check Serial Numbers", "Main Tab", "Allow Data Note"]
              n225 = Unbundle By Name(w595) -> ("Bank 2 State:"=w591:u16)
              n226 = Not Equal?(x=w591, y="Bank 2 Power State:") -> (x != y?=w590:bool)
              n227 = Bundle By Name(cluster=w594, "Bank 2 State:"="Bank 2 Power State:") -> (w593:T26)
            }
            frame 67 {
              w598 = T15[] [enum."Reset LS Cycles"] items=["Main", "Init Files", "Init", "Unused", "Save As", "Start Profile", "Check Step Time", "Alarm", "Alarm Dismiss", "Run Step", "Stop Profile", "Cycle Reset", "Time Reset", "Time Reset All", "Time Set", "Tare CTs", "Save Profile", "Open Profile", "Get Profiles", "Update Screen", "Update Controls", "Save App Config", "Write Outputs", "Disable Background", "Enable Background", "Get/Release Control", "Log Fuel Change", "Fuel Change Popup", "Read Inputs", "Remote Timer Reset", "Controller Change", "Get Alarms", "Init Alarms", "Save Alarms", "Voltage Selection", "Set Watlow Temp 1", "Set Watlow Temp 2", "Get Pressure", "Write Tare Pressure", "Adjust Controls", "Reinit ADC", "Write Initial Times", "Write Pumps Present", "HMI Command", "Save Pump Times", "Check Pump Stop Time", "Save LS App Config", "Init Data File", "Reset LS Cycles", "Reset Anomalies", "Reset Opens", "Save LS Data", "Save LS Test Data", "Check Serial Numbers", "Main Tab", "Allow Data Note"]
            }
            frame 68 {
              w601 = T15[] [enum."Reset Anomalies"] items=["Main", "Init Files", "Init", "Unused", "Save As", "Start Profile", "Check Step Time", "Alarm", "Alarm Dismiss", "Run Step", "Stop Profile", "Cycle Reset", "Time Reset", "Time Reset All", "Time Set", "Tare CTs", "Save Profile", "Open Profile", "Get Profiles", "Update Screen", "Update Controls", "Save App Config", "Write Outputs", "Disable Background", "Enable Background", "Get/Release Control", "Log Fuel Change", "Fuel Change Popup", "Read Inputs", "Remote Timer Reset", "Controller Change", "Get Alarms", "Init Alarms", "Save Alarms", "Voltage Selection", "Set Watlow Temp 1", "Set Watlow Temp 2", "Get Pressure", "Write Tare Pressure", "Adjust Controls", "Reinit ADC", "Write Initial Times", "Write Pumps Present", "HMI Command", "Save Pump Times", "Check Pump Stop Time", "Save LS App Config", "Init Data File", "Reset LS Cycles", "Reset Anomalies", "Reset Opens", "Save LS Data", "Save LS Test Data", "Check Serial Numbers", "Main Tab", "Allow Data Note"]
            }
            frame 69 {
              w604 = T15[] [enum."Reset Opens"] items=["Main", "Init Files", "Init", "Unused", "Save As", "Start Profile", "Check Step Time", "Alarm", "Alarm Dismiss", "Run Step", "Stop Profile", "Cycle Reset", "Time Reset", "Time Reset All", "Time Set", "Tare CTs", "Save Profile", "Open Profile", "Get Profiles", "Update Screen", "Update Controls", "Save App Config", "Write Outputs", "Disable Background", "Enable Background", "Get/Release Control", "Log Fuel Change", "Fuel Change Popup", "Read Inputs", "Remote Timer Reset", "Controller Change", "Get Alarms", "Init Alarms", "Save Alarms", "Voltage Selection", "Set Watlow Temp 1", "Set Watlow Temp 2", "Get Pressure", "Write Tare Pressure", "Adjust Controls", "Reinit ADC", "Write Initial Times", "Write Pumps Present", "HMI Command", "Save Pump Times", "Check Pump Stop Time", "Save LS App Config", "Init Data File", "Reset LS Cycles", "Reset Anomalies", "Reset Opens", "Save LS Data", "Save LS Test Data", "Check Serial Numbers", "Main Tab", "Allow Data Note"]
            }
            frame 70 {
              w606 = T15[] [enum."Init Data File", enum."Save LS App Config"] items=["Main", "Init Files", "Init", "Unused", "Save As", "Start Profile", "Check Step Time", "Alarm", "Alarm Dismiss", "Run Step", "Stop Profile", "Cycle Reset", "Time Reset", "Time Reset All", "Time Set", "Tare CTs", "Save Profile", "Open Profile", "Get Profiles", "Update Screen", "Update Controls", "Save App Config", "Write Outputs", "Disable Background", "Enable Background", "Get/Release Control", "Log Fuel Change", "Fuel Change Popup", "Read Inputs", "Remote Timer Reset", "Controller Change", "Get Alarms", "Init Alarms", "Save Alarms", "Voltage Selection", "Set Watlow Temp 1", "Set Watlow Temp 2", "Get Pressure", "Write Tare Pressure", "Adjust Controls", "Reinit ADC", "Write Initial Times", "Write Pumps Present", "HMI Command", "Save Pump Times", "Check Pump Stop Time", "Save LS App Config", "Init Data File", "Reset LS Cycles", "Reset Anomalies", "Reset Opens", "Save LS Data", "Save LS Test Data", "Check Serial Numbers", "Main Tab", "Allow Data Note"]
              n228 = Unbundle By Name(w609) -> ("day of month"=w608:i32)
              n229 = Get Date/Time In Seconds() -> (seconds since 1Jan1904=w612:timestamp)
              n230 = Seconds To Date/Time(time stamp (now)=w612) -> (date time rec=w613:T46)  [unwired: 1 in]
              n231 = Unbundle By Name(w613) -> ("day of month"=w605:i32)
              n232 = Not Equal?(x=w608, y=w605) -> (x != y?=w607:bool)
              n233 = Bundle By Name(cluster=w611, "day of month"=w605) -> (w610:T26)
            }
            frame 71 {
              w614 = T15[] [enum."Save App Config", enum."Write Outputs"] items=["Main", "Init Files", "Init", "Unused", "Save As", "Start Profile", "Check Step Time", "Alarm", "Alarm Dismiss", "Run Step", "Stop Profile", "Cycle Reset", "Time Reset", "Time Reset All", "Time Set", "Tare CTs", "Save Profile", "Open Profile", "Get Profiles", "Update Screen", "Update Controls", "Save App Config", "Write Outputs", "Disable Background", "Enable Background", "Get/Release Control", "Log Fuel Change", "Fuel Change Popup", "Read Inputs", "Remote Timer Reset", "Controller Change", "Get Alarms", "Init Alarms", "Save Alarms", "Voltage Selection", "Set Watlow Temp 1", "Set Watlow Temp 2", "Get Pressure", "Write Tare Pressure", "Adjust Controls", "Reinit ADC", "Write Initial Times", "Write Pumps Present", "HMI Command", "Save Pump Times", "Check Pump Stop Time", "Save LS App Config", "Init Data File", "Reset LS Cycles", "Reset Anomalies", "Reset Opens", "Save LS Data", "Save LS Test Data", "Check Serial Numbers", "Main Tab", "Allow Data Note"]
              n234 = Unbundle By Name(w619) -> ("App Config.Anomaly Threshold:"=w620:dbl)
              n235 = Not Equal?(x=w620, y="Anomaly Threshold:") -> (x != y?=w616:bool)
              n236 = Bundle By Name(cluster=w618, "App Config.Anomaly Threshold:"="Anomaly Threshold:") -> (w617:T26)
            }
            frame 72 {
              w621 = T15[] [enum."Save LS App Config"] items=["Main", "Init Files", "Init", "Unused", "Save As", "Start Profile", "Check Step Time", "Alarm", "Alarm Dismiss", "Run Step", "Stop Profile", "Cycle Reset", "Time Reset", "Time Reset All", "Time Set", "Tare CTs", "Save Profile", "Open Profile", "Get Profiles", "Update Screen", "Update Controls", "Save App Config", "Write Outputs", "Disable Background", "Enable Background", "Get/Release Control", "Log Fuel Change", "Fuel Change Popup", "Read Inputs", "Remote Timer Reset", "Controller Change", "Get Alarms", "Init Alarms", "Save Alarms", "Voltage Selection", "Set Watlow Temp 1", "Set Watlow Temp 2", "Get Pressure", "Write Tare Pressure", "Adjust Controls", "Reinit ADC", "Write Initial Times", "Write Pumps Present", "HMI Command", "Save Pump Times", "Check Pump Stop Time", "Save LS App Config", "Init Data File", "Reset LS Cycles", "Reset Anomalies", "Reset Opens", "Save LS Data", "Save LS Test Data", "Check Serial Numbers", "Main Tab", "Allow Data Note"]
              n237 = Unbundle By Name(w626) -> ("LS App Config.Record Constant"=w627:bool)
              n238 = Not Equal?(x=w627, y="Record Constant") -> (x != y?=w623:bool)
              n239 = Bundle By Name(cluster=w625, "LS App Config.Record Constant"="Record Constant") -> (w624:T26)
            }
            frame 73 {
              w629 = T15[] [] items=["Main", "Init Files", "Init", "Unused", "Save As", "Start Profile", "Check Step Time", "Alarm", "Alarm Dismiss", "Run Step", "Stop Profile", "Cycle Reset", "Time Reset", "Time Reset All", "Time Set", "Tare CTs", "Save Profile", "Open Profile", "Get Profiles", "Update Screen", "Update Controls", "Save App Config", "Write Outputs", "Disable Background", "Enable Background", "Get/Release Control", "Log Fuel Change", "Fuel Change Popup", "Read Inputs", "Remote Timer Reset", "Controller Change", "Get Alarms", "Init Alarms", "Save Alarms", "Voltage Selection", "Set Watlow Temp 1", "Set Watlow Temp 2", "Get Pressure", "Write Tare Pressure", "Adjust Controls", "Reinit ADC", "Write Initial Times", "Write Pumps Present", "HMI Command", "Save Pump Times", "Check Pump Stop Time", "Save LS App Config", "Init Data File", "Reset LS Cycles", "Reset Anomalies", "Reset Opens", "Save LS Data", "Save LS Test Data", "Check Serial Numbers", "Main Tab", "Allow Data Note"]
              n240 = call "LS Data Global.vi"() -> ("Recording Out"=→"Recording":bool)  [unwired: 14 in, 1 out]
            }
            frame 74 {
              w632 = T15[] [enum."Save LS App Config", enum."Write Outputs"] items=["Main", "Init Files", "Init", "Unused", "Save As", "Start Profile", "Check Step Time", "Alarm", "Alarm Dismiss", "Run Step", "Stop Profile", "Cycle Reset", "Time Reset", "Time Reset All", "Time Set", "Tare CTs", "Save Profile", "Open Profile", "Get Profiles", "Update Screen", "Update Controls", "Save App Config", "Write Outputs", "Disable Background", "Enable Background", "Get/Release Control", "Log Fuel Change", "Fuel Change Popup", "Read Inputs", "Remote Timer Reset", "Controller Change", "Get Alarms", "Init Alarms", "Save Alarms", "Voltage Selection", "Set Watlow Temp 1", "Set Watlow Temp 2", "Get Pressure", "Write Tare Pressure", "Adjust Controls", "Reinit ADC", "Write Initial Times", "Write Pumps Present", "HMI Command", "Save Pump Times", "Check Pump Stop Time", "Save LS App Config", "Init Data File", "Reset LS Cycles", "Reset Anomalies", "Reset Opens", "Save LS Data", "Save LS Test Data", "Check Serial Numbers", "Main Tab", "Allow Data Note"]
              n241 = Unbundle By Name(w636) -> ("LS App Config.2nd Step Check"=w633:bool)
              n242 = Not Equal?(x=w633, y="Second Step Check") -> (x != y?=w635:bool)
              n243 = Bundle By Name(cluster=w638, "LS App Config.2nd Step Check"="Second Step Check") -> (w637:T26)
            }
          }
        }
        n244 = Tick Count (ms)() -> (millisecond timer value=w83:u32)
        n245 = Subtract(x=w83, y=w85) -> (x-y=w82:u32)
        n246 = Subtract(x=w83, y=w84) -> (x-y=w81:u32)
        n247 = Greater?(x=w82, y=u32 100) -> (0:w77:bool)
        n248 = Greater?(x=w81, y=u32 500) -> (0:w76:bool)
        n249 = disable-structure shown="Disabled" {
          frame Disabled {
          }
          frame Enabled {
          }
        }
        n250 = case shown="True" w76 {
          tunnel: w86 -> [w99 w103]
          tunnel: Sequence_States."Update Screen" -> [_ w102]
          tunnel: [w99 w100] -> w87
          frame False {
          }
          frame True {
            n251 = Insert Into Array(array=w103, index=0, new element=w102) -> (w100:T15[])
          }
        }
        n252 = case shown="True" w77 {
          tunnel: w87 -> [w104 w108]
          tunnel: Sequence_States."Read Inputs" -> [_ w107]
          tunnel: [w104 w105] -> w90
          frame False {
          }
          frame True {
            n253 = Insert Into Array(array=w108, index=0, new element=w107) -> (w105:T15[])
          }
        }
        n254 = case shown="True" w78 {
          tunnel: w90 -> [w109 w113]
          tunnel: Sequence_States."Check Step Time" -> [_ w112]
          tunnel: [w109 w110] -> w91
          frame False {
          }
          frame True {
            n255 = Insert Into Array(array=w113, index=0, new element=w112) -> (w110:T15[])
          }
        }
        n256 = case shown="True" w93 {
          tunnel: w91 -> [w114 w118]
          tunnel: w94 -> [_ w117]
          tunnel: [w114 w115] -> w92
          frame False {
          }
          frame True {
            n257 = Insert Into Array(array=w118, index=0, new element=w117) -> (w115:T15[])
          }
        }
      }
      frame "Init Files" {
        w672 = T15[] [enum."Write Tare Pressure", enum."Write Initial Times", enum."Write Pumps Present"] items=["Main", "Init Files", "Init", "Unused", "Save As", "Start Profile", "Check Step Time", "Alarm", "Alarm Dismiss", "Run Step", "Stop Profile", "Cycle Reset", "Time Reset", "Time Reset All", "Time Set", "Tare CTs", "Save Profile", "Open Profile", "Get Profiles", "Update Screen", "Update Controls", "Save App Config", "Write Outputs", "Disable Background", "Enable Background", "Get/Release Control", "Log Fuel Change", "Fuel Change Popup", "Read Inputs", "Remote Timer Reset", "Controller Change", "Get Alarms", "Init Alarms", "Save Alarms", "Voltage Selection", "Set Watlow Temp 1", "Set Watlow Temp 2", "Get Pressure", "Write Tare Pressure", "Adjust Controls", "Reinit ADC", "Write Initial Times", "Write Pumps Present", "HMI Command", "Save Pump Times", "Check Pump Stop Time", "Save LS App Config", "Init Data File", "Reset LS Cycles", "Reset Anomalies", "Reset Opens", "Save LS Data", "Save LS Test Data", "Check Serial Numbers", "Main Tab", "Allow Data Note"]
        w681 = dbl[][] [[0.0, 11.0, 0.0, 0.0, 0.0], [0.0, 11.0, 0.0, 0.0, 0.0], [0.0, 11.0, 0.0, 0.0, 0.0], [0.0, 11.0, 0.0, 0.0, 0.0], [0.0, 11.0, 0.0, 0.0, 0.0], [0.0, 11.0, 0.0, 0.0, 0.0], [0.0, 1.0, 0.0, 0.0, 0.0], [0.0, 1.0, 0.0, 0.0, 0.0], [0.0, 1.0, 0.0, 0.0, 0.0], [0.0, 2.0, 0.0, 0.0, 0.0], [0.0, 1.0, 0.0, 0.0, 0.0], [0.0, 1.0, 0.0, 0.0, 0.0], [0.0, 1.0, 0.0, 0.0, 0.0], [0.0, 1.0, 0.0, 0.0, 0.0], [0.0, 1.0, 0.0, 0.0, 0.0], [0.0, 1.0, 0.0, 0.0, 0.0], [0.0, 1.0, 0.0, 0.0, 0.0], [0.0, 1.0, 0.0, 0.0, 0.0], [0.0, 1.0, 0.0, 0.0, 0.0], [0.0, 1.0, 0.0, 0.0, 0.0], [0.0, 1.0, 0.0, 0.0, 0.0], [0.0, 1.0, 0.0, 0.0, 0.0], [-60.0, 24.0, 0.0, 0.0, 0.0], [-60.0, 24.0, 0.0, 0.0, 0.0], [-60.0, 24.0, 0.0, 0.0, 0.0], [-60.0, 24.0, 0.0, 0.0, 0.0], [-60.0, 24.0, 0.0, 0.0, 0.0], [-60.0, 24.0, 0.0, 0.0, 0.0], [-660.0, 200.0, 0.0, 0.0, 0.0], [-660.0, 200.0, 0.0, 0.0, 0.0], [-258.5, 258.5, 0.0, 0.0, 0.0], [-258.5, 258.5, 0.0, 0.0, 0.0], [-258.5, 258.5, 0.0, 0.0, 0.0], [-258.5, 258.5, 0.0, 0.0, 0.0], [-258.5, 258.5, 0.0, 0.0, 0.0], [-258.5, 258.5, 0.0, 0.0, 0.0], [-150.0, 150.0, 0.0, 0.0, 0.0], [-150.0, 150.0, 0.0, 0.0, 0.0], [-150.0, 150.0, 0.0, 0.0, 0.0], [-150.0, 150.0, 0.0, 0.0, 0.0], [-150.0, 150.0, 0.0, 0.0, 0.0], [-150.0, 150.0, 0.0, 0.0, 0.0], [0.0, 1.0, 0.0, 0.0, 0.0], [0.0, 1.0, 0.0, 0.0, 0.0], [0.0, 1.0, 0.0, 0.0, 0.0], [0.0, 1.0, 0.0, 0.0, 0.0], [0.0, 1.0, 0.0, 0.0, 0.0], [0.0, 1.0, 0.0, 0.0, 0.0], [0.0, 11.0, 0.0, 0.0, 0.0], [0.0, 11.0, 0.0, 0.0, 0.0], [0.0, 11.0, 0.0, 0.0, 0.0], [0.0, 11.0, 0.0, 0.0, 0.0], [0.0, 11.0, 0.0, 0.0, 0.0], [0.0, 11.0, 0.0, 0.0, 0.0], [0.0, 0.0001, 0.0, 0.0, 0.0], [0.0, 0.0001, 0.0, 0.0, 0.0], [0.0, 0.0001, 0.0, 0.0, 0.0], [0.0, 0.0001, 0.0, 0.0, 0.0], [0.0, 0.0001, 0.0, 0.0, 0.0], [0.0, 0.0001, 0.0, 0.0, 0.0]]  # Cal Coefficients
        # "This is 10.30.189.0"
        n258 = Unbundle By Name(w690) -> ("App Config"=w675:T6, "LS App Config"=w651:T13)
        n259 = String To IP() -> (0:w685:u32)  [unwired: 1 in]
        n260 = Subtract(x=w685, y=u32 169786624) -> (x-y=w657:u32)
        n261 = Number To Decimal String(number=w657) -> (decimal integer string=w684:string)  [unwired: 1 in]
        n262 = call <vilib>:"Open Config Data.vi"("configuration file path"=path "c:/LS App Config.ini") -> ("error out"=w654:errorcluster, "file created?"=w652:bool, "refnum"=w653:T47)  [unwired: 8 in]
        n263 = case shown="True" w652 {
          tunnel: w654 -> [w708 w715]
          tunnel: w653 -> [w707 w716]
          tunnel: w651 -> [w706 w714]
          tunnel: [w706 w713] -> w640
          tunnel: [w702 w709] -> w650
          frame True {
            n264 = call "Read Write LS App Config.vi"("Write (F)"=TRUE, "Error IN"=w708, "LS App Config In"=w706, "Refnum in"=w707) -> ("Error OUT"=w703:errorcluster, "Refnum out"=w704:T47)  [unwired: 5 in, 1 out]
            n265 = call <vilib>:"Close Config Data.vi"("error in (no error)"=w703, "refnum"=w704) -> ("error out"=w702:errorcluster)  [unwired: 8 in, 1 out]
          }
          frame False {
            n266 = call "Read Write LS App Config.vi"("Error IN"=w715, "LS App Config In"=w714, "Refnum in"=w716) -> ("Error OUT"=w712:errorcluster, "LS App Config Out"=w713:T13, "Refnum out"=w711:T47)  [unwired: 6 in]
            n267 = call <vilib>:"Close Config Data.vi"("error in (no error)"=w712, "refnum"=w711) -> ("error out"=w710:errorcluster)  [unwired: 8 in, 1 out]
            n268 = call <vilib>:"Clear Errors.vi"("error in (no error)"=w710) -> ("error out"=w709:errorcluster)  [unwired: 6 in]
          }
        }
        n269 = call <vilib>:"Open Config Data.vi"("error in (no error)"=w650, "configuration file path"=path "c:/App Config.ini") -> ("error out"=w697:errorcluster, "file created?"=w695:bool, "refnum"=w698:T47)  [unwired: 7 in]
        n270 = case shown="False" w695 {
          tunnel: w698 -> [w747 w752]
          tunnel: w697 -> [w745 w750]
          tunnel: w675 -> [w742 w749]
          tunnel: [w743 w749] -> w658
          tunnel: [w741 w751] -> w659
          frame False {
            # "Read App Config.ini"
            n271 = call "Read Write App Config.vi"("Error IN"=w745, "App Config"=w742, "Refnum in"=w747) -> ("Error OUT"=w744:errorcluster, "App Config OUT"=w743:T6, "Refnum out"=w746:T47)  [unwired: 6 in]
            n272 = call <vilib>:"Close Config Data.vi"("error in (no error)"=w744, "refnum"=w746) -> ("error out"=w748:errorcluster)  [unwired: 8 in, 1 out]
            n273 = call <vilib>:"Clear Errors.vi"("error in (no error)"=w748) -> ("error out"=w741:errorcluster)  [unwired: 6 in]
          }
          frame True {
            # "Doesn't exist, so create."
            n274 = call "Read Write App Config.vi"("Write (F)"=TRUE, "Error IN"=w750, "App Config"=w749, "Refnum in"=w752) -> ("Error OUT"=w754:errorcluster, "Refnum out"=w755:T47)  [unwired: 5 in, 1 out]
            n275 = call <vilib>:"Close Config Data.vi"("error in (no error)"=w754, "refnum"=w755) -> ("error out"=w751:errorcluster)  [unwired: 8 in, 1 out]
          }
        }
        n276 = Concatenate Strings("/c/" ("string"), w684, ".cal" ("string")) -> (w676:string)
        n277 = String To Path(string=w676) -> (path=w677:path)
        n278 = To Long Integer(number=w657) -> (32bit integer=w656:i32)
        n279 = Bundle By Name(cluster=w658, "Data Log Init.IP Last 3"=w656) -> (w644:T6)
        n280 = disable-structure shown="Disabled" {
          disable-tunnel: w644 -> [w699 _]
          frame Disabled {
            n281 = Unbundle By Name(w699) -> ("Data Log Init"=w700:T7)
            n282 = call "Data Logger Main.vi"("Data Logger Mode"=Data_Logger_Mode."Init", "Data Log Init"=w700) -> ()  [unwired: 18 in]
          }
          frame Enabled {
          }
        }
        n283 = Unbundle By Name(w640) -> ("2nd Step Check"=w639:bool)
        n284 = call "Get Elapsed Times.vi"("Error In"=w659, "Path"=path "c:/ElapsedTimes" ("file (use dialog)")) -> ("Error Out"=w679:errorcluster, "Elapsed Times"=w691:dbl[])  [unwired: 8 in]
        n285 = Unbundle By Name(w644) -> ("Voltage Limits"=w662:T42, "Voltage Far PI"=w669:T43, "Voltage Mid PI"=w668:T44, "Voltage Close PI"=w667:T45, "Voltage Scale"=w666:cluster{"V_FFm":dbl, "V_FFb":dbl}, "Voltage Cutoffs"=w665:cluster{"V_MidCutoff":dbl, "V_CloseCutoff":dbl}, "Pressure Scale"=w664:cluster{"Pres_FFm":dbl, "Pres_FFb":dbl}, "Temp Format"=w661:i32, "Temp Tolerance"=w660:dbl)
        n286 = call <vilib>:"Clear Errors.vi"("error in (no error)"=w679) -> ("error out"=w680:errorcluster)  [unwired: 6 in]
        n287 = local write "Second Step Check"(w639) -> ()
        n288 = Unbundle By Name(w644) -> ("Step Threshold:"=w642:dbl, "Anomaly Threshold:"=w641:dbl, "Normal Steps:"=w643:u32)
        n289 = call "Get Pressure Offsets.vi"("Error In"=w680, "Path"=path "c:/PressureOffsets" ("file (use dialog)")) -> ("Error Out"=w678:errorcluster, "Pressure Offsets"=w692:dbl[])  [unwired: 8 in]
        n290 = call <vilib>:"Clear Errors.vi"("error in (no error)"=w678) -> ("error out"=w648:errorcluster)  [unwired: 6 in]
        n291 = local write "Voltage Limits"(w662) -> ()
        n292 = local write "Far PI"(w669) -> ()
        n293 = local write "Mid PI"(w668) -> ()
        n294 = local write "Close PI"(w667) -> ()
        n295 = local write "Voltage Scale"(w666) -> ()
        n296 = local write "Cutoffs"(w665) -> ()
        n297 = local write "Pressure Scale"(w664) -> ()
        n298 = local write "Thermocouple"(w661) -> ()
        n299 = local write "Temp Tolerance"(w660) -> ()
        n300 = call "Get Initial LS Data.vi"("Error In"=w648, "Path"=path "c:/Monitored Statistics") -> ("Error Out"=w647:errorcluster, "Initial LS Data"=w645:T16)  [unwired: 8 in]
        n301 = local write "Step Threshold:"(w642) -> ()
        n302 = local write "Anomaly Threshold:"(w641) -> ()
        n303 = local write "Normal Steps:"(w643) -> ()
        n304 = call <vilib>:"Clear Errors.vi"("error in (no error)"=w647) -> ("error out"=w646:errorcluster)  [unwired: 6 in]
        n305 = call "Get Cal Coefficients.vi"("Error In"=w646, "Path"=w677) -> ("Error"=w687:bool, "Cal Coefficients"=w688:dbl[][])  [unwired: 7 in, 1 out]
        n306 = case shown="False" w687 {
          tunnel: w688 -> [_ w720]
          tunnel: [w717 w719] -> w663
          tunnel: w681 -> [w717 w718]
          frame True {
          }
          frame False {
            n307 = for {
              tunnel: w720 -> [w722] mode=indexing
              shift-right: [w723] -> w719
              shift-left: w718 -> [w724]
              i -> [w721]
              n308 = Index Array(array=w722) -> (element #1=w735:dbl, element #2=w734:dbl, element #3=w733:dbl, element #4=w729:dbl, element #5=w728:dbl)  [unwired: 5 in]
              n309 = Equal To 0?(x=w735) -> (x = 0?=w732:bool)
              n310 = Equal To 0?(x=w734) -> (x = 0?=w731:bool)
              n311 = Equal To 0?(x=w733) -> (x = 0?=w730:bool)
              n312 = Equal To 0?(x=w729) -> (x = 0?=w727:bool)
              n313 = Equal To 0?(x=w728) -> (x = 0?=w726:bool)
              n314 = Compound Arithmetic op=AND(w732, w731, w730, w727, w726) -> (w725:bool)
              n315 = case shown="False" w725 {
                tunnel: w724 -> [w739 w740]
                tunnel: [w738 w740] -> w723
                tunnel: w722 -> [w737 _]
                tunnel: w721 -> [w736 _]
                frame False {
                  n316 = Replace Array Subset(array=w739, new element=w737, index (row)=w736) -> (w738:dbl[][])  [unwired: 1 in]
                }
                frame True {
                }
              }
            }
          }
        }
        n317 = call "PI with FF.vi"("Cutoffs"=w665, "FFcluster"=w666, "ClosePIcluster"=w667, "MidPIcluster"=w668, "FarPIcluster"=w669, "LimitCluster"=w662, "Init (F)"=TRUE) -> ()  [unwired: 8 in, 1 out]
        n318 = Insert Into Array(array=w671, index=0, new element=w672) -> (w673:T15[])
        n319 = Bundle By Name(cluster=w690, "App Config"=w644, "Initial Times"=w691, "Pressure Offsets"=w692, "CalArray"=w663, "Initial LS Data"=w645, "LS App Config"=w640) -> (w689:T26)
      }
      frame "Init" {
        w774 = TRUE ("Visible")
        w773 = T31."Enabled" ("Disabled")
        w776 = FALSE
        w783 = u16 0 items=["0 - Off", "1 - On", "2 - Pulsing"] ("Bank 1 Power State:")
        w762 = FALSE ("Running?")
        w806 = T15[] [enum."Get Profiles", enum."Enable Background", enum."Get/Release Control", enum."Get Pressure", enum."Get Alarms", enum."Set Watlow Temp 1", enum."Set Watlow Temp 2", enum."Update Controls", enum."Controller Change", enum."Stop Profile"] items=["Main", "Init Files", "Init", "Unused", "Save As", "Start Profile", "Check Step Time", "Alarm", "Alarm Dismiss", "Run Step", "Stop Profile", "Cycle Reset", "Time Reset", "Time Reset All", "Time Set", "Tare CTs", "Save Profile", "Open Profile", "Get Profiles", "Update Screen", "Update Controls", "Save App Config", "Write Outputs", "Disable Background", "Enable Background", "Get/Release Control", "Log Fuel Change", "Fuel Change Popup", "Read Inputs", "Remote Timer Reset", "Controller Change", "Get Alarms", "Init Alarms", "Save Alarms", "Voltage Selection", "Set Watlow Temp 1", "Set Watlow Temp 2", "Get Pressure", "Write Tare Pressure", "Adjust Controls", "Reinit ADC", "Write Initial Times", "Write Pumps Present", "HMI Command", "Save Pump Times", "Check Pump Stop Time", "Save LS App Config", "Init Data File", "Reset LS Cycles", "Reset Anomalies", "Reset Opens", "Save LS Data", "Save LS Test Data", "Check Serial Numbers", "Main Tab", "Allow Data Note"]
        # "This solves an issue where location wouldn't\nshow up in the built version."
        n320 = Unbundle By Name(w820) -> ("App Config.Profiles Path"=w812:path, "App Config.Watlow Present"=w814:bool, "App Config.Temp 1"=w819:dbl, "App Config.Temp 2"=w818:dbl, "App Config.Location"=w813:string, "LS App Config.Record Bursts"=w779:bool, "LS App Config.RecInterval(s)"=w802:i32, "LS App Config.RecDuration(s)"=w801:i32, "LS App Config.RecFrequeny (Hz)"=w800:i32, "App Config.CA Number"=w781:string, "LS App Config.Data File Name:"=w780:string, "LS App Config.Serial Numbers"=w760:string[], "LS App Config.DetectionMode"=w763:i32)
        "Location:" <- w813
        n321 = case shown="1" w763 {
          frame 0, Default {
            n322 = local write "Live Data Tab"(enum32{"Page 1", "Page 2", "Page 3"}."Page 2" ("Live Data Tab")) -> ()
          }
          frame 1 {
            n323 = local write "Live Data Tab"(enum32{"Page 1", "Page 2", "Page 3"}."Page 3" ("Live Data Tab")) -> ()
          }
        }
        n324 = call "Init OneHour FPGA.vi"("FPGA OneHour"=w758) -> ("error out"=w757:errorcluster, "FPGA OneHour Out"=w756:T27)  [unwired: 9 in]
        n325 = call "Watlow Global.vi"("Write (F)"=TRUE, "Watlow Present"=w814) -> ()  [unwired: 9 in, 1 out]
        n326 = disable-structure shown="Disabled" {
          disable-tunnel: w756 -> [w854 _]
          disable-tunnel: w757 -> [w853 w855]
          disable-tunnel: [w852 w855] -> w817
          frame Disabled {
            n327 = call "Init ADCs.vi"("Error IN"=w853, "FPGA Ref"=w854) -> ("error out"=w852:errorcluster)  [unwired: 7 in, 2 out]
          }
          frame Enabled {
          }
        }
        n328 = local write "Main Tab"(T9."Main" ("Main Tab")) -> ()
        n329 = local write "pb.Run Profile"(FALSE ("pb.Run Profile")) -> ()
        n330 = local write "Bank 1 Power State:"(w783) -> ()
        n331 = local write "Bank 2 Power State:"(w783) -> ()
        n332 = property on="Location:" class="Str"("Text.Text"=w813) -> ()  [unwired: 2 in, 2 out]
        n333 = local write "Tank 1 Temp Cmd:"(w819) -> ()
        n334 = local write "Tank 2 Temp Cmd:"(w818) -> ()
        n335 = flat-sequence {
          tunnel: w817 -> [_]
          tunnel: w816 -> [w856]
          frame #0 {
            n336 = Set Occurrence(w856) -> ()
          }
        }
        n337 = Empty String/Path?(string/path=w781) -> (empty?=w767:bool)
        n338 = Empty String/Path?(string/path=w780) -> (empty?=w782:bool)
        n339 = Get Date/Time In Seconds() -> (seconds since 1Jan1904=w765:timestamp)
        n340 = call <vilib>:"Check if File or Folder Exists.vi"("path"=path "u:/CA Numbers" ("base path")) -> ("error out"=w797:errorcluster, "file or folder exists?"=w799:bool, "dup path"=w798:path)  [unwired: 8 in]
        n341 = Or(x=w767, y=w782) -> (x .or. y?=w772:bool)
        n342 = case shown="False" w799 {
          tunnel: w798 -> [w849 w851]
          tunnel: w797 -> [w848 w850]
          tunnel: [w847 w851] -> w795
          tunnel: [w846 w850] -> w790
          frame False {
            n343 = Create Folder(path (use dialog)=w849, error in=w848) -> (created path=w847:path, error out=w846:errorcluster)  [unwired: 1 in, 1 out]
          }
          frame True {
          }
        }
        n344 = call <vilib>:"Check if File or Folder Exists.vi"("path"=w812) -> ("file or folder exists?"=w824:bool, "dup path"=w823:path)  [unwired: 8 in, 1 out]
        n345 = property on="Time:" class="DigNum (strict)"("Visible"=w776) -> ()  [unwired: 2 in, 2 out]
        n346 = property on="Step:" class="DigNum (strict)"("Visible"=w776) -> ()  [unwired: 2 in, 2 out]
        n347 = Format Date/Time String(time format string (%c)="_%m%d%y.csv", seconds (now)=w765) -> (date/time string=w764:string)  [unwired: 1 in]
        n348 = Build Path(base path=w795, name or relative path=w781) -> (appended path=w792:path)
        n349 = case shown="False" w824 {
          tunnel: w823 -> [w857 _]
          frame False {
            n350 = Create Folder(path (use dialog)=w857) -> ()  [unwired: 2 in, 3 out]
          }
          frame True {
          }
        }
        n351 = call <vilib>:"Check if File or Folder Exists.vi"("error in (no error)"=w790, "path"=w792) -> ("error out"=w794:errorcluster, "file or folder exists?"=w768:bool, "dup path"=w793:path)  [unwired: 7 in]
        n352 = Or(x=w768, y=w767) -> (x .or. y?=w769:bool)
        n353 = case shown="False" w772 {
          tunnel: w779 -> [w828 _]
          tunnel: [w828 FALSE ("Record")] -> w775
          tunnel: [T31."Enabled" ("Disabled") T31."Disabled and Grayed Out" ("Disabled")] -> w778
          frame False {
            # "Valid File"
          }
          frame True {
            # "Invalid File"
          }
        }
        n354 = case shown="False" w769 {
          tunnel: w793 -> [w843 w845]
          tunnel: w794 -> [w842 w844]
          tunnel: [w841 w845] -> w791
          tunnel: [w840 w844] -> w785
          frame False {
            n355 = Create Folder(path (use dialog)=w843, error in=w842) -> (created path=w841:path, error out=w840:errorcluster)  [unwired: 1 in, 1 out]
          }
          frame True {
          }
        }
        n356 = Concatenate Strings(w780, w764) -> (w787:string)
        n357 = Build Path(base path=w791, name or relative path=w787) -> (appended path=w786:path)
        n358 = property on="Data File Name:" class="Str"("Visible"=w774, "DisabledEnum"=w773) -> ()  [unwired: 2 in, 2 out]
        n359 = call <vilib>:"Check if File or Folder Exists.vi"("error in (no error)"=w785, "path"=w786) -> ("error out"=w788:errorcluster, "file or folder exists?"=w771:bool, "dup path"=w789:path)  [unwired: 7 in]
        n360 = Or(x=w771, y=w772) -> (x .or. y?=w770:bool)
        n361 = case shown="False" w770 {
          tunnel: w789 -> [w837 w839]
          tunnel: w788 -> [w836 w838]
          tunnel: [w833 w839] -> w777
          tunnel: [w831 w838] -> w784
          frame False {
            n362 = Open/Create/Replace File(file path (use dialog)=w837, error in=w836, operation (0:open)=T32."create") -> (refnum out=w834:refnum<file>, error out=w832:errorcluster)  [unwired: 3 in, 1 out]
            n363 = Close File(refnum=w834, error in=w832) -> (path=w833:path, error out=w831:errorcluster)
          }
          frame True {
          }
        }
        n364 = property on="Record During Profile" class="Bool (strict)"("Value"=w775, "DisabledEnum"=w778) -> ()  [unwired: 2 in, 2 out]
        n365 = property on="pb.Run Profile" class="Bool (strict)"("Visible"=w774, "DisabledEnum"=w773) -> ()  [unwired: 2 in, 2 out]
        n366 = Bundle(cluster=T30 {"Running?"=FALSE, "Profile Record"=FALSE, "RecordInterval"=0, "RecordDuration"=0, "RecordFreq"=0, "Data Filepath"=path "", "Hr Record"=FALSE, "Serial Numbers"=[]} ("LS Cluster In"), "Running?"=w762, "Profile Record"=w775, "RecordInterval"=w802, "RecordDuration"=w801, "RecordFreq"=w800, "Data Filepath"=w777, "Hr Record"=w762, "Serial Numbers"=w760) -> (w803:T30)
        n367 = call "Controller List.vi"() -> ("Controller List OUT"=w811:T23[])  [unwired: 11 in]
        n368 = call "LS Data Global.vi"("Mode"=enum16{"Read", "Engine Writes", "Main Writes"}."Main Writes", "LS Cluster In"=w803) -> ()  [unwired: 12 in, 2 out]
        n369 = Bundle By Name(cluster=w820, "Alarm Config Path"=path "c:/Alarm Config", "Fuel Log Path"=path "u:/Fuel Change Log.csv", "Tank CMDs.Temp 1 CMD"=w819, "Tank CMDs.Temp 2 CMD"=w818, "Controller List"=w811, "LS Data Filepath"=w777, "pb.Run Profile"=w762, "LS App Config.Record Bursts"=w775) -> (w821:T26)
        n370 = call <vilib>:"Clear Errors.vi"("error in (no error)"=w784) -> ()  [unwired: 6 in, 1 out]
        n371 = Insert Into Array(array=w807, index=0, new element=w806) -> (w804:T15[])
      }
      frame "Unused" {
      }
      frame "Get Alarms" {
        n372 = Unbundle By Name(w867) -> ("Alarm Config"=w868:T10, "Alarm Config Path"=w865:path)
        n373 = call <vilib>:"Check if File or Folder Exists.vi"("path"=w865) -> ("file or folder exists?"=w870:bool, "dup path"=w869:path)  [unwired: 8 in, 1 out]
        n374 = case shown="False" w870 {
          tunnel: w869 -> [w875 w882]
          tunnel: w868 -> [_ w880]
          tunnel: [T10 {"Alarms:"=[{"Description:"="PS/E-Stop/Float Switch", "Enabled:"=TRUE, "Data Index:"=9, "Data Type:"="Tank", "Low Limit:"=5.0, "High Limit:"=20.0, "Trip Time:"=1000, "Profile Sync:"=FALSE}, {"Description:"="Voltage (pump or ctrl)", "Enabled:"=TRUE, "Data Index:"=0, "Data Type:"="Pump", "Low Limit:"=12.0, "High Limit:"=17.0, "Trip Time:"=3000, "Profile Sync:"=TRUE}, {"Description:"="Pump Current", "Enabled:"=TRUE, "Data Index:"=10, "Data Type:"="Pump", "Low Limit:"=0.0, "High Limit:"=22.0, "Trip Time:"=1000, "Profile Sync:"=TRUE}, {"Description:"="Pump Speed", "Enabled:"=TRUE, "Data Index:"=16, "Data Type:"="Pump", "Low Limit:"=0.0, "High Limit:"=10000.0, "Trip Time:"=1000, "Profile Sync:"=TRUE}, {"Description:"="Controller Current", "Enabled:"=TRUE, "Data Index:"=22, "Data Type:"="Pump", "Low Limit:"=0.0, "High Limit:"=20.0, "Trip Time:"=1000, "Profile Sync:"=TRUE}, {"Description:"="Pump Pressure", "Enabled:"=TRUE, "Data Index:"=30, "Data Type:"="Pump", "Low Limit:"=550.0, "High Limit:"=750.0, "Trip Time:"=1000, "Profile Sync:"=TRUE}, {"Description:"="Pump Flow", "Enabled:"=FALSE, "Data Index:"=36, "Data Type:"="Pump", "Low Limit:"=0.0, "High Limit:"=400.0, "Trip Time:"=1000, "Profile Sync:"=TRUE}, {"Description:"="Tank Temperature 1", "Enabled:"=FALSE, "Data Index:"=28, "Data Type:"="Tank", "Low Limit:"=-50.0, "High Limit:"=0.0, "Trip Time:"=10000, "Profile Sync:"=FALSE}, {"Description:"="Tank Temperature 2", "Enabled:"=FALSE, "Data Index:"=29, "Data Type:"="Tank", "Low Limit:"=0.0, "High Limit:"=70.0, "Trip Time:"=10000, "Profile Sync:"=FALSE}], "Profile Sync:"={"Trip Time:"=2000, "Consecutive Trips:"=5}} ("Alarm Config") w878] -> w861
          tunnel: [w872 w877] -> w860
          frame False {
            w872 = T15[] [enum."Init Alarms", enum."Save Alarms"] items=["Main", "Init Files", "Init", "Unused", "Save As", "Start Profile", "Check Step Time", "Alarm", "Alarm Dismiss", "Run Step", "Stop Profile", "Cycle Reset", "Time Reset", "Time Reset All", "Time Set", "Tare CTs", "Save Profile", "Open Profile", "Get Profiles", "Update Screen", "Update Controls", "Save App Config", "Write Outputs", "Disable Background", "Enable Background", "Get/Release Control", "Log Fuel Change", "Fuel Change Popup", "Read Inputs", "Remote Timer Reset", "Controller Change", "Get Alarms", "Init Alarms", "Save Alarms", "Voltage Selection", "Set Watlow Temp 1", "Set Watlow Temp 2", "Get Pressure", "Write Tare Pressure", "Adjust Controls", "Reinit ADC", "Write Initial Times", "Write Pumps Present", "HMI Command", "Save Pump Times", "Check Pump Stop Time", "Save LS App Config", "Init Data File", "Reset LS Cycles", "Reset Anomalies", "Reset Opens", "Save LS Data", "Save LS Test Data", "Check Serial Numbers", "Main Tab", "Allow Data Note"]
            n375 = Open/Create/Replace File(file path (use dialog)=w875, operation (0:open)=T32."create") -> (refnum out=w874:refnum<file>, error out=w873:errorcluster)  [unwired: 4 in, 1 out]
            n376 = Close File(refnum=w874, error in=w873) -> ()  [unwired: 2 out]
          }
          frame True {
            w877 = T15[] [enum."Init Alarms"] items=["Main", "Init Files", "Init", "Unused", "Save As", "Start Profile", "Check Step Time", "Alarm", "Alarm Dismiss", "Run Step", "Stop Profile", "Cycle Reset", "Time Reset", "Time Reset All", "Time Set", "Tare CTs", "Save Profile", "Open Profile", "Get Profiles", "Update Screen", "Update Controls", "Save App Config", "Write Outputs", "Disable Background", "Enable Background", "Get/Release Control", "Log Fuel Change", "Fuel Change Popup", "Read Inputs", "Remote Timer Reset", "Controller Change", "Get Alarms", "Init Alarms", "Save Alarms", "Voltage Selection", "Set Watlow Temp 1", "Set Watlow Temp 2", "Get Pressure", "Write Tare Pressure", "Adjust Controls", "Reinit ADC", "Write Initial Times", "Write Pumps Present", "HMI Command", "Save Pump Times", "Check Pump Stop Time", "Save LS App Config", "Init Data File", "Reset LS Cycles", "Reset Anomalies", "Reset Opens", "Save LS Data", "Save LS Test Data", "Check Serial Numbers", "Main Tab", "Allow Data Note"]
            n377 = Read from Text File(file (use dialog)=w882) -> (refnum out=w879:refnum<file>, text=w881:string)  [unwired: 3 in, 2 out]
            n378 = Close File(refnum=w879) -> ()  [unwired: 1 in, 2 out]
            n379 = Unflatten From JSON(JSON string=w881, type and defaults=w880) -> (value=w878:T10)  [unwired: 5 in, 1 out]
          }
        }
        n380 = Bundle By Name(cluster=w867, "Alarm Config"=w861) -> (w866:T26)
        n381 = local write "Alarm Config"(w861) -> ()
        n382 = Insert Into Array(array=w862, index=0, new element=w860) -> (w863:T15[])
      }
      frame "Init Alarms" {
        # "Initialize alarm arrays."
        n383 = Unbundle By Name(w889) -> ("Alarm Config.Alarms:"=w891:T11[])
        n384 = for {
          tunnel: w891 -> [w898] mode=indexing
          shift-right: [w894] -> w885
          shift-left: 0 -> [w893]
          n385 = Unbundle By Name(w898) -> ("Data Type:"=w897:string, "Enabled:"=w896:bool)
          n386 = case shown="\"Pump\", Default" w897 {
            tunnel: [6 1] -> w895
            frame "Pump", Default {
            }
            frame "Tank" {
            }
          }
          n387 = case shown="True" w896 {
            tunnel: w895 -> [_ w902]
            tunnel: [w899 w901] -> w894
            tunnel: w893 -> [w899 w900]
            frame False {
            }
            frame True {
              n388 = Add(x=w902, y=w900) -> (x+y=w901:i32)
            }
          }
        }
        n389 = Tick Count (ms)() -> (millisecond timer value=w886:u32)
        n390 = Initialize Array(0, w885) -> (w884:i32[])
        n391 = Initialize Array(w886, w885) -> (w883:u32[])
        n392 = Bundle By Name(cluster=w889, "Trip Counters"=w884, "Previous Times"=w883, "Prev ON Times"=w883) -> (w888:T26)
      }
      frame "Save Alarms" {
        n393 = Unbundle By Name(w908) -> ("Alarm Config Path"=w906:path, "Alarm Config"=w907:T10)
        n394 = Flatten To JSON(anything=w907) -> (JSON string=w905:string)  [unwired: 2 in, 1 out]
        n395 = Write to Text File(file (use dialog)=w906, text=w905) -> ()  [unwired: 2 in, 3 out]
      }
      frame "Get Profiles" {
        n396 = Unbundle By Name(w917) -> ("App Config.Profiles Path"=w918:path)
        n397 = List Folder(path=w918) -> (filenames=w915:string[], error out=w914:errorcluster)  [unwired: 3 in, 2 out]
        n398 = call <vilib>:"Clear Errors.vi"("error in (no error)"=w914) -> ()  [unwired: 6 in, 1 out]
        n399 = property on="Profile Name:" class="CmbBox"("Strings[]"=w915) -> ()  [unwired: 2 in, 2 out]
        n400 = Bundle By Name(cluster=w917, "Profiles"=w915) -> (w916:T26)
        n401 = Insert Into Array(array=w911, index=0, new element=Sequence_States."Open Profile") -> (w910:T15[])
      }
      frame "Open Profile" {
        w920 = T15[] [enum."Update Screen", enum."Save App Config"] items=["Main", "Init Files", "Init", "Unused", "Save As", "Start Profile", "Check Step Time", "Alarm", "Alarm Dismiss", "Run Step", "Stop Profile", "Cycle Reset", "Time Reset", "Time Reset All", "Time Set", "Tare CTs", "Save Profile", "Open Profile", "Get Profiles", "Update Screen", "Update Controls", "Save App Config", "Write Outputs", "Disable Background", "Enable Background", "Get/Release Control", "Log Fuel Change", "Fuel Change Popup", "Read Inputs", "Remote Timer Reset", "Controller Change", "Get Alarms", "Init Alarms", "Save Alarms", "Voltage Selection", "Set Watlow Temp 1", "Set Watlow Temp 2", "Get Pressure", "Write Tare Pressure", "Adjust Controls", "Reinit ADC", "Write Initial Times", "Write Pumps Present", "HMI Command", "Save Pump Times", "Check Pump Stop Time", "Save LS App Config", "Init Data File", "Reset LS Cycles", "Reset Anomalies", "Reset Opens", "Save LS Data", "Save LS Test Data", "Check Serial Numbers", "Main Tab", "Allow Data Note"]
        n402 = Unbundle By Name(w932) -> ("App Config.Profiles Path"=w934:path, "App Config.Current Profile"=w933:string)
        n403 = Build Path(base path=w934, name or relative path=w933) -> (appended path=w929:path)
        n404 = Read from Text File(file (use dialog)=w929) -> (refnum out=w927:refnum<file>, text=w928:string, error out=w926:errorcluster)  [unwired: 3 in, 1 out]
        n405 = Close File(refnum=w927, error in=w926) -> (error out=w925:errorcluster)  [unwired: 1 out]
        n406 = case shown="No Error" w925 {
          tunnel: w928 -> [w936 _]
          tunnel: [w937 string[][] []] -> w919
          frame No Error {
            n407 = Spreadsheet String To Array(delimiter (Tab)=",", format string="%s", spreadsheet string=w936, array type (2D Dbl)=string[][] []) -> (array=w937:string[][])
          }
          frame Error {
          }
        }
        n408 = Array Size(array=w919) -> (size(s)=w930:i32[])
        n409 = Index Array(array=w930) -> (element=w924:i32)  [unwired: 1 in]
        n410 = Bundle By Name(cluster=w932, "Profile"=w919, "# of Steps"=w924) -> (w931:T26)
        n411 = Insert Into Array(array=w922, index=0, new element=w920) -> (w921:T15[])
      }
      frame "Save Profile" {
        n412 = Unbundle By Name(w946) -> ("App Config.Profiles Path"=w950:path, "App Config.Current Profile"=w948:string, "Profile"=w949:string[][])
        n413 = Empty String/Path?(string/path=w948) -> (empty?=w947:bool)
        n414 = case shown="False" w947 {
          tunnel: w950 -> [w954 _]
          tunnel: w948 -> [w953 _]
          tunnel: w949 -> [w952 _]
          tunnel: [w951 string[][] [] ("Profile OUT")] -> w943
          frame False {
            n415 = call "Save Profile.vi"("Profile"=w952, "Current Profile"=w953, "Profiles Path"=w954) -> ("Profile OUT"=w951:string[][])  [unwired: 8 in]
          }
          frame True {
          }
        }
        n416 = Array Size(array=w943) -> (size(s)=w944:i32[])
        n417 = Index Array(array=w944) -> (element=w942:i32)  [unwired: 1 in]
        n418 = Bundle By Name(cluster=w946, "Profile"=w943, "# of Steps"=w942) -> (w945:T26)
      }
      frame "Start Profile" {
        w957 = TRUE ("Running?")
        w969 = TRUE
        w972 = T15[] [enum."Init Alarms", enum."Check Step Time"] items=["Main", "Init Files", "Init", "Unused", "Save As", "Start Profile", "Check Step Time", "Alarm", "Alarm Dismiss", "Run Step", "Stop Profile", "Cycle Reset", "Time Reset", "Time Reset All", "Time Set", "Tare CTs", "Save Profile", "Open Profile", "Get Profiles", "Update Screen", "Update Controls", "Save App Config", "Write Outputs", "Disable Background", "Enable Background", "Get/Release Control", "Log Fuel Change", "Fuel Change Popup", "Read Inputs", "Remote Timer Reset", "Controller Change", "Get Alarms", "Init Alarms", "Save Alarms", "Voltage Selection", "Set Watlow Temp 1", "Set Watlow Temp 2", "Get Pressure", "Write Tare Pressure", "Adjust Controls", "Reinit ADC", "Write Initial Times", "Write Pumps Present", "HMI Command", "Save Pump Times", "Check Pump Stop Time", "Save LS App Config", "Init Data File", "Reset LS Cycles", "Reset Anomalies", "Reset Opens", "Save LS Data", "Save LS Test Data", "Check Serial Numbers", "Main Tab", "Allow Data Note"]
        w975 = 0 ("Current Step")
        w968 = T31."Disabled" ("Disabled")
        n419 = Unbundle By Name(w958) -> ("LS App Config.Record Bursts"=w966:bool, "LS App Config.RecInterval(s)"=w965:i32, "LS App Config.RecDuration(s)"=w964:i32, "LS App Config.RecFrequeny (Hz)"=w963:i32, "LS Data Filepath"=w962:path, "LS App Config.Record Constant"=w960:bool, "LS App Config.Serial Numbers"=w959:string[])
        n420 = Bundle(cluster=T30 {"Running?"=FALSE, "Profile Record"=FALSE, "RecordInterval"=0, "RecordDuration"=0, "RecordFreq"=0, "Data Filepath"=path "", "Hr Record"=FALSE, "Serial Numbers"=[]} ("LS Cluster In"), "Running?"=w957, "Profile Record"=w966, "RecordInterval"=w965, "RecordDuration"=w964, "RecordFreq"=w963, "Data Filepath"=w962, "Hr Record"=w960, "Serial Numbers"=w959) -> (w967:T30)
        n421 = disable-structure shown="Disabled" {
          disable-tunnel: "Data Log Enabled" -> [w982 _]
          disable-tunnel: w958 -> [w981 _]
          frame Disabled {
            n422 = case shown="True" w982 {
              tunnel: w981 -> [_ w989]
              frame False {
              }
              frame True {
                n423 = Unbundle By Name(w989) -> ("App Config"=w988:T6, "Profile"=w987:string[][], "App Config.Controller Type:"=w986:T3, "Tank CMDs"=w984:T20)
                n424 = Format Into String(w986) -> (resulting string=w985:string)  [unwired: 3 in, 1 out]
                n425 = Bundle By Name(cluster=T33 {"App Config"={"Location"="", "Profiles Path"=path "", "Current Profile"="", "CA Number"="", "Cycles Completed"=0, "Controller Type:"=enum."Kuhnke", "Stagger Time (ms)"=0, "Tank 1 Fuel"="", "Tank 2 Fuel"="", "Serial Numbers"={"Position 1 SN"="", "Position 2 SN"="", "Poaition 3 SN"="", "Position 4 SN"="", "Position 5 SN"="", "Position 6 SN"=""}, "Pumps Present"={"Pump 1"=FALSE, "Pump 2"=FALSE, "Pump 3"=FALSE, "Pump 4"=FALSE, "Pump 5"=FALSE, "Pump 6"=FALSE}, "VoltCtrlRef"="", "VoltageSelect"=FALSE, "Watlow Present"=FALSE, "Temp 1"=0.0, "Temp 2"=0.0, "V_Run PI?"=FALSE, "Voltage Limits"={"V_Step"=0.0, "V_CmdMax"=0.0, "V_CmdMin"=0.0}, "Voltage Far PI"={"V_FarSlew"=0.0, "V_FarKp"=0.0, "V_FarKi"=0.0}, "Voltage Mid PI"={"V_MidSlew"=0.0, "V_MidKp"=0.0, "V_MidKi"=0.0}, "Voltage Close PI"={"V_CloseSlew"=0.0, "V_CloseKp"=0.0, "V_CloseKi"=0.0}, "Voltage Scale"={"V_FFm"=0.0, "V_FFb"=0.0}, "Voltage Cutoffs"={"V_MidCutoff"=0.0, "V_CloseCutoff"=0.0}, "Pressure Scale"={"Pres_FFm"=0.0, "Pres_FFb"=0.0}, "Temp Format"=0, "Temp Tolerance"=0.0, "Target Voltage"=0.0, "Target Pressure"=0.0, "Data Log Init"={"Data Path"=path "", "Data Log Rate (S/s)"=0, "AKLH Rate (Hours/S)"=0.0, "Sync Time Offset (min)"=0, "IP Last 3"=0, "WebDAV IP"=""}, "Email Handler IP"="", "ADC Check"=FALSE, "3 Pump Tank"=FALSE, "Cycle Threshold:"=0.0, "Cycle Pts to Avg:"=0, "Anomaly Threshold:"=0.0, "Normal Steps:"=0, "Step Threshold:"=0.0}, "Profile"=[], "Controller Type"="", "Tank CMDs"={"PS CMD"=0.0, "Press CMD"=0.0, "Temp 1 CMD"=0.0, "Temp 2 CMD"=0.0}} ("Data Log Start"), "App Config"=w988, "Profile"=w987, "Controller Type"=w985, "Tank CMDs"=w984) -> (w990:T33)
                n426 = call "Data Logger Main.vi"("Data Logger Mode"=Data_Logger_Mode."Start", "Data Log Start"=w990) -> ()  [unwired: 18 in]
              }
            }
          }
          frame Enabled {
          }
        }
        n427 = call "LS Data Global.vi"("Mode"=enum16{"Read", "Engine Writes", "Main Writes"}."Main Writes", "LS Cluster In"=w967) -> ()  [unwired: 12 in, 2 out]
        n428 = property on="Time:" class="DigNum (strict)"("Visible"=w969) -> ()  [unwired: 2 in, 2 out]
        n429 = property on="Step:" class="DigNum (strict)"("Visible"=w969) -> ()  [unwired: 2 in, 2 out]
        n430 = property on="Bank 1" class="Clust (strict)"("DisabledEnum"=w968) -> ()  [unwired: 2 in, 2 out]
        n431 = property on="Bank 2" class="Clust (strict)"("DisabledEnum"=w968) -> ()  [unwired: 2 in, 2 out]
        n432 = property on="Live Data Tab" class="TabCtl (strict)"("DisabledEnum"=w968) -> ()  [unwired: 2 in, 2 out]
        n433 = property on="Pump Timers Tab" class="TabCtl (strict)"("DisabledEnum"=w968) -> ()  [unwired: 2 in, 2 out]
        n434 = Get Date/Time In Seconds() -> (seconds since 1Jan1904=w978:timestamp)
        n435 = To Double Precision Float(number=w978) -> (double precision float=w977:dbl)
        n436 = Bundle By Name(cluster=w958, "Recording"="Data Log Enabled", "Run Profile"=TRUE, "Step Start Time"=w977, "Last Profile Time"=w977, "Step Time"=0.0, "Current Step"=w975, "Stagger Counter"=w975, "pb.Run Profile"=w957) -> (w980:T26)
        n437 = Insert Into Array(array=w974, index=0, new element=w972) -> (w973:T15[])
      }
      frame "Check Step Time" {
        # "T: Test has to be running to be in this state\nRecording has been happening and has now stopped so stop runnning pumps"
        # "Time elapsed since\nstart of step."
        n438 = Unbundle By Name(w1019) -> ("Step Start Time"=w1022:dbl, "Step Time"=w1020:dbl, "Current Step"=w1017:i32, "App Config.Stagger Time (ms)"=w1002:i32, "Stagger Counter"=w1008:i32)
        n439 = Get Date/Time In Seconds() -> (seconds since 1Jan1904=w1021:timestamp)
        n440 = local read "Recording"() -> (w993:bool)
        n441 = Increment(x=w1008) -> (x+1=w1003:i32)
        n442 = To Double Precision Float(number=w1021) -> (double precision float=w1016:dbl)
        n443 = Multiply(x=w1002, y=w1003) -> (x*y=w1014:i32)
        n444 = Subtract(x=w1016, y=w1022) -> (x-y=w1013:dbl)
        n445 = To Double Precision Float(number=w1014) -> (double precision float=w1007:dbl)
        n446 = feedback #3(FALSE ("Record Constant")) -> (w992:bool)
        n447 = feedback-in #3(w993) -> ()
        n448 = Divide(x=w1007, y=1000.0) -> (x/y=w1005:dbl)
        n449 = Less?(x=w993, y=w992) -> (x < y?=w994:bool)
        n450 = Not Equal To 0?(x=w1002) -> (x != 0?=w1001:bool)
        n451 = Greater Or Equal?(x=w1013, y=w1005) -> (x >= y?=w1012:bool)
        n452 = Less Or Equal?(x=w1008, y=4) -> (x <= y?=w1010:bool)
        n453 = Subtract(x=w1020, y=w1013) -> (x-y=w998:dbl)
        "Time:" <- w998
        n454 = Compound Arithmetic op=AND(w1012, w1010, w1001) -> (w1009:bool)
        n455 = Less Or Equal To 0?(x=w998) -> (x <= 0?=w1004:bool)
        n456 = case shown="False" w1004 {
          tunnel: [w1029 w1037] -> w997
          tunnel: w1017 -> [w1030 w1039]
          tunnel: [w1030 w1038] -> w999
          tunnel: [w1026 0 ("Stagger Counter")] -> w1015
          tunnel: w1009 -> [w1028 _]
          tunnel: w1008 -> [w1027 _]
          tunnel: w1000 -> [w1025 _]
          frame False {
            # "There's time left.  Update screen."
            n457 = case shown="True" w1028 {
              tunnel: [w1031 w1035] -> w1029
              tunnel: w1027 -> [w1032 w1034]
              tunnel: [w1032 w1033] -> w1026
              tunnel: w1025 -> [w1031 _]
              frame False {
              }
              frame True {
                w1035 = T15[] [enum."Run Step"] items=["Main", "Init Files", "Init", "Unused", "Save As", "Start Profile", "Check Step Time", "Alarm", "Alarm Dismiss", "Run Step", "Stop Profile", "Cycle Reset", "Time Reset", "Time Reset All", "Time Set", "Tare CTs", "Save Profile", "Open Profile", "Get Profiles", "Update Screen", "Update Controls", "Save App Config", "Write Outputs", "Disable Background", "Enable Background", "Get/Release Control", "Log Fuel Change", "Fuel Change Popup", "Read Inputs", "Remote Timer Reset", "Controller Change", "Get Alarms", "Init Alarms", "Save Alarms", "Voltage Selection", "Set Watlow Temp 1", "Set Watlow Temp 2", "Get Pressure", "Write Tare Pressure", "Adjust Controls", "Reinit ADC", "Write Initial Times", "Write Pumps Present", "HMI Command", "Save Pump Times", "Check Pump Stop Time", "Save LS App Config", "Init Data File", "Reset LS Cycles", "Reset Anomalies", "Reset Opens", "Save LS Data", "Save LS Test Data", "Check Serial Numbers", "Main Tab", "Allow Data Note"]
                n458 = Increment(x=w1034) -> (x+1=w1033:i32)
              }
            }
          }
          frame True {
            w1037 = T15[] [enum."Run Step"] items=["Main", "Init Files", "Init", "Unused", "Save As", "Start Profile", "Check Step Time", "Alarm", "Alarm Dismiss", "Run Step", "Stop Profile", "Cycle Reset", "Time Reset", "Time Reset All", "Time Set", "Tare CTs", "Save Profile", "Open Profile", "Get Profiles", "Update Screen", "Update Controls", "Save App Config", "Write Outputs", "Disable Background", "Enable Background", "Get/Release Control", "Log Fuel Change", "Fuel Change Popup", "Read Inputs", "Remote Timer Reset", "Controller Change", "Get Alarms", "Init Alarms", "Save Alarms", "Voltage Selection", "Set Watlow Temp 1", "Set Watlow Temp 2", "Get Pressure", "Write Tare Pressure", "Adjust Controls", "Reinit ADC", "Write Initial Times", "Write Pumps Present", "HMI Command", "Save Pump Times", "Check Pump Stop Time", "Save LS App Config", "Init Data File", "Reset LS Cycles", "Reset Anomalies", "Reset Opens", "Save LS Data", "Save LS Test Data", "Check Serial Numbers", "Main Tab", "Allow Data Note"]
            # "No time left.  Go to next step."
            n459 = Increment(x=w1039) -> (x+1=w1038:i32)
          }
        }
        "Step:" <- w999
        n460 = case shown="True" w994 {
          tunnel: w997 -> [w1023 _]
          tunnel: [w1023 w1024] -> w996
          frame False {
          }
          frame True {
            w1024 = T15[] [enum."Stop Profile"] items=["Main", "Init Files", "Init", "Unused", "Save As", "Start Profile", "Check Step Time", "Alarm", "Alarm Dismiss", "Run Step", "Stop Profile", "Cycle Reset", "Time Reset", "Time Reset All", "Time Set", "Tare CTs", "Save Profile", "Open Profile", "Get Profiles", "Update Screen", "Update Controls", "Save App Config", "Write Outputs", "Disable Background", "Enable Background", "Get/Release Control", "Log Fuel Change", "Fuel Change Popup", "Read Inputs", "Remote Timer Reset", "Controller Change", "Get Alarms", "Init Alarms", "Save Alarms", "Voltage Selection", "Set Watlow Temp 1", "Set Watlow Temp 2", "Get Pressure", "Write Tare Pressure", "Adjust Controls", "Reinit ADC", "Write Initial Times", "Write Pumps Present", "HMI Command", "Save Pump Times", "Check Pump Stop Time", "Save LS App Config", "Init Data File", "Reset LS Cycles", "Reset Anomalies", "Reset Opens", "Save LS Data", "Save LS Test Data", "Check Serial Numbers", "Main Tab", "Allow Data Note"]
          }
        }
        n461 = Bundle By Name(cluster=w1019, "Last Profile Time"=w1016, "Step Time Left"=w998, "New Step"=w1004, "Current Step"=w999, "Stagger Counter"=w1015) -> (w1018:T26)
      }
      frame "Run Step" {
        w1049 = T15[] [enum."Write Outputs", enum."Read Inputs", enum."Update Screen"] items=["Main", "Init Files", "Init", "Unused", "Save As", "Start Profile", "Check Step Time", "Alarm", "Alarm Dismiss", "Run Step", "Stop Profile", "Cycle Reset", "Time Reset", "Time Reset All", "Time Set", "Tare CTs", "Save Profile", "Open Profile", "Get Profiles", "Update Screen", "Update Controls", "Save App Config", "Write Outputs", "Disable Background", "Enable Background", "Get/Release Control", "Log Fuel Change", "Fuel Change Popup", "Read Inputs", "Remote Timer Reset", "Controller Change", "Get Alarms", "Init Alarms", "Save Alarms", "Voltage Selection", "Set Watlow Temp 1", "Set Watlow Temp 2", "Get Pressure", "Write Tare Pressure", "Adjust Controls", "Reinit ADC", "Write Initial Times", "Write Pumps Present", "HMI Command", "Save Pump Times", "Check Pump Stop Time", "Save LS App Config", "Init Data File", "Reset LS Cycles", "Reset Anomalies", "Reset Opens", "Save LS Data", "Save LS Test Data", "Check Serial Numbers", "Main Tab", "Allow Data Note"]
        n462 = Unbundle By Name(w1067) -> ("Profile"=w1061:string[][], "Current Step"=w1060:i32, "# of Steps"=w1059:i32, "App Config.Cycles Completed"=w1058:u32, "App Config.Pumps Present"=w1050:T8, "New Step"=w1065:bool, "Step Start Time"=w1064:dbl)
        n463 = call "Run Step.vi"("Profile"=w1061, "Current Step in"=w1060, "# of Steps"=w1059, "Cycles Completed in"=w1058, "Pumps Present"=w1050) -> ("Bank1State"=w1043:u16, "Bank2State"=w1042:u16, "LS Freq"=w1041:dbl, "LS Duty"=w1040:dbl, "PS Cmd"=w1057:dbl, "Press Cmd"=w1056:dbl, "Ignition Relays"=w1055:T8, "Current Step out"=w1054:i32, "Cycles Completed out"=w1053:u32, "Step Time"=w1052:dbl, "Controller CMDs"=w1051:dbl[], "Power Relays"=w1047:T8)  [unwired: 11 in]
        n464 = local write "Bank 1 Power State:"(w1043) -> ()
        n465 = local write "Bank 2 Power State:"(w1042) -> ()
        n466 = local write "LS Power (Freq):"(w1041) -> ()
        n467 = local write "LS Power (Duty):"(w1040) -> ()
        n468 = case shown="True" w1065 {
          tunnel: [w1076 w1077] -> w1048
          tunnel: w1064 -> [w1076 _]
          tunnel: w1051 -> [_ _]
          frame False {
          }
          frame True {
            n469 = Get Date/Time In Seconds() -> (seconds since 1Jan1904=w1078:timestamp)
            n470 = To Double Precision Float(number=w1078) -> (double precision float=w1077:dbl)
          }
        }
        n471 = Insert Into Array(array=w1062, index=0, new element=w1049) -> (w1046:T15[])
        n472 = flat-sequence {
          tunnel: w1048 -> [_]
          frame #0 {
            n473 = Tick Count (ms)() -> (millisecond timer value=w1075:u32)
            n474 = feedback #4() -> (w1074:u32)  [unwired: 1 in]
            n475 = feedback-in #4(w1075) -> ()
            n476 = Subtract(x=w1075, y=w1074) -> (x-y=→"Run Step (ms)":u32)
          }
        }
        n477 = case shown="True" "Stop Time Enable" {
          tunnel: w1046 -> [w1068 w1070]
          tunnel: [w1068 w1069] -> w1045
          frame False {
          }
          frame True {
            w1072 = T15[] [enum."Check Pump Stop Time"] items=["Main", "Init Files", "Init", "Unused", "Save As", "Start Profile", "Check Step Time", "Alarm", "Alarm Dismiss", "Run Step", "Stop Profile", "Cycle Reset", "Time Reset", "Time Reset All", "Time Set", "Tare CTs", "Save Profile", "Open Profile", "Get Profiles", "Update Screen", "Update Controls", "Save App Config", "Write Outputs", "Disable Background", "Enable Background", "Get/Release Control", "Log Fuel Change", "Fuel Change Popup", "Read Inputs", "Remote Timer Reset", "Controller Change", "Get Alarms", "Init Alarms", "Save Alarms", "Voltage Selection", "Set Watlow Temp 1", "Set Watlow Temp 2", "Get Pressure", "Write Tare Pressure", "Adjust Controls", "Reinit ADC", "Write Initial Times", "Write Pumps Present", "HMI Command", "Save Pump Times", "Check Pump Stop Time", "Save LS App Config", "Init Data File", "Reset LS Cycles", "Reset Anomalies", "Reset Opens", "Save LS Data", "Save LS Test Data", "Check Serial Numbers", "Main Tab", "Allow Data Note"]
            n478 = Insert Into Array(array=w1070, index=0, new element=w1072) -> (w1069:T15[])
          }
        }
        n479 = Bundle By Name(cluster=w1067, "Bank 1 State:"=w1043, "Bank 2 State:"=w1042, "LS App Config.LS Power (Freq):"=w1041, "LS App Config.LS Power (Duty):"=w1040, "Tank CMDs.PS CMD"=w1057, "Tank CMDs.Press CMD"=w1056, "Ignition Relay"=w1055, "Current Step"=w1054, "App Config.Cycles Completed"=w1053, "Step Time"=w1052, "Controller CMDs"=w1051, "Power Relay"=w1047, "Step Start Time"=w1048) -> (w1066:T26)
      }
      frame "Write Outputs" {
        w1081 = fxp<+/-,28,17> 0.0 ("Step Threshold")
        w1114 = T15[] [] items=["Main", "Init Files", "Init", "Unused", "Save As", "Start Profile", "Check Step Time", "Alarm", "Alarm Dismiss", "Run Step", "Stop Profile", "Cycle Reset", "Time Reset", "Time Reset All", "Time Set", "Tare CTs", "Save Profile", "Open Profile", "Get Profiles", "Update Screen", "Update Controls", "Save App Config", "Write Outputs", "Disable Background", "Enable Background", "Get/Release Control", "Log Fuel Change", "Fuel Change Popup", "Read Inputs", "Remote Timer Reset", "Controller Change", "Get Alarms", "Init Alarms", "Save Alarms", "Voltage Selection", "Set Watlow Temp 1", "Set Watlow Temp 2", "Get Pressure", "Write Tare Pressure", "Adjust Controls", "Reinit ADC", "Write Initial Times", "Write Pumps Present", "HMI Command", "Save Pump Times", "Check Pump Stop Time", "Save LS App Config", "Init Data File", "Reset LS Cycles", "Reset Anomalies", "Reset Opens", "Save LS Data", "Save LS Test Data", "Check Serial Numbers", "Main Tab", "Allow Data Note"]
        # "T:Anomalies     F:Opens"
        n480 = Unbundle By Name(w1129) -> ("App Config.Pumps Present"=w1135:T8, "Controller Config.Controller Name"=w1136:T3, "Controller Config.Frequency"=w1134:i32, "Controller CMDs"=w1133:dbl[], "Stagger Counter"=w1132:i32, "App Config.Stagger Time (ms)"=w1131:i32, "Run Profile"=w1130:bool, "Power Relay"=w1120:T8, "Ignition Relay"=w1119:T8, "Tank CMDs"=w1122:T20, "App Config"=w1121:T6, "Voltage Enable"=w1118:bool, "App Config.V_Run PI?"=w1126:bool, "Tank CMDs.PS CMD"=w1124:dbl, "Tank Data.PS Actual (V):"=w1125:dbl, "App Config.VoltCtrlRef"=w1123:string, "LS App Config.Bank 1 Present"=w1113:T2, "LS App Config.Bank 2 Present"=w1112:T1, "LS App Config.DetectionMode"=w1093:i32, "Bank 1 State:"=w1100:u16, "Bank 2 State:"=w1103:u16, "LS App Config.LS Power (Freq):"=w1111:dbl, "LS App Config.LS Power (Duty):"=w1102:dbl, "App Config.Normal Steps:"=w1087:u32, "App Config.Anomaly Threshold:"=w1084:dbl, "App Config.Step Threshold:"=w1085:dbl, "LS App Config.2nd Step Check"=w1080:bool)
        n481 = Cluster To Array(cluster=w1113) -> (array=w1096:bool[])
        n482 = Cluster To Array(cluster=w1112) -> (array=w1098:bool[])
        n483 = Equal To 0?(x=w1093) -> (x = 0?=w1092:bool)
        n484 = Divide(x=40000000.0, y=w1111) -> (x/y=w1106:dbl)
        n485 = case shown="2" w1100 {
          tunnel: [FALSE FALSE TRUE] -> w1099
          tunnel: [FALSE TRUE FALSE] -> w1088
          frame 0, Default {
            # "Off"
          }
          frame 1 {
            # "On"
          }
          frame 2 {
            # "Pulsing"
          }
        }
        n486 = case shown="2" w1103 {
          tunnel: [FALSE FALSE TRUE] -> w1101
          tunnel: [FALSE TRUE FALSE] -> w1089
          frame 0, Default {
            # "Off"
          }
          frame 1 {
            # "On"
          }
          frame 2 {
            # "Pulsing"
          }
        }
        n487 = Divide(x=w1106, y=100.0) -> (x/y=w1108:dbl)
        n488 = disable-structure shown="Enabled" {
          disable-tunnel: w1136 -> [w1168 _]
          disable-tunnel: w1135 -> [w1167 _]
          disable-tunnel: w1134 -> [w1166 _]
          disable-tunnel: w1133 -> [w1165 w1197]
          disable-tunnel: w1132 -> [w1164 _]
          disable-tunnel: w1131 -> [w1163 _]
          disable-tunnel: w1130 -> [w1162 _]
          disable-tunnel: [w1161 w1197] -> w1127
          disable-tunnel: w1126 -> [w1160 _]
          disable-tunnel: w1125 -> [w1159 _]
          disable-tunnel: w1086 -> [w1157 _]
          disable-tunnel: w1124 -> [w1155 _]
          disable-tunnel: w1123 -> [w1154 _]
          disable-tunnel: w1122 -> [w1153 _]
          disable-tunnel: w1121 -> [w1152 _]
          disable-tunnel: w1120 -> [w1151 _]
          disable-tunnel: w1119 -> [w1150 _]
          disable-tunnel: w1118 -> [w1149 _]
          frame Disabled {
            n489 = call "Power Supply Global.vi"("Closed Loop"=w1160, "PS Global Mode"=Power_Supply_Global_Mode."Write Setpoint", "PS Cmd"=w1155, "PS Voltage"=w1159, "VoltCtrlRef"=w1154) -> ()  [unwired: 6 in, 5 out]
            n490 = disable-structure shown="Enabled" {
              disable-tunnel: w1157 -> [w1175 w1176]
              disable-tunnel: [w1174 w1176] -> w1156
              disable-tunnel: w1153 -> [w1173 _]
              disable-tunnel: w1152 -> [w1172 _]
              disable-tunnel: w1151 -> [w1171 _]
              disable-tunnel: w1150 -> [w1170 _]
              disable-tunnel: w1149 -> [w1169 _]
              frame Disabled {
                n491 = call "Write FPGA Outputs.vi"("FPGA Ref"=w1175, "Tank CMDs"=w1173, "App Config"=w1172, "Power Relay"=w1171, "Ignition Relay"=w1170, "Voltage Enable"=w1169) -> ("FPGA Ref OUT"=w1174:T48)  [unwired: 13 in]
              }
              frame Enabled {
              }
            }
            n492 = case shown="\"Kuhnke\", \"Helbako BLDC\", \"PSA\", Default" w1168 {
              selector: w1168 -> [_ w1188]
              tunnel: w1156 -> [w1183 _]
              tunnel: w1167 -> [_ w1192]
              tunnel: w1166 -> [w1182 _]
              tunnel: w1165 -> [w1181 w1190]
              tunnel: w1164 -> [w1180 _]
              tunnel: w1163 -> [w1179 _]
              tunnel: w1162 -> [w1178 _]
              tunnel: [w1177 w1190] -> w1161
              tunnel: w1151 -> [_ w1187]
              tunnel: w1150 -> [_ w1186]
              frame "Kuhnke", "Helbako BLDC", "PSA", Default {
                n493 = call "Write PWM Outputs.vi"("FPGE Ref"=w1183, "Frequency"=w1182, "Controller CMDs IN"=w1181, "Stagger Counter"=w1180, "Stagger Time (ms)"=w1179, "Run Profile"=w1178) -> ("Controller CMDs OUT"=w1177:dbl[])  [unwired: 13 in]
              }
              frame "Conti".."Hella BLDC Pressure" {
                n494 = Cluster To Array(cluster=w1192) -> (array=w1185:bool[])
                n495 = Search 1D Array(1D array=w1185, element=TRUE) -> (index of element=w1191:i32)  [unwired: 1 in]
                n496 = Less Than 0?(x=w1191) -> (x < 0?=w1196:bool)
                n497 = Select(t=0, s=w1196, f=w1191) -> (s? t:f=w1194:i32)
                n498 = Index Array(array=w1190, index=w1194) -> (element=w1184:dbl)
                n499 = call "CAN Global.vi"("Controller Type:"=w1188, "Write (F)"=TRUE, "CAN Cmd"=w1184, "Power Relay"=w1187, "Ignition Relay"=w1186) -> ()  [unwired: 7 in, 4 out]
              }
            }
          }
          frame Enabled {
          }
        }
        n500 = Multiply(x=w1108, y=w1102) -> (x*y=w1107:dbl)
        n501 = To Unsigned Long Integer(number=w1106) -> (unsigned 32bit integer=w1104:u32)
        n502 = To Long Integer(number=w1107) -> (32bit integer=w1105:i32)
        n503 = Insert Into Array(array=w1098, index=0, new element=w1096) -> (w1095:bool[])
        n504 = Not(x=w1092) -> (.not. x?=w1091:bool)
        n505 = And(x=w1095, y=w1092) -> (x .and. y?=w1094:bool[])
        n506 = And(x=w1095, y=w1091) -> (x .and. y?=w1090:bool[])
        n507 = To Fixed-Point(fixed-point type=w1081, number=w1084) -> (fixed-point=w1082:fxp<+/-,28,17>)
        n508 = To Fixed-Point(fixed-point type=w1081, number=w1085) -> (fixed-point=w1083:fxp<+/-,28,17>)
        n509 = xnode "Read/Write Control"("FPGA VI Reference In"=w1086, "Enable Readings"=w1095, "Enable Cycles"=w1094, "Enable Anomalies"=w1094, "Enable Opens"=w1090, "Bank1(Pulse/Const)"=w1099, "Bank1Const(On/Off)"=w1088, "Bank2(Pulse/Const)"=w1101, "Bank2Const(On/Off)"=w1089, "PWM Period (Ticks)"=w1104, "Duty (Ticks)"=w1105, "Normal Steps"=w1087, "Anomaly Threshold"=w1082, "Step Threshold"=w1083, "Enable2ndStepCheck"=w1080, "Subtract Noise"="Subtract Noise") -> ()  [unwired: 1 in, 2 out]
        n510 = Bundle By Name(cluster=w1129, "Controller CMDs"=w1127) -> (w1128:T26)
        n511 = Insert Into Array(array=w1116, index=0, new element=w1114) -> (w1115:T15[])
      }
      frame "Read Inputs" {
        w1201 = FALSE ("WebDAV Push")
        n512 = Unbundle By Name(w1247) -> ("Concat Data"=w1202:bool, "WebDAV Push"=w1212:bool, "Current Step"=w1211:i32, "Step Time Left"=w1210:dbl, "Run Profile"=w1230:bool, "Controller Config"=w1225:T23, "Trip Counters"=w1240:i32[], "Previous Times"=w1239:u32[], "Prev ON Times"=w1238:u32[], "Alarm Config"=w1241:T10, "Alarm Message 2"=w1234:string, "Alarm Message 1"=w1235:string, "Alarm Latch"=w1236:bool, "App Config.Pumps Present"=w1223:T8, "Power Relay"=w1242:T8, "Controller CMDs"=w1226:dbl[], "App Config"=w1227:T6, "Tank CMDs"=w1228:T20, "Time/Date"=w1231:string, "Run Profile"=w1224:bool, "Recording"=w1233:bool, "Power Relay"=w1229:T8, "App Config.ADC Check"=w1204:bool, "Initial LS Data"=w1199:T16)
        n513 = Cluster To Array(cluster=w1223) -> (array=w1208:bool[])
        n514 = call "Tank Data Global.vi"() -> ("Tank Data OUT"=w1246:dbl[], "Pump Data"=w1214:T18, "Tank Data"=w1213:T24, "Record Time (sec)"=w1203:dbl)  [unwired: 12 in]
        n515 = disable-structure shown="Enabled" {
          disable-tunnel: w1198 -> [w1257 _]
          disable-tunnel: w1228 -> [w1256 _]
          disable-tunnel: w1227 -> [w1255 _]
          disable-tunnel: w1226 -> [w1254 _]
          disable-tunnel: w1225 -> [w1253 _]
          disable-tunnel: w1224 -> [w1252 _]
          disable-tunnel: w1213 -> [w1251 _]
          disable-tunnel: [w1250 _] -> w1209
          disable-tunnel: w1208 -> [w1249 _]
          disable-tunnel: [w1248 _] -> w1206
          frame Disabled {
            n516 = call "Enable Timers.vi"("FPGA Ref"=w1257, "Tank Data"=w1251, "Tank CMDs"=w1256, "App Config"=w1255, "Controller CMDs"=w1254, "Controller Config"=w1253, "Run Profile"=w1252, "Pumps Present"=w1249) -> ("In Spec"=w1250:bool[], "Reset ADCs"=w1248:bool)  [unwired: 18 in]
          }
          frame Enabled {
          }
        }
        n517 = call "Evaluate Alarms.vi"("In Test"=w1230, "Controller"=w1225, "Alarm Config"=w1241, "Data"=w1246, "Pumps Present"=w1208, "Trip Counter"=w1240, "Previous Times"=w1239, "Manual CMDs"=w1226, "Prev ON Times"=w1238) -> ("Trip Counter OUT"=w1245:i32[], "Previous Times OUT"=w1244:u32[], "Alarm Tripped"=w1216:bool, "Prev ON Times OUT"=w1243:u32[], "Alarm Message 1"=w1221:string, "Alarm Message 2"=w1220:string)  [unwired: 13 in]
        n518 = call "RPi HMI Com.vi"("Pump Data"=w1214, "Tank Data"=w1213, "Power Relays"=w1242, "Pump CMDs"=w1226, "App Config"=w1227, "Tank CMDs"=w1228, "Alarm"=w1236, "RPi HMI Mode"=RPi_HMI_Mode."Write Data", "In Test"=w1224, "Alarm Message 1"=w1235, "Controller Config"=w1225, "Alarm Message 2"=w1234, "Recording"=w1233, "Pumps Present"=w1208, "Time/Date"=w1231) -> ()  [unwired: 4 in, 1 out]
        n519 = call "Freeze PID.vi"("Run Profile"=w1224, "Controller CMDs"=w1226, "Controller Config"=w1225, "Power Relay"=w1229) -> ()  [unwired: 12 in]
        n520 = call "Data Logger Global.vi"("WebDAV Push"=w1212, "In Spec"=w1209, "Current Step"=w1211, "Step Time Left"=w1210, "Pump Data"=w1214, "Tank Data"=w1213, "Concat Data"=w1202, "Record Time (sec)"=w1203, "Write (F)"=TRUE) -> ()  [unwired: 3 in, 8 out]
        n521 = call "Get OneHour LS Data.vi"("Initial LS Data"=w1199, "FPGA OneHour Ref"=w1198) -> ("LS Data"=w1200:T16)  [unwired: 9 in]
        n522 = flat-sequence {
          frame #0 {
            n523 = Tick Count (ms)() -> (millisecond timer value=w1260:u32)
            n524 = feedback #5() -> (w1259:u32)  [unwired: 1 in]
            n525 = feedback-in #5(w1260) -> ()
            n526 = Subtract(x=w1260, y=w1259) -> (x-y=→"Read Inputs (ms)":u32)
          }
        }
        n527 = And(x=w1206, y=w1204) -> (x .and. y?=w1205:bool)
        n528 = case shown="True" w1205 {
          tunnel: w1232 -> [w1266 w1270]
          tunnel: [w1266 w1269] -> w1218
          frame False {
          }
          frame True {
            n529 = Insert Into Array(array=w1270, index=0, new element=Sequence_States."Reinit ADC" ("new element/subarray")) -> (w1269:T15[])
          }
        }
        n530 = Tick Count (ms)() -> (millisecond timer value=w1207:u32)
        n531 = call "Get Time and Date.vi"() -> ("Time/Date"=w1219:string)  [unwired: 11 in]
        n532 = case shown="True" w1216 {
          tunnel: w1218 -> [w1261 w1265]
          tunnel: [w1261 w1264] -> w1217
          frame False {
          }
          frame True {
            w1262 = T15[] [enum."Stop Profile", enum."Update Screen", enum."Disable Background", enum."Alarm"] items=["Main", "Init Files", "Init", "Unused", "Save As", "Start Profile", "Check Step Time", "Alarm", "Alarm Dismiss", "Run Step", "Stop Profile", "Cycle Reset", "Time Reset", "Time Reset All", "Time Set", "Tare CTs", "Save Profile", "Open Profile", "Get Profiles", "Update Screen", "Update Controls", "Save App Config", "Write Outputs", "Disable Background", "Enable Background", "Get/Release Control", "Log Fuel Change", "Fuel Change Popup", "Read Inputs", "Remote Timer Reset", "Controller Change", "Get Alarms", "Init Alarms", "Save Alarms", "Voltage Selection", "Set Watlow Temp 1", "Set Watlow Temp 2", "Get Pressure", "Write Tare Pressure", "Adjust Controls", "Reinit ADC", "Write Initial Times", "Write Pumps Present", "HMI Command", "Save Pump Times", "Check Pump Stop Time", "Save LS App Config", "Init Data File", "Reset LS Cycles", "Reset Anomalies", "Reset Opens", "Save LS Data", "Save LS Test Data", "Check Serial Numbers", "Main Tab", "Allow Data Note"]
            n533 = Insert Into Array(array=w1265, index=0, new element=w1262) -> (w1264:T15[])
          }
        }
        n534 = Bundle By Name(cluster=w1247, "Inputs Timer"=w1207, "Pump Data"=w1214, "Tank Data"=w1213, "Trip Counters"=w1245, "Previous Times"=w1244, "Alarm Latch"=w1216, "Prev ON Times"=w1243, "Alarm Message 1"=w1221, "Alarm Message 2"=w1220, "Time/Date"=w1219, "WebDAV Push"=w1201, "Concat Data"=w1201, "LS Data"=w1200) -> (w1222:T26)
      }
      frame "Update Screen" {
        n535 = Unbundle By Name(w1281) -> ("App Config.Cycles Completed"=→"Cycles Completed:":u32, "Current Step"=→"Current Step:":i32, "Step Time Left"=→"Step Time Left:":dbl, "Time/Date"=→"Time/Date":string, "Recording"=→"Recording":bool, "Pump Data"=w1283:T18, "Tank Data"=w1282:T24, "LS Data"=w1278:T16, "Run Profile"=w1288:bool)
        n536 = Unbundle(w1283) -> ("Voltages"=→"Voltages":dbl[], "PumpCurrent"=→"PumpCurrent":dbl[], "Speed"=→"Speed":dbl[], "ControllerCurrent"=→"ControllerCurrent":dbl[], "Pressure"=→"Pressure":dbl[], "Flow"=→"Flow":dbl[], "Elapsed Time (Display)"=→"Elapsed Time:":dbl[], "Avg Pressure"=→"Avg Press:":dbl, "Avg Speed"=→"Ave. Speed":dbl)  [unwired: 1 out]
        n537 = Unbundle(w1282) -> ("PS Actual (V):"=→"PS Actual (V):":dbl, "Temp1"=→"Temp1":dbl, "Temp2"=→"Temp2":dbl)
        n538 = Unbundle(w1278) -> ("Total Cycles"=→"Total Cycles":u32[], "Steps"=→"Steps":u32[], "Anomalies Total"=→"Anomalies Total":i32[], "Cycles"=→"Cycles":u32[], "Anomalies/Cycle"=→"Anomalies/Cycle":i32[], "Anomalies (Last Cycle)"=→"Anomalies (Last Cycle)":i32[], "Opens"=→"Opens":i32[])
        n539 = flat-sequence {
          frame #0 {
            n540 = Tick Count (ms)() -> (millisecond timer value=w1308:u32)
            n541 = feedback #6() -> (w1307:u32)  [unwired: 1 in]
            n542 = feedback-in #6(w1308) -> ()
            n543 = Subtract(x=w1308, y=w1307) -> (x-y=→"Update Screen (ms)":u32)
          }
        }
        n544 = case shown="True" w1288 {
          tunnel: [w1309 w1312] -> w1305
          tunnel: w1304 -> [w1309 w1311]
          frame False {
          }
          frame True {
            w1310 = T15[] [enum."Save Pump Times", enum."Update Controls"] items=["Main", "Init Files", "Init", "Unused", "Save As", "Start Profile", "Check Step Time", "Alarm", "Alarm Dismiss", "Run Step", "Stop Profile", "Cycle Reset", "Time Reset", "Time Reset All", "Time Set", "Tare CTs", "Save Profile", "Open Profile", "Get Profiles", "Update Screen", "Update Controls", "Save App Config", "Write Outputs", "Disable Background", "Enable Background", "Get/Release Control", "Log Fuel Change", "Fuel Change Popup", "Read Inputs", "Remote Timer Reset", "Controller Change", "Get Alarms", "Init Alarms", "Save Alarms", "Voltage Selection", "Set Watlow Temp 1", "Set Watlow Temp 2", "Get Pressure", "Write Tare Pressure", "Adjust Controls", "Reinit ADC", "Write Initial Times", "Write Pumps Present", "HMI Command", "Save Pump Times", "Check Pump Stop Time", "Save LS App Config", "Init Data File", "Reset LS Cycles", "Reset Anomalies", "Reset Opens", "Save LS Data", "Save LS Test Data", "Check Serial Numbers", "Main Tab", "Allow Data Note"]
            n545 = Insert Into Array(array=w1311, index=0, new element=w1310) -> (w1312:T15[])
          }
        }
        n546 = call "App Global.vi"() -> ("CPU Usage OUT"=→"CPU Usage:":dbl, "Login OUT"=w1284:bool)  [unwired: 9 in, 1 out]
        n547 = Tick Count (ms)() -> (millisecond timer value=w1279:u32)
        n548 = local write "Login"(w1284) -> ()
        n549 = Bundle By Name(cluster=w1281, "Screen Timer"=w1279) -> (w1280:T26)
      }
      frame "Update Controls" {
        w1338 = bool[] [FALSE, FALSE, FALSE, FALSE, FALSE, FALSE] ("pb.Resets")
        w1339 = T15[] [] items=["Main", "Init Files", "Init", "Unused", "Save As", "Start Profile", "Check Step Time", "Alarm", "Alarm Dismiss", "Run Step", "Stop Profile", "Cycle Reset", "Time Reset", "Time Reset All", "Time Set", "Tare CTs", "Save Profile", "Open Profile", "Get Profiles", "Update Screen", "Update Controls", "Save App Config", "Write Outputs", "Disable Background", "Enable Background", "Get/Release Control", "Log Fuel Change", "Fuel Change Popup", "Read Inputs", "Remote Timer Reset", "Controller Change", "Get Alarms", "Init Alarms", "Save Alarms", "Voltage Selection", "Set Watlow Temp 1", "Set Watlow Temp 2", "Get Pressure", "Write Tare Pressure", "Adjust Controls", "Reinit ADC", "Write Initial Times", "Write Pumps Present", "HMI Command", "Save Pump Times", "Check Pump Stop Time", "Save LS App Config", "Init Data File", "Reset LS Cycles", "Reset Anomalies", "Reset Opens", "Save LS Data", "Save LS Test Data", "Check Serial Numbers", "Main Tab", "Allow Data Note"]
        n550 = Unbundle By Name(w1341) -> ("App Config.Stagger Time (ms)"=w1350:i32, "Profile"=w1351:string[][], "App Config.Current Profile"=w1346:string, "App Config.CA Number"=w1345:string, "App Config.Controller Type:"=w1352:T3, "App Config.Pumps Present"=w1342:T8, "App Config.Tank 1 Fuel"=w1349:string, "App Config.Tank 2 Fuel"=w1348:string, "App Config.Serial Numbers"=w1347:T41, "App Config.Target Voltage"=w1344:dbl, "App Config.Target Pressure"=w1343:dbl, "Email Alarms Disabled"=w1337:bool, "Run Profile"=w1336:bool, "Recording"=w1335:bool, "Tank CMDs.Press CMD"=w1334:dbl, "Controller CMDs"=w1333:dbl[], "Tank CMDs.PS CMD"=w1332:dbl, "Power Relay"=w1331:T8, "Ignition Relay"=w1316:T8, "WebDAV Push"=w1315:bool, "Concat Data"=w1314:bool, "LS App Config.LS Power (Freq):"=w1320:dbl, "LS App Config.LS Power (Duty):"=w1319:dbl, "LS App Config.Bank 1 Present"=w1318:T2, "LS App Config.Bank 2 Present"=w1317:T1, "LS App Config.Data File Name:"=w1321:string, "LS App Config.Record Bursts"=w1330:bool, "LS App Config.RecInterval(s)"=w1329:i32, "LS App Config.RecDuration(s)"=w1328:i32, "LS App Config.RecFrequeny (Hz)"=w1327:i32, "LS App Config.DetectionMode"=w1326:i32, "LS App Config.Serial Numbers"=w1325:string[], "Bank 1 State:"=w1323:u16, "Bank 2 State:"=w1322:u16)
        n551 = Array To Cluster(array=w1325) -> (cluster=w1324:T49)
        n552 = local write "LS Power (Freq):"(w1320) -> ()
        n553 = local write "LS Power (Duty):"(w1319) -> ()
        n554 = local write "Bank 1"(w1318) -> ()
        n555 = local write "Bank 2"(w1317) -> ()
        n556 = local write "Data File Name:"(w1321) -> ()
        n557 = local write "Record During Profile"(w1330) -> ()
        n558 = local write "Interval Between\nRecordings (s):"(w1329) -> ()
        n559 = local write "Recording\nDuration (s):"(w1328) -> ()
        n560 = local write "Recording\nFrequency (Hz):"(w1327) -> ()
        n561 = local write "Detection Mode:"(w1326) -> ()
        n562 = local write "LS Serial Numbers"(w1324) -> ()
        n563 = local write "Bank 1 Power State:"(w1323) -> ()
        n564 = local write "Bank 2 Power State:"(w1322) -> ()
        n565 = local write "pb.Run Profile"(w1336) -> ()
        n566 = local write "Recording"(w1335) -> ()
        n567 = local write "PressureCMD"(w1334) -> ()
        n568 = local write "Controller\nCMD"(w1333) -> ()
        n569 = local write "Power Supply Cmd:"(w1332) -> ()
        n570 = local write "Power Relay"(w1331) -> ()
        n571 = local write "Ignition Relay"(w1316) -> ()
        n572 = local write "WebDAV Push"(w1315) -> ()
        n573 = local write "Concat Data"(w1314) -> ()
        n574 = local write "pb.Resets"(w1338) -> ()
        n575 = local write "pb.Sets"(w1338) -> ()
        n576 = case shown="False" w1336 {
          tunnel: w1352 -> [w1366 _]
          tunnel: w1351 -> [w1365 _]
          tunnel: w1350 -> [w1364 _]
          tunnel: w1349 -> [w1363 _]
          tunnel: w1348 -> [w1362 _]
          tunnel: w1347 -> [w1361 _]
          tunnel: w1346 -> [w1360 _]
          tunnel: w1345 -> [w1359 _]
          tunnel: w1344 -> [w1358 _]
          tunnel: w1343 -> [w1357 _]
          tunnel: w1342 -> [w1356 _]
          tunnel: w1337 -> [w1355 _]
          frame False {
            n577 = local write "Stagger Time (ms):"(w1364) -> ()
            n578 = local write "Profile:"(w1365) -> ()
            n579 = local write "Profile Name:"(w1360) -> ()
            n580 = local write "CA Number:"(w1359) -> ()
            n581 = local write "Controller Type:"(w1366) -> ()
            n582 = local write "Pumps Present"(w1356) -> ()
            n583 = local write "Tank 1 Fuel Type:"(w1363) -> ()
            n584 = local write "Tank 2 Fuel Type:"(w1362) -> ()
            n585 = local write "Serial Numbers"(w1361) -> ()
            n586 = local write "Target Voltage:"(w1358) -> ()
            n587 = local write "Target Pressure:"(w1357) -> ()
            n588 = local write "Disable Alarm Email"(w1355) -> ()
            "Email Alarms Disabled" <- w1355
          }
          frame True {
          }
        }
        n589 = Insert Into Array(array=w1353, index=0, new element=w1339) -> (w1354:T15[])
      }
      frame "Check Pump Stop Time" {
        n590 = Unbundle By Name(w1376) -> ("Pump Data.Elapsed Time"=w1368:dbl[], "App Config.Pumps Present"=w1370:T8)
        n591 = Cluster To Array(cluster=w1370) -> (array=w1369:bool[])
        n592 = for {
          tunnel: w1369 -> [w1377] mode=indexing
          tunnel: w1368 -> [w1378] mode=indexing
          tunnel: [w1378] -> w1367 mode=indexing if=w1377
        }
        n593 = Array Max & Min(array=w1367) -> (min value=w1375:dbl)  [unwired: 3 out]
        n594 = Greater?(x=w1375, y="Stop Time:") -> (0:w1371:bool)
        n595 = case shown="True" w1371 {
          tunnel: w1373 -> [w1379 w1381]
          tunnel: [w1379 w1380] -> w1372
          frame False {
          }
          frame True {
            w1382 = T15[] [enum."Stop Profile"] items=["Main", "Init Files", "Init", "Unused", "Save As", "Start Profile", "Check Step Time", "Alarm", "Alarm Dismiss", "Run Step", "Stop Profile", "Cycle Reset", "Time Reset", "Time Reset All", "Time Set", "Tare CTs", "Save Profile", "Open Profile", "Get Profiles", "Update Screen", "Update Controls", "Save App Config", "Write Outputs", "Disable Background", "Enable Background", "Get/Release Control", "Log Fuel Change", "Fuel Change Popup", "Read Inputs", "Remote Timer Reset", "Controller Change", "Get Alarms", "Init Alarms", "Save Alarms", "Voltage Selection", "Set Watlow Temp 1", "Set Watlow Temp 2", "Get Pressure", "Write Tare Pressure", "Adjust Controls", "Reinit ADC", "Write Initial Times", "Write Pumps Present", "HMI Command", "Save Pump Times", "Check Pump Stop Time", "Save LS App Config", "Init Data File", "Reset LS Cycles", "Reset Anomalies", "Reset Opens", "Save LS Data", "Save LS Test Data", "Check Serial Numbers", "Main Tab", "Allow Data Note"]
            n596 = Insert Into Array(array=w1381, index=0, new element=w1382) -> (w1380:T15[])
          }
        }
      }
      frame "Stop Profile" {
        w1390 = u16 0 items=["0 - Off", "1 - On", "2 - Pulsing"] ("Bank 1 Power State:")
        w1391 = FALSE
        w1389 = FALSE ("Running?")
        w1402 = T15[] [enum."Write Outputs", enum."Update Controls"] items=["Main", "Init Files", "Init", "Unused", "Save As", "Start Profile", "Check Step Time", "Alarm", "Alarm Dismiss", "Run Step", "Stop Profile", "Cycle Reset", "Time Reset", "Time Reset All", "Time Set", "Tare CTs", "Save Profile", "Open Profile", "Get Profiles", "Update Screen", "Update Controls", "Save App Config", "Write Outputs", "Disable Background", "Enable Background", "Get/Release Control", "Log Fuel Change", "Fuel Change Popup", "Read Inputs", "Remote Timer Reset", "Controller Change", "Get Alarms", "Init Alarms", "Save Alarms", "Voltage Selection", "Set Watlow Temp 1", "Set Watlow Temp 2", "Get Pressure", "Write Tare Pressure", "Adjust Controls", "Reinit ADC", "Write Initial Times", "Write Pumps Present", "HMI Command", "Save Pump Times", "Check Pump Stop Time", "Save LS App Config", "Init Data File", "Reset LS Cycles", "Reset Anomalies", "Reset Opens", "Save LS Data", "Save LS Test Data", "Check Serial Numbers", "Main Tab", "Allow Data Note"]
        w1407 = T8 {"Pump 1"=FALSE, "Pump 2"=FALSE, "Pump 3"=FALSE, "Pump 4"=FALSE, "Pump 5"=FALSE, "Pump 6"=FALSE} ("Power Relay")
        n597 = Unbundle By Name(w1406) -> ("Controller Config.Stop Command"=w1405:dbl, "LS App Config.Record Bursts"=w1396:bool, "LS App Config.RecInterval(s)"=w1395:i32, "LS App Config.RecDuration(s)"=w1394:i32, "LS App Config.RecFrequeny (Hz)"=w1393:i32, "LS Data Filepath"=w1392:path, "LS App Config.Record Constant"=w1386:bool, "LS App Config.Serial Numbers"=w1385:string[], "Login"=w1388:bool)
        n598 = Bundle(cluster=T30 {"Running?"=FALSE, "Profile Record"=FALSE, "RecordInterval"=0, "RecordDuration"=0, "RecordFreq"=0, "Data Filepath"=path "", "Hr Record"=FALSE, "Serial Numbers"=[]} ("LS Cluster In"), "Running?"=w1389, "Profile Record"=w1396, "RecordInterval"=w1395, "RecordDuration"=w1394, "RecordFreq"=w1393, "Data Filepath"=w1392, "Hr Record"=w1386, "Serial Numbers"=w1385) -> (w1397:T30)
        n599 = call "LS Data Global.vi"("Mode"=enum16{"Read", "Engine Writes", "Main Writes"}."Main Writes", "LS Cluster In"=w1397) -> ()  [unwired: 12 in, 2 out]
        n600 = case shown="True" w1388 {
          frame False {
          }
          frame True {
            w1413 = T31."Enabled" ("Disabled")
            n601 = property on="Bank 1" class="Clust (strict)"("DisabledEnum"=w1413) -> ()  [unwired: 2 in, 2 out]
            n602 = property on="Bank 2" class="Clust (strict)"("DisabledEnum"=w1413) -> ()  [unwired: 2 in, 2 out]
            n603 = property on="Live Data Tab" class="TabCtl (strict)"("DisabledEnum"=w1413) -> ()  [unwired: 2 in, 2 out]
            n604 = property on="Pump Timers Tab" class="TabCtl (strict)"("DisabledEnum"=w1413) -> ()  [unwired: 2 in, 2 out]
          }
        }
        n605 = disable-structure shown="Disabled" {
          frame Disabled {
            n606 = call "Data Logger Main.vi"("Data Logger Mode"=Data_Logger_Mode."Stop") -> ()  [unwired: 19 in]
          }
          frame Enabled {
          }
        }
        n607 = local write "Stop Time Enable"(FALSE ("Stop Time Enable")) -> ()
        n608 = Initialize Array(w1405, 6 ("dimension size")) -> (w1403:dbl[])
        n609 = property on="Time:" class="DigNum (strict)"("Visible"=w1391) -> ()  [unwired: 2 in, 2 out]
        n610 = property on="Step:" class="DigNum (strict)"("Visible"=w1391) -> ()  [unwired: 2 in, 2 out]
        n611 = local write "Bank 1 Power State:"(w1390) -> ()
        n612 = local write "Bank 2 Power State:"(w1390) -> ()
        n613 = Bundle By Name(cluster=w1406, "pb.Run Profile"=w1389, "Run Profile"=FALSE, "Controller CMDs"=w1403, "Power Relay"=w1407, "Ignition Relay"=w1407, "Tank CMDs.Press CMD"=0.0, "Recording"=FALSE, "Bank 1 State:"=w1390, "Bank 2 State:"=w1390) -> (w1400:T26)
        n614 = Insert Into Array(array=w1410, index=0, new element=w1402) -> (w1409:T15[])
      }
      frame "Save As" {
        n615 = property on="Save As Tab" class="TabCtl (strict)"("Visible"=TRUE) -> (error out=w1418:errorcluster)  [unwired: 2 in, 1 out]
        n616 = while {
          tunnel: ["pb.Save As OK"] -> w1424
          tunnel: w1418 -> [_]
          stop <- w1426 stop-if-true
          n617 = Wait (ms)(milliseconds to wait=u32 10) -> ()  [unwired: 1 out]
          n618 = Or(x="pb.Save As OK", y="pb.Save As Cancel") -> (x .or. y?=w1426:bool)
        }
        n619 = Unbundle By Name(w1422) -> ("App Config.Profiles Path"=w1423:path, "Profile"=w1420:string[][])
        n620 = case shown="True" w1424 {
          tunnel: w1423 -> [_ w1434]
          tunnel: [w1429 w1431] -> w1415
          tunnel: w1422 -> [w1430 w1436]
          tunnel: [w1430 w1435] -> w1421
          tunnel: w1420 -> [_ w1433]
          frame False {
            w1429 = T15[] [enum."Enable Background"] items=["Main", "Init Files", "Init", "Unused", "Save As", "Start Profile", "Check Step Time", "Alarm", "Alarm Dismiss", "Run Step", "Stop Profile", "Cycle Reset", "Time Reset", "Time Reset All", "Time Set", "Tare CTs", "Save Profile", "Open Profile", "Get Profiles", "Update Screen", "Update Controls", "Save App Config", "Write Outputs", "Disable Background", "Enable Background", "Get/Release Control", "Log Fuel Change", "Fuel Change Popup", "Read Inputs", "Remote Timer Reset", "Controller Change", "Get Alarms", "Init Alarms", "Save Alarms", "Voltage Selection", "Set Watlow Temp 1", "Set Watlow Temp 2", "Get Pressure", "Write Tare Pressure", "Adjust Controls", "Reinit ADC", "Write Initial Times", "Write Pumps Present", "HMI Command", "Save Pump Times", "Check Pump Stop Time", "Save LS App Config", "Init Data File", "Reset LS Cycles", "Reset Anomalies", "Reset Opens", "Save LS Data", "Save LS Test Data", "Check Serial Numbers", "Main Tab", "Allow Data Note"]
          }
          frame True {
            w1431 = T15[] [enum."Enable Background", enum."Get Profiles"] items=["Main", "Init Files", "Init", "Unused", "Save As", "Start Profile", "Check Step Time", "Alarm", "Alarm Dismiss", "Run Step", "Stop Profile", "Cycle Reset", "Time Reset", "Time Reset All", "Time Set", "Tare CTs", "Save Profile", "Open Profile", "Get Profiles", "Update Screen", "Update Controls", "Save App Config", "Write Outputs", "Disable Background", "Enable Background", "Get/Release Control", "Log Fuel Change", "Fuel Change Popup", "Read Inputs", "Remote Timer Reset", "Controller Change", "Get Alarms", "Init Alarms", "Save Alarms", "Voltage Selection", "Set Watlow Temp 1", "Set Watlow Temp 2", "Get Pressure", "Write Tare Pressure", "Adjust Controls", "Reinit ADC", "Write Initial Times", "Write Pumps Present", "HMI Command", "Save Pump Times", "Check Pump Stop Time", "Save LS App Config", "Init Data File", "Reset LS Cycles", "Reset Anomalies", "Reset Opens", "Save LS Data", "Save LS Test Data", "Check Serial Numbers", "Main Tab", "Allow Data Note"]
            n621 = call "Save Profile.vi"("Profile"=w1433, "Current Profile"="New Profile Name:", "Profiles Path"=w1434) -> ()  [unwired: 8 in, 1 out]
            n622 = Bundle By Name(cluster=w1436, "App Config.Current Profile"="New Profile Name:") -> (w1435:T26)
          }
        }
        n623 = Insert Into Array(array=w1417, index=0, new element=w1415) -> (w1416:T15[])
      }
      frame "Save App Config" {
        n624 = Unbundle By Name(w1445) -> ("App Config"=w1444:T6)
        n625 = call <vilib>:"Open Config Data.vi"("create file if necessary (T)"=TRUE, "configuration file path"=path "c:/App Config.ini") -> ("error out"=w1438:errorcluster, "refnum"=w1442:T47)  [unwired: 7 in, 1 out]
        n626 = call "Read Write App Config.vi"("Write (F)"=TRUE, "Error IN"=w1438, "App Config"=w1444, "Refnum in"=w1442) -> ("Error OUT"=w1440:errorcluster, "Refnum out"=w1441:T47)  [unwired: 5 in, 1 out]
        n627 = call <vilib>:"Close Config Data.vi"("error in (no error)"=w1440, "refnum"=w1441) -> ()  [unwired: 8 in, 2 out]
      }
      frame "Save LS App Config" {
        n628 = Unbundle By Name(w1474) -> ("LS App Config"=w1456:T13, "pb.Run Profile"=w1467:bool, "LS App Config.Record Bursts"=w1452:bool, "LS App Config.RecInterval(s)"=w1466:i32, "LS App Config.RecDuration(s)"=w1465:i32, "LS App Config.RecFrequeny (Hz)"=w1464:i32, "LS Data Filepath"=w1462:path, "LS App Config.Record Constant"=w1453:bool, "LS App Config.Serial Numbers"=w1457:string[], "App Config.CA Number"=w1455:string, "LS App Config.Data File Name:"=w1454:string)
        n629 = Empty String/Path?(string/path=w1455) -> (empty?=w1460:bool)
        n630 = Empty String/Path?(string/path=w1454) -> (empty?=w1459:bool)
        n631 = call <vilib>:"Open Config Data.vi"("create file if necessary (T)"=TRUE, "configuration file path"=path "c:/LS App Config.ini") -> ("error out"=w1469:errorcluster, "refnum"=w1472:T47)  [unwired: 7 in, 1 out]
        n632 = Bundle By Name(cluster=T30 {"Running?"=FALSE, "Profile Record"=FALSE, "RecordInterval"=0, "RecordDuration"=0, "RecordFreq"=0, "Data Filepath"=path "", "Hr Record"=FALSE, "Serial Numbers"=[]} ("LS Cluster In"), "Running?"=w1467, "Profile Record"=w1452, "RecordInterval"=w1466, "RecordDuration"=w1465, "RecordFreq"=w1464, "Data Filepath"=w1462, "Hr Record"=w1453, "Serial Numbers"=w1457) -> (w1463:T30)
        n633 = Or(x=w1460, y=w1459) -> (x .or. y?=w1458:bool)
        n634 = call "Read Write LS App Config.vi"("Write (F)"=TRUE, "Error IN"=w1469, "LS App Config In"=w1456, "Refnum in"=w1472) -> ("Error OUT"=w1470:errorcluster, "Refnum out"=w1471:T47)  [unwired: 5 in, 1 out]
        n635 = case shown="False" w1458 {
          tunnel: w1453 -> [w1477 _]
          tunnel: w1452 -> [w1478 _]
          tunnel: [w1480 FALSE ("Record During Profile")] -> w1449
          tunnel: [w1479 T31."Disabled and Grayed Out" ("Disabled")] -> w1451
          tunnel: [w1482 FALSE ("Record During Profile")] -> w1448
          tunnel: [w1481 T31."Disabled and Grayed Out" ("Disabled")] -> w1450
          frame False {
            # "Valid file"
            n636 = And(x=w1478, y=w1477) -> (x .and. y?=w1483:bool)
            n637 = case shown="False" w1483 {
              tunnel: [w1484 FALSE] -> w1482
              tunnel: [w1488 T31."Enabled" ("Disabled")] -> w1481
              tunnel: [w1489 FALSE] -> w1480
              tunnel: [w1485 T31."Enabled" ("Disabled")] -> w1479
              tunnel: w1478 -> [w1484 _]
              tunnel: w1477 -> [w1489 _]
              frame False {
                n638 = Select(t=T31."Disabled and Grayed Out" ("Disabled"), s=w1489, f=T31."Enabled" ("Disabled")) -> (s? t:f=w1488:T31)
                n639 = Select(t=T31."Disabled and Grayed Out" ("Disabled"), s=w1484, f=T31."Enabled" ("Disabled")) -> (s? t:f=w1485:T31)
              }
              frame True {
                # "Reset allowing new selection"
                # "Error! - Cannot have both saves active"
              }
            }
          }
          frame True {
            # "Missing Data File Name/CA Number\nCannot Save"
          }
        }
        n640 = call <vilib>:"Close Config Data.vi"("error in (no error)"=w1470, "refnum"=w1471) -> ()  [unwired: 8 in, 2 out]
        n641 = call "LS Data Global.vi"("Mode"=enum16{"Read", "Engine Writes", "Main Writes"}."Main Writes", "LS Cluster In"=w1463) -> ()  [unwired: 12 in, 2 out]
        n642 = property on="Record During Profile" class="Bool (strict)"("Value"=w1448, "DisabledEnum"=w1450) -> ()  [unwired: 2 in, 2 out]
        n643 = property on="Record Constant" class="Bool (strict)"("Value"=w1449, "DisabledEnum"=w1451) -> ()  [unwired: 2 in, 2 out]
      }
      frame "Save Pump Times" {
        n644 = Unbundle By Name(w1504) -> ("Pump Data.Elapsed Time"=w1503:dbl[])
        n645 = Array Size(array=w1503) -> (size(s)=w1502:i32)
        n646 = Equal?(x=w1502, y=6) -> (x = y?=w1500:bool)
        n647 = case shown="True" w1500 {
          tunnel: w1503 -> [_ w1507]
          frame False {
          }
          frame True {
            n648 = Write to Binary File(file (use dialog)=path "c:/ElapsedTimes", data=w1507) -> (refnum out=w1508:refnum<file>, error out=w1509:errorcluster)  [unwired: 4 in, 1 out]
            n649 = Close File(refnum=w1508, error in=w1509) -> ()  [unwired: 2 out]
          }
        }
      }
      frame "Disable Background" {
        w1510 = T31."Disabled and Grayed Out" ("Disabled")
        n650 = property on="Main Tab" class="TabCtl (strict)"("DisabledEnum"=w1510) -> ()  [unwired: 2 in, 2 out]
        n651 = property on="pb.Stop Profile" class="Bool"("DisabledEnum"=w1510) -> ()  [unwired: 2 in, 2 out]
        n652 = property on="Monitoring Tab" class="TabCtl (strict)"("DisabledEnum"=w1510) -> ()  [unwired: 2 in, 2 out]
        n653 = property on="Title Tab" class="TabCtl (strict)"("DisabledEnum"=w1510) -> ()  [unwired: 2 in, 2 out]
        n654 = property on="CPU Usage:" class="DigNum (strict)"("DisabledEnum"=w1510) -> ()  [unwired: 2 in, 2 out]
        n655 = property on="Pump Timers Tab" class="TabCtl (strict)"("DisabledEnum"=w1510) -> ()  [unwired: 2 in, 2 out]
        n656 = property on="Live Data Tab" class="TabCtl (strict)"("DisabledEnum"=w1510) -> ()  [unwired: 2 in, 2 out]
      }
      frame "Enable Background" {
        w1513 = FALSE ("Visible")
        w1514 = T31."Enabled" ("Disabled")
        n657 = disable-structure shown="Enabled" {
          disable-tunnel: w1516 -> [w1519 w1521]
          frame Disabled {
            n658 = xnode "Read/Write Control"("FPGA VI Reference In"=w1519, "Timer Resets"=bool[] [FALSE, FALSE, FALSE, FALSE, FALSE, FALSE] ("array")) -> ()  [unwired: 1 in, 2 out]
          }
          frame Enabled {
            w1520 = bool[] [FALSE, FALSE, FALSE, FALSE, FALSE, FALSE, FALSE, FALSE, FALSE, FALSE, FALSE, FALSE] ("Opens Resets")
            n659 = xnode "Read/Write Control"("FPGA VI Reference In"=w1521, "Opens Resets"=w1520, "Anomaly Resets"=w1520, "Cycle Resets"=w1520) -> ()  [unwired: 1 in, 2 out]
          }
        }
        n660 = property on="Save As Tab" class="TabCtl (strict)"("Visible"=w1513) -> ()  [unwired: 2 in, 2 out]
        n661 = property on="Reset Tab" class="TabCtl (strict)"("Visible"=w1513) -> ()  [unwired: 2 in, 2 out]
        n662 = property on="Set Time Tab" class="TabCtl (strict)"("Visible"=w1513) -> ()  [unwired: 2 in, 2 out]
        n663 = property on="Alarm Tab" class="TabCtl (strict)"("Visible"=w1513) -> ()  [unwired: 2 in, 2 out]
        n664 = property on="Fuel Change Tab" class="TabCtl (strict)"("Visible"=w1513) -> ()  [unwired: 2 in, 2 out]
        n665 = property on="Note Tab" class="TabCtl (strict)"("Visible"=w1513) -> ()  [unwired: 2 in, 2 out]
        n666 = property on="Main Tab" class="TabCtl (strict)"("DisabledEnum"=w1514) -> ()  [unwired: 2 in, 2 out]
        n667 = property on="pb.Stop Profile" class="Bool"("DisabledEnum"=w1514) -> ()  [unwired: 2 in, 2 out]
        n668 = property on="Monitoring Tab" class="TabCtl (strict)"("DisabledEnum"=w1514) -> ()  [unwired: 2 in, 2 out]
        n669 = property on="Title Tab" class="TabCtl (strict)"("DisabledEnum"=w1514) -> ()  [unwired: 2 in, 2 out]
        n670 = property on="CPU Usage:" class="DigNum (strict)"("DisabledEnum"=w1514) -> ()  [unwired: 2 in, 2 out]
        n671 = property on="Alarm Tab" class="TabCtl (strict)"("DisabledEnum"=w1514) -> ()  [unwired: 2 in, 2 out]
        n672 = property on="Pump Timers Tab" class="TabCtl (strict)"("DisabledEnum"=w1514) -> ()  [unwired: 2 in, 2 out]
        n673 = property on="Live Data Tab" class="TabCtl (strict)"("DisabledEnum"=w1514) -> ()  [unwired: 2 in, 2 out]
      }
      frame "Cycle Reset".."Time Reset All", "Reset LS Cycles".."Reset Opens" {
        w1526 = T15[] [enum."Enable Background", enum."Write Initial Times"] items=["Main", "Init Files", "Init", "Unused", "Save As", "Start Profile", "Check Step Time", "Alarm", "Alarm Dismiss", "Run Step", "Stop Profile", "Cycle Reset", "Time Reset", "Time Reset All", "Time Set", "Tare CTs", "Save Profile", "Open Profile", "Get Profiles", "Update Screen", "Update Controls", "Save App Config", "Write Outputs", "Disable Background", "Enable Background", "Get/Release Control", "Log Fuel Change", "Fuel Change Popup", "Read Inputs", "Remote Timer Reset", "Controller Change", "Get Alarms", "Init Alarms", "Save Alarms", "Voltage Selection", "Set Watlow Temp 1", "Set Watlow Temp 2", "Get Pressure", "Write Tare Pressure", "Adjust Controls", "Reinit ADC", "Write Initial Times", "Write Pumps Present", "HMI Command", "Save Pump Times", "Check Pump Stop Time", "Save LS App Config", "Init Data File", "Reset LS Cycles", "Reset Anomalies", "Reset Opens", "Save LS Data", "Save LS Test Data", "Check Serial Numbers", "Main Tab", "Allow Data Note"]
        n674 = property on="Reset Tab" class="TabCtl (strict)"("Visible"=TRUE) -> (error out=w1522:errorcluster)  [unwired: 2 in, 1 out]
        n675 = while {
          tunnel: ["pb.Reset OK"] -> w1524
          tunnel: w1522 -> [_]
          stop <- w1601 stop-if-true
          n676 = Wait (ms)(milliseconds to wait=u32 10) -> ()  [unwired: 1 out]
          n677 = Or(x="pb.Reset Cancel", y="pb.Reset OK") -> (x .or. y?=w1601:bool)
        }
        n678 = disable-structure shown="Enabled" {
          disable-tunnel: [w1541 w1571] -> w1532
          disable-tunnel: w1531 -> [w1540 w1569]
          disable-tunnel: w1530 -> [w1539 w1567]
          disable-tunnel: w1529 -> [w1538 w1570]
          disable-tunnel: w1524 -> [w1537 w1568]
          frame Disabled {
            n679 = Unbundle By Name(w1539) -> ("pb.Resets"=w1536:bool[], "Initial Times"=w1533:dbl[])
            n680 = Search 1D Array(1D array=w1536, element=TRUE) -> (index of element=w1534:i32)  [unwired: 1 in]
            n681 = case shown="True" w1537 {
              tunnel: [w1542 w1548] -> w1541
              tunnel: w1539 -> [w1542 w1547]
              tunnel: w1534 -> [_ w1546]
              tunnel: w1533 -> [_ w1545]
              tunnel: w1540 -> [_ w1544]
              tunnel: w1538 -> [_ w1543]
              frame False {
              }
              frame True {
                n682 = case shown="\"Time Reset\"" w1543 {
                  tunnel: w1547 -> [w1551 w1561 w1566]
                  tunnel: [w1550 w1560 w1565] -> w1548
                  tunnel: w1546 -> [_ w1556 _]
                  tunnel: w1545 -> [_ w1559 _]
                  tunnel: w1544 -> [_ w1554 w1564]
                  frame "Cycle Reset", Default {
                    n683 = Bundle By Name(cluster=w1551, "App Config.Cycles Completed"=u32 0) -> (w1550:T26)
                  }
                  frame "Time Reset" {
                    n684 = Replace Array Subset(array=w1559, new element=0.0 ("new element/subarray"), index=w1556) -> (w1552:dbl[])
                    n685 = Replace Array Subset(array=bool[] [FALSE, FALSE, FALSE, FALSE, FALSE, FALSE], new element=TRUE ("new element/subarray"), index=w1556) -> (w1557:bool[])
                    n686 = xnode "Read/Write Control"("FPGA VI Reference In"=w1554, "Timer Resets"=w1557) -> ()  [unwired: 1 in, 2 out]
                    n687 = Bundle By Name(cluster=w1561, "Initial Times"=w1552) -> (w1560:T26)
                  }
                  frame "Time Reset All" {
                    n688 = xnode "Read/Write Control"("FPGA VI Reference In"=w1564, "Timer Resets"=bool[] [TRUE, TRUE, TRUE, TRUE, TRUE, TRUE] ("array")) -> ()  [unwired: 1 in, 2 out]
                    n689 = Bundle By Name(cluster=w1566, "Initial Times"=dbl[] [0.0, 0.0, 0.0, 0.0, 0.0, 0.0] ("Intitial Times")) -> (w1565:T26)
                  }
                }
              }
            }
          }
          frame Enabled {
            n690 = case shown="True" w1568 {
              tunnel: [w1572 w1576] -> w1571
              tunnel: w1567 -> [w1572 w1575]
              tunnel: w1569 -> [_ w1574]
              tunnel: w1570 -> [_ w1573]
              frame False {
              }
              frame True {
                n691 = case shown="\"Reset Opens\"" w1573 {
                  tunnel: w1575 -> [w1580 w1588 w1595 w1599]
                  tunnel: [w1579 w1587 w1594 w1599] -> w1576
                  tunnel: w1574 -> [w1578 w1586 w1593 _]
                  frame "Reset LS Cycles" {
                    n692 = flat-sequence {
                      tunnel: w1578 -> [w1582]
                      frame #0 {
                        n693 = xnode "Read/Write Control"("FPGA VI Reference In"=w1582, "Cycle Resets"=bool[] [TRUE, TRUE, TRUE, TRUE, TRUE, TRUE, TRUE, TRUE, TRUE, TRUE, TRUE, TRUE] ("Opens Resets")) -> ()  [unwired: 1 in, 2 out]
                      }
                      frame #1 {
                        n694 = Wait (ms)(milliseconds to wait=u32 5) -> ()  [unwired: 1 out]
                      }
                    }
                    n695 = Bundle By Name(cluster=w1580, "Initial LS Data.Total Cycles"=u32[] [0, 0, 0, 0, 0, 0, 0, 0, 0, 0, 0, 0]) -> (w1579:T26)
                  }
                  frame "Reset Anomalies" {
                    w1584 = i32[] [0, 0, 0, 0, 0, 0, 0, 0, 0, 0, 0, 0] ("Initial LS Data.Anomalies (Last Cycle)")
                    w1585 = u32[] [0, 0, 0, 0, 0, 0, 0, 0, 0, 0, 0, 0] ("Initial LS Data.Steps")
                    n696 = flat-sequence {
                      tunnel: w1586 -> [w1590]
                      frame #0 {
                        n697 = xnode "Read/Write Control"("FPGA VI Reference In"=w1590, "Anomaly Resets"=bool[] [TRUE, TRUE, TRUE, TRUE, TRUE, TRUE, TRUE, TRUE, TRUE, TRUE, TRUE, TRUE] ("Opens Resets")) -> ()  [unwired: 1 in, 2 out]
                      }
                      frame #1 {
                        n698 = Wait (ms)(milliseconds to wait=u32 5) -> ()  [unwired: 1 out]
                      }
                    }
                    n699 = Bundle By Name(cluster=w1588, "Initial LS Data.Steps"=w1585, "Initial LS Data.Anomalies Total"=w1584, "Initial LS Data.Cycles"=w1585, "Initial LS Data.Anomalies/Cycle"=w1584, "Initial LS Data.Anomalies (Last Cycle)"=w1584) -> (w1587:T26)
                  }
                  frame "Reset Opens" {
                    n700 = flat-sequence {
                      tunnel: w1593 -> [w1597]
                      frame #0 {
                        n701 = xnode "Read/Write Control"("FPGA VI Reference In"=w1597, "Opens Resets"=bool[] [TRUE, TRUE, TRUE, TRUE, TRUE, TRUE, TRUE, TRUE, TRUE, TRUE, TRUE, TRUE]) -> ()  [unwired: 1 in, 2 out]
                      }
                      frame #1 {
                        n702 = Wait (ms)(milliseconds to wait=u32 5) -> ()  [unwired: 1 out]
                      }
                    }
                    n703 = Bundle By Name(cluster=w1595, "Initial LS Data.Opens"=i32[] [0, 0, 0, 0, 0, 0, 0, 0, 0, 0, 0, 0]) -> (w1594:T26)
                  }
                  frame Default {
                  }
                }
              }
            }
          }
        }
        n704 = Insert Into Array(array=w1528, index=0, new element=w1526) -> (w1527:T15[])
      }
      frame "Alarm" {
        w1613 = T15[] [] items=["Main", "Init Files", "Init", "Unused", "Save As", "Start Profile", "Check Step Time", "Alarm", "Alarm Dismiss", "Run Step", "Stop Profile", "Cycle Reset", "Time Reset", "Time Reset All", "Time Set", "Tare CTs", "Save Profile", "Open Profile", "Get Profiles", "Update Screen", "Update Controls", "Save App Config", "Write Outputs", "Disable Background", "Enable Background", "Get/Release Control", "Log Fuel Change", "Fuel Change Popup", "Read Inputs", "Remote Timer Reset", "Controller Change", "Get Alarms", "Init Alarms", "Save Alarms", "Voltage Selection", "Set Watlow Temp 1", "Set Watlow Temp 2", "Get Pressure", "Write Tare Pressure", "Adjust Controls", "Reinit ADC", "Write Initial Times", "Write Pumps Present", "HMI Command", "Save Pump Times", "Check Pump Stop Time", "Save LS App Config", "Init Data File", "Reset LS Cycles", "Reset Anomalies", "Reset Opens", "Save LS Data", "Save LS Test Data", "Check Serial Numbers", "Main Tab", "Allow Data Note"]
        n705 = Unbundle By Name(w1604) -> ("Alarm Message 1"=w1609:string, "Alarm Message 2"=w1616:string, "App Config.Location"=w1617:string, "App Config.Email Handler IP"=w1606:string, "Email Alarms Disabled"=w1605:bool)
        n706 = Format Into String(format string="%s\n\n%s", w1609, w1616) -> (resulting string=w1614:string)  [unwired: 2 in, 1 out]
        n707 = Concatenate Strings(w1617, " ALARM!" ("string")) -> (w1615:string)
        n708 = case shown="False" w1605 {
          tunnel: w1615 -> [w1620 _]
          tunnel: w1614 -> [w1619 _]
          tunnel: w1606 -> [w1618 _]
          frame False {
            n709 = flat-sequence {
              tunnel: w1620 -> [w1624]
              tunnel: w1619 -> [w1623]
              tunnel: w1618 -> [w1621]
              frame #0 {
                n710 = call "Email to Handler.vi"("Email Mode"=Email_Mode."Trigger Email", "Email Handler IP"=w1621, "Message:"=w1623, "Subject:"=w1624) -> ()  [unwired: 8 in]
              }
              frame #1 {
                n711 = call "Email Global.vi"("Write (F)"=TRUE, "Send Email"=TRUE) -> ()  [unwired: 9 in, 1 out]
              }
            }
          }
          frame True {
          }
        }
        n712 = flat-sequence {
          tunnel: w1614 -> [w1627]
          frame #0 {
            "Alarm Message" <- w1627
          }
          frame #1 {
            n713 = property on="Alarm Tab" class="TabCtl (strict)"("Visible"=TRUE) -> ()  [unwired: 2 in, 2 out]
          }
        }
        n714 = Insert Into Array(array=w1611, index=0, new element=w1613) -> (w1610:T15[])
      }
      frame "Alarm Dismiss" {
        w1635 = T15[] [enum."Enable Background"] items=["Main", "Init Files", "Init", "Unused", "Save As", "Start Profile", "Check Step Time", "Alarm", "Alarm Dismiss", "Run Step", "Stop Profile", "Cycle Reset", "Time Reset", "Time Reset All", "Time Set", "Tare CTs", "Save Profile", "Open Profile", "Get Profiles", "Update Screen", "Update Controls", "Save App Config", "Write Outputs", "Disable Background", "Enable Background", "Get/Release Control", "Log Fuel Change", "Fuel Change Popup", "Read Inputs", "Remote Timer Reset", "Controller Change", "Get Alarms", "Init Alarms", "Save Alarms", "Voltage Selection", "Set Watlow Temp 1", "Set Watlow Temp 2", "Get Pressure", "Write Tare Pressure", "Adjust Controls", "Reinit ADC", "Write Initial Times", "Write Pumps Present", "HMI Command", "Save Pump Times", "Check Pump Stop Time", "Save LS App Config", "Init Data File", "Reset LS Cycles", "Reset Anomalies", "Reset Opens", "Save LS Data", "Save LS Test Data", "Check Serial Numbers", "Main Tab", "Allow Data Note"]
        n715 = Bundle By Name(cluster=w1631, "Alarm Latch"=FALSE) -> (w1630:T26)
        n716 = Insert Into Array(array=w1633, index=0, new element=w1635) -> (w1632:T15[])
      }
      frame "Time Set" {
        w1639 = T15[] [enum."Enable Background", enum."Write Initial Times"] items=["Main", "Init Files", "Init", "Unused", "Save As", "Start Profile", "Check Step Time", "Alarm", "Alarm Dismiss", "Run Step", "Stop Profile", "Cycle Reset", "Time Reset", "Time Reset All", "Time Set", "Tare CTs", "Save Profile", "Open Profile", "Get Profiles", "Update Screen", "Update Controls", "Save App Config", "Write Outputs", "Disable Background", "Enable Background", "Get/Release Control", "Log Fuel Change", "Fuel Change Popup", "Read Inputs", "Remote Timer Reset", "Controller Change", "Get Alarms", "Init Alarms", "Save Alarms", "Voltage Selection", "Set Watlow Temp 1", "Set Watlow Temp 2", "Get Pressure", "Write Tare Pressure", "Adjust Controls", "Reinit ADC", "Write Initial Times", "Write Pumps Present", "HMI Command", "Save Pump Times", "Check Pump Stop Time", "Save LS App Config", "Init Data File", "Reset LS Cycles", "Reset Anomalies", "Reset Opens", "Save LS Data", "Save LS Test Data", "Check Serial Numbers", "Main Tab", "Allow Data Note"]
        n717 = disable-structure shown="Disabled" {
          disable-tunnel: [w1653 w1671] -> w1642
          disable-tunnel: w1641 -> [w1652 w1671]
          disable-tunnel: w1640 -> [w1645 _]
          frame Disabled {
            n718 = Unbundle By Name(w1652) -> ("pb.Sets"=w1651:bool[], "Initial Times"=w1646:dbl[], "Pump Data.Elapsed Time"=w1649:dbl[])
            n719 = Search 1D Array(1D array=w1651, element=TRUE) -> (index of element=w1648:i32)  [unwired: 1 in]
            n720 = Index Array(array=w1649, index=w1648) -> (element=w1647:dbl)
            n721 = local write "New Time"(w1647) -> ()
            n722 = property on="Set Time Tab" class="TabCtl (strict)"("Visible"=TRUE) -> (error out=w1643:errorcluster)  [unwired: 2 in, 1 out]
            n723 = while {
              tunnel: ["pb.Set Time OK"] -> w1654
              tunnel: w1647 -> [_]
              tunnel: w1643 -> [_]
              stop <- w1657 stop-if-true
              n724 = Wait (ms)(milliseconds to wait=u32 10) -> ()  [unwired: 1 out]
              n725 = Or(x="pb.Set Time Cancel", y="pb.Set Time OK") -> (x .or. y?=w1657:bool)
            }
            n726 = case shown="True" w1654 {
              tunnel: w1652 -> [w1659 w1665]
              tunnel: [w1659 w1664] -> w1653
              tunnel: w1648 -> [_ w1661]
              tunnel: w1646 -> [_ w1663]
              tunnel: w1645 -> [_ w1662]
              frame False {
              }
              frame True {
                n727 = xnode "Read/Write Control"("FPGA VI Reference In"=w1662) -> ("FPGA VI Reference Out"=w1668:T27, "Timer Resets"=w1669)  [unwired: 1 in, 1 out]
                n728 = Replace Array Subset(array=w1663, new element="New Time", index=w1661) -> (w1670:dbl[])
                n729 = Replace Array Subset(array=w1669, new element=TRUE ("new element/subarray"), index=w1661) -> (w1667:bool[])
                n730 = Bundle By Name(cluster=w1665, "Initial Times"=w1670) -> (w1664:T26)
                n731 = xnode "Read/Write Control"("FPGA VI Reference In"=w1668, "Timer Resets"=w1667) -> ()  [unwired: 1 in, 2 out]
              }
            }
          }
          frame Enabled {
          }
        }
        n732 = Insert Into Array(array=w1637, index=0, new element=w1639) -> (w1636:T15[])
      }
      frame "Remote Timer Reset" {
        w1675 = T15[] [enum."Write Initial Times"] items=["Main", "Init Files", "Init", "Unused", "Save As", "Start Profile", "Check Step Time", "Alarm", "Alarm Dismiss", "Run Step", "Stop Profile", "Cycle Reset", "Time Reset", "Time Reset All", "Time Set", "Tare CTs", "Save Profile", "Open Profile", "Get Profiles", "Update Screen", "Update Controls", "Save App Config", "Write Outputs", "Disable Background", "Enable Background", "Get/Release Control", "Log Fuel Change", "Fuel Change Popup", "Read Inputs", "Remote Timer Reset", "Controller Change", "Get Alarms", "Init Alarms", "Save Alarms", "Voltage Selection", "Set Watlow Temp 1", "Set Watlow Temp 2", "Get Pressure", "Write Tare Pressure", "Adjust Controls", "Reinit ADC", "Write Initial Times", "Write Pumps Present", "HMI Command", "Save Pump Times", "Check Pump Stop Time", "Save LS App Config", "Init Data File", "Reset LS Cycles", "Reset Anomalies", "Reset Opens", "Save LS Data", "Save LS Test Data", "Check Serial Numbers", "Main Tab", "Allow Data Note"]
        n733 = disable-structure shown="Disabled" {
          disable-tunnel: w1678 -> [w1684 _]
          frame Disabled {
            n734 = xnode "Read/Write Control"("FPGA VI Reference In"=w1684, "Timer Resets"=bool[] [TRUE, TRUE, TRUE, TRUE, TRUE, TRUE] ("pb.Resets")) -> ("FPGA VI Reference Out"=w1682:T27)  [unwired: 1 in, 1 out]
            n735 = flat-sequence {
              tunnel: w1682 -> [w1685]
              tunnel: [w1685] -> w1681
              frame #0 {
                n736 = Wait (ms)(milliseconds to wait=u32 20) -> ()  [unwired: 1 out]
              }
            }
            n737 = xnode "Read/Write Control"("FPGA VI Reference In"=w1681, "Timer Resets"=bool[] [FALSE, FALSE, FALSE, FALSE, FALSE, FALSE] ("pb.Resets")) -> ()  [unwired: 1 in, 2 out]
          }
          frame Enabled {
          }
        }
        n738 = Bundle By Name(cluster=w1677, "Initial Times"=dbl[] [0.0, 0.0, 0.0, 0.0, 0.0, 0.0] ("Intitial Times")) -> (w1679:T26)
        n739 = Insert Into Array(array=w1672, index=0, new element=w1675) -> (w1673:T15[])
      }
      frame "Get/Release Control" {
        n740 = Unbundle By Name(w1691) -> ("Login"=w1689:bool)
        n741 = case shown="False" w1689 {
          tunnel: [T31."Disabled" ("Disabled") T31."Enabled" ("Disabled")] -> w1687
          frame False {
          }
          frame True {
          }
        }
        n742 = local write "Main Tab"(T9."Main" ("Main Tab")) -> ()
        n743 = property on="Main Tab" class="TabCtl (strict)"("DisabledEnum"=w1687) -> ()  [unwired: 2 in, 2 out]
        n744 = property on="Monitoring Tab" class="TabCtl (strict)"("DisabledEnum"=w1687) -> ()  [unwired: 2 in, 2 out]
        n745 = property on="Bank 1" class="Clust (strict)"("DisabledEnum"=w1687) -> ()  [unwired: 2 in, 2 out]
        n746 = property on="Bank 2" class="Clust (strict)"("DisabledEnum"=w1687) -> ()  [unwired: 2 in, 2 out]
        n747 = property on="Pump Timers Tab" class="TabCtl (strict)"("DisabledEnum"=w1687) -> ()  [unwired: 2 in, 2 out]
        n748 = property on="Live Data Tab" class="TabCtl (strict)"("DisabledEnum"=w1687) -> ()  [unwired: 2 in, 2 out]
        n749 = disable-structure shown="Disabled" {
          disable-tunnel: w1687 -> [w1692 _]
          frame Disabled {
            n750 = property on="pb.Stop Profile" class="Bool"("DisabledEnum"=w1692) -> ()  [unwired: 2 in, 2 out]
          }
          frame Enabled {
          }
        }
      }
      frame "Log Fuel Change" {
        n751 = Get Date/Time In Seconds() -> (seconds since 1Jan1904=w1700:timestamp)
        n752 = Unbundle By Name(w1702) -> ("Fuel Log Path"=w1699:path)
        n753 = Format Date/Time String(seconds (now)=w1700) -> (date/time string=w1698:string)  [unwired: 2 in]
        n754 = Build Array(w1698) -> (w1697:string[])
        n755 = call-poly <vilib>:"Write To Spreadsheet File.vi"("delimiter (\\t)"="," ("delimiter (\\t)"), "append to file? (new file:F)"=TRUE, "1D data"=w1697, "file path (dialog if empty)"=w1699) -> ()  [unwired: 4 in, 1 out]
      }
      frame "Fuel Change Popup" {
        w1703 = T15[] [enum."Enable Background"] items=["Main", "Init Files", "Init", "Unused", "Save As", "Start Profile", "Check Step Time", "Alarm", "Alarm Dismiss", "Run Step", "Stop Profile", "Cycle Reset", "Time Reset", "Time Reset All", "Time Set", "Tare CTs", "Save Profile", "Open Profile", "Get Profiles", "Update Screen", "Update Controls", "Save App Config", "Write Outputs", "Disable Background", "Enable Background", "Get/Release Control", "Log Fuel Change", "Fuel Change Popup", "Read Inputs", "Remote Timer Reset", "Controller Change", "Get Alarms", "Init Alarms", "Save Alarms", "Voltage Selection", "Set Watlow Temp 1", "Set Watlow Temp 2", "Get Pressure", "Write Tare Pressure", "Adjust Controls", "Reinit ADC", "Write Initial Times", "Write Pumps Present", "HMI Command", "Save Pump Times", "Check Pump Stop Time", "Save LS App Config", "Init Data File", "Reset LS Cycles", "Reset Anomalies", "Reset Opens", "Save LS Data", "Save LS Test Data", "Check Serial Numbers", "Main Tab", "Allow Data Note"]
        n756 = while {
          stop <- "pb.Fuel Change OK" stop-if-true
          n757 = property on="Fuel Change Tab" class="TabCtl (strict)"("Visible"=TRUE) -> ()  [unwired: 2 in, 2 out]
          n758 = Wait (ms)(milliseconds to wait=u32 20) -> ()  [unwired: 1 out]
        }
        n759 = Insert Into Array(array=w1707, index=0, new element=w1703) -> (w1706:T15[])
      }
      frame "Controller Change" {
        n760 = disable-structure shown="Enabled" {
          disable-tunnel: w1717 -> [w1720 _]
          disable-tunnel: w1716 -> [w1719 w1762]
          disable-tunnel: [w1718 w1762] -> w1715
          frame Disabled {
            n761 = flat-sequence {
              tunnel: [w1725] -> w1722
              tunnel: [w1745] -> w1721
              tunnel: [w1732] -> w1718
              tunnel: w1719 -> [w1733]
              tunnel: w1720 -> [w1740]
              tunnel: w1719 -> [w1744]
              tunnel: w1722 -> [w1761]
              tunnel: w1721 -> [w1754]
              frame #0 {
                w1729 = dbl[] [0.0, 0.0, 0.0, 0.0, 0.0, 0.0] ("ControllerCurrent")
                # "Not updating properly."
                # "Need to write this here as well in case a non-CAN\ncontroller is chosen (otherwise, most recent CAN\ncode will continue to execute)."
                n762 = Unbundle By Name(w1744) -> ("Controller List"=w1726:T25, "App Config.Controller Type:"=w1723:T3)
                n763 = Index Array(array=w1726, index=w1723) -> (element=w1728:T50)
                n764 = Unbundle By Name(w1728) -> ("Frequency"=w1730:i32, "CommSeg"=w1731:i32, "Controller?"=w1745:bool, "High Command"=w1735:dbl, "Low Command"=w1736:dbl, "Command Step"=w1737:dbl, "Invert PWM"=w1727:bool)
                n765 = Equal?(x=1, y=w1731) -> (x = y?=w1725:bool)
                n766 = case shown="False" w1725 {
                  tunnel: [w1749 fxp<+,32,16> 1.0 ("CommFactor")] -> w1742
                  tunnel: w1731 -> [w1750 _]
                  frame False {
                    n767 = case shown="10, Default" w1750 {
                      tunnel: [fxp<+,32,16> 4.0 ("CommFactor") fxp<+,32,16> 5.0 ("CommFactor")] -> w1749
                      frame 8 {
                      }
                      frame 10, Default {
                      }
                    }
                  }
                  frame True {
                  }
                }
                n768 = call "CAN Global.vi"("Controller Type:"=w1723, "Write (F)"=TRUE) -> ()  [unwired: 10 in, 4 out]
                n769 = property on="ControllerCurrent" class="Arr (strict)"("Value"=w1729) -> ()  [unwired: 2 in, 2 out]
                n770 = local write "ControllerCurrent"(w1729) -> ()
                n771 = Divide(x=40000000.0 ("40 MHz"), y=w1730) -> (x/y=w1739:dbl)
                n772 = To Unsigned Long Integer(number=w1739) -> (unsigned 32bit integer=w1734:u32)
                n773 = xnode "Read/Write Control"("FPGA VI Reference In"=w1740, "Brushless"=w1725, "CommFactor"=w1742, "RPMhyst"="RPMhyst", "PWM Period (Ticks)"=w1734, "InvertPWM?"=w1727) -> ()  [unwired: 1 in, 2 out]
                n774 = disable-structure shown="Disabled" {
                  disable-tunnel: w1737 -> [w1748 _]
                  disable-tunnel: w1736 -> [w1747 _]
                  disable-tunnel: w1735 -> [w1746 _]
                  frame Disabled {
                    n775 = property on="Numeric" class="DigNum (strict)"("Maximum"=w1746, "Minimum"=w1747, "Increment"=w1748) -> ()  [unwired: 2 in, 2 out]
                  }
                  frame Enabled {
                  }
                }
                n776 = Bundle By Name(cluster=w1733, "Controller Config"=w1728) -> (w1732:T26)
              }
              frame #1 {
                n777 = Select(t="Pump\nCurrent\n(RMS)" ("Label.Text"), s=w1761, f="Pump\nCurrent\n(DC)" ("Label.Text")) -> (s? t:f=w1756:string)
                n778 = Select(t=T31."Enabled" ("Disabled"), s=w1754, f=T31."Disabled and Grayed Out" ("Disabled")) -> (s? t:f=w1757:T31)
                n779 = property on="PumpCurrent" class="Arr (strict)"("Caption.Text"=w1756) -> ()  [unwired: 2 in, 2 out]
                n780 = property on="ControllerCurrent" class="Arr (strict)"("DisabledEnum"=w1757) -> ()  [unwired: 2 in, 2 out]
              }
            }
          }
          frame Enabled {
          }
        }
        n781 = Insert Into Array(array=w1714, index=0, new element=Sequence_States."Voltage Selection" ("new element/subarray")) -> (w1713:T15[])
      }
      frame "Voltage Selection" {
        # "Delete out controller voltage\nrows to make array correct size"
        n782 = Unbundle By Name(w1772) -> ("Controller Config.Controller?"=w1764:bool, "CalArray"=w1769:dbl[][])
        n783 = Delete From Array(array=w1769, length=6, index (row)=48) -> (deleted portion=w1765:dbl[][], array with subset deleted=w1766:dbl[][])  [unwired: 1 in]
        n784 = case shown="False" w1764 {
          tunnel: w1766 -> [w1776 w1779]
          tunnel: w1765 -> [_ w1778]
          tunnel: [w1776 w1777] -> w1763
          frame False {
            # "Voltage @ Pump\nNo Change"
          }
          frame True {
            # "Switch Voltage\ncoefficients to \nthe controller"
            n785 = for {
              tunnel: w1778 -> [w1782] mode=indexing
              shift-right: [w1781] -> w1777
              shift-left: w1779 -> [w1783]
              i -> [w1780]
              n786 = Replace Array Subset(array=w1783, new element=w1782, index (row)=w1780) -> (w1781:dbl[][])  [unwired: 1 in]
            }
          }
        }
        n787 = Select(t="Controller\nVoltage\n(V)" ("Caption.Text"), s=w1764, f="Pump\nVoltage\n(V)" ("Caption.Text")) -> (s? t:f=w1775:string)
        n788 = property on="Voltages" class="Arr (strict)"("Caption.Text"=w1775) -> ()  [unwired: 2 in, 2 out]
        n789 = call "Tank Data Global.vi"("Pump Data Mode"=Pump_Data_Mode."Write Cal", "Cal Coefficients"=w1763) -> ()  [unwired: 10 in, 4 out]
      }
      frame "Set Watlow Temp 1", "Set Watlow Temp 2" {
        n790 = Unbundle By Name(w1792) -> ("Tank CMDs.Temp 1 CMD"=w1791:dbl, "Tank CMDs.Temp 2 CMD"=w1790:dbl)
        n791 = To Single Precision Float(number=w1791) -> (single precision float=w1789:sgl)
        n792 = To Single Precision Float(number=w1790) -> (single precision float=w1788:sgl)
        n793 = case shown="\"Set Watlow Temp 2\"" w1787 {
          tunnel: [Modbus_Mode."Tank 1 Write" ("Modbus Mode") Modbus_Mode."Tank 2 Write" ("Modbus Mode")] -> w1786
          tunnel: [Modbus_Variable."Setpoint" ("Variable") Modbus_Variable."Setpoint" ("Variable")] -> w1785
          tunnel: [w1794 w1797] -> w1784
          tunnel: w1789 -> [w1794 _]
          tunnel: w1788 -> [_ w1797]
          frame "Set Watlow Temp 1", Default {
          }
          frame "Set Watlow Temp 2" {
          }
        }
        n794 = call "Watlow Modbus.vi"("Modbus Mode"=w1786, "Data Write"=w1784, "Variable"=w1785) -> ()  [unwired: 7 in, 2 out]
      }
      frame "Get Pressure" {
        w1816 = T15[] [enum."Write Tare Pressure"] items=["Main", "Init Files", "Init", "Unused", "Save As", "Start Profile", "Check Step Time", "Alarm", "Alarm Dismiss", "Run Step", "Stop Profile", "Cycle Reset", "Time Reset", "Time Reset All", "Time Set", "Tare CTs", "Save Profile", "Open Profile", "Get Profiles", "Update Screen", "Update Controls", "Save App Config", "Write Outputs", "Disable Background", "Enable Background", "Get/Release Control", "Log Fuel Change", "Fuel Change Popup", "Read Inputs", "Remote Timer Reset", "Controller Change", "Get Alarms", "Init Alarms", "Save Alarms", "Voltage Selection", "Set Watlow Temp 1", "Set Watlow Temp 2", "Get Pressure", "Write Tare Pressure", "Adjust Controls", "Reinit ADC", "Write Initial Times", "Write Pumps Present", "HMI Command", "Save Pump Times", "Check Pump Stop Time", "Save LS App Config", "Init Data File", "Reset LS Cycles", "Reset Anomalies", "Reset Opens", "Save LS Data", "Save LS Test Data", "Check Serial Numbers", "Main Tab", "Allow Data Note"]
        n795 = flat-sequence {
          tunnel: [w1820] -> w1808
          frame #0 {
            n796 = call "Tank Data Global.vi"("Pump Data Mode"=Pump_Data_Mode."Write Pressure Offsets", "Pressure Offsets"=dbl[] [0.0, 0.0, 0.0, 0.0, 0.0, 0.0]) -> ()  [unwired: 10 in, 4 out]
          }
          frame #1 {
            # "Wait for write to occur."
            n797 = Wait (ms)(milliseconds to wait=u32 500) -> ()  [unwired: 1 out]
          }
          frame #2 {
            n798 = call "Tank Data Global.vi"("Pump Data Mode"=Pump_Data_Mode."Read") -> ("Tank Data OUT"=w1820:dbl[])  [unwired: 11 in, 3 out]
          }
        }
        n799 = Array Subset(array=w1808, index=30, length=6) -> (w1800:dbl[])
        n800 = Bundle By Name(cluster=w1809, "Pressure Offsets"=w1800) -> (w1810:T26)
        n801 = To Double Precision Float(number=w1800) -> (double precision float=w1805:dbl[])
        n802 = Array To Spreadsheet String(delimiter (Tab)=",", array=w1805, 3:"%.2f" ("format string")) -> (spreadsheet string=w1803:string)
        n803 = Write to Text File(file (use dialog)=path "c:/PressureOffsets", text=w1803) -> (refnum out=w1802:refnum<file>, error out=w1801:errorcluster)  [unwired: 2 in, 1 out]
        n804 = Close File(refnum=w1802, error in=w1801) -> ()  [unwired: 2 out]
        n805 = Insert Into Array(array=w1814, index=0, new element=w1816) -> (w1813:T15[])
      }
      frame "Write Tare Pressure" {
        n806 = Unbundle By Name(w1824) -> ("Pressure Offsets"=w1822:dbl[])
        n807 = call "Tank Data Global.vi"("Pump Data Mode"=Pump_Data_Mode."Write Pressure Offsets", "Pressure Offsets"=w1822) -> ()  [unwired: 10 in, 4 out]
      }
      frame "Adjust Controls" {
        n808 = Unbundle By Name(w1833) -> ("App Config.Voltage Limits"=w1827:T42, "App Config.Voltage Far PI"=w1828:T43, "App Config.Voltage Mid PI"=w1829:T44, "App Config.Voltage Close PI"=w1830:T45, "App Config.Voltage Scale"=w1831:cluster{"V_FFm":dbl, "V_FFb":dbl}, "App Config.Voltage Cutoffs"=w1826:cluster{"V_MidCutoff":dbl, "V_CloseCutoff":dbl})
        n809 = call "PI with FF.vi"("Cutoffs"=w1826, "FFcluster"=w1831, "ClosePIcluster"=w1830, "MidPIcluster"=w1829, "FarPIcluster"=w1828, "LimitCluster"=w1827, "Init (F)"=TRUE) -> ()  [unwired: 8 in, 1 out]
      }
      frame "Reinit ADC" {
        n810 = call "Init OneHour FPGA.vi"("FPGA OneHour"=w1836) -> ("error out"=w1837:errorcluster, "FPGA OneHour Out"=w1835:T27)  [unwired: 9 in]
        n811 = feedback #7(0) -> (w1838:i32)
        "ADC Errors" <- w1838
        n812 = Increment(x=w1838) -> (x+1=w1839:i32)
        n813 = feedback-in #7(w1839) -> ()
        n814 = disable-structure shown="Disabled" {
          disable-tunnel: w1835 -> [w1844 _]
          disable-tunnel: w1837 -> [w1843 _]
          frame Disabled {
            n815 = call "Init ADCs.vi"("Error IN"=w1843, "FPGA Ref"=w1844) -> ()  [unwired: 7 in, 3 out]
          }
          frame Enabled {
          }
        }
      }
      frame "Write Initial Times" {
        w1848 = T15[] [enum."Read Inputs", enum."Save Pump Times"] items=["Main", "Init Files", "Init", "Unused", "Save As", "Start Profile", "Check Step Time", "Alarm", "Alarm Dismiss", "Run Step", "Stop Profile", "Cycle Reset", "Time Reset", "Time Reset All", "Time Set", "Tare CTs", "Save Profile", "Open Profile", "Get Profiles", "Update Screen", "Update Controls", "Save App Config", "Write Outputs", "Disable Background", "Enable Background", "Get/Release Control", "Log Fuel Change", "Fuel Change Popup", "Read Inputs", "Remote Timer Reset", "Controller Change", "Get Alarms", "Init Alarms", "Save Alarms", "Voltage Selection", "Set Watlow Temp 1", "Set Watlow Temp 2", "Get Pressure", "Write Tare Pressure", "Adjust Controls", "Reinit ADC", "Write Initial Times", "Write Pumps Present", "HMI Command", "Save Pump Times", "Check Pump Stop Time", "Save LS App Config", "Init Data File", "Reset LS Cycles", "Reset Anomalies", "Reset Opens", "Save LS Data", "Save LS Test Data", "Check Serial Numbers", "Main Tab", "Allow Data Note"]
        n816 = Unbundle By Name(w1850) -> ("Initial Times"=w1849:dbl[])
        n817 = call "Tank Data Global.vi"("Pump Data Mode"=Pump_Data_Mode."Write Initial Times", "Intitial Times"=w1849) -> ()  [unwired: 10 in, 4 out]
        n818 = Insert Into Array(array=w1846, index=0, new element=w1848) -> (w1845:T15[])
      }
      frame "Write Pumps Present" {
        w1867 = T15[] [enum."Write Outputs", enum."Update Controls"] items=["Main", "Init Files", "Init", "Unused", "Save As", "Start Profile", "Check Step Time", "Alarm", "Alarm Dismiss", "Run Step", "Stop Profile", "Cycle Reset", "Time Reset", "Time Reset All", "Time Set", "Tare CTs", "Save Profile", "Open Profile", "Get Profiles", "Update Screen", "Update Controls", "Save App Config", "Write Outputs", "Disable Background", "Enable Background", "Get/Release Control", "Log Fuel Change", "Fuel Change Popup", "Read Inputs", "Remote Timer Reset", "Controller Change", "Get Alarms", "Init Alarms", "Save Alarms", "Voltage Selection", "Set Watlow Temp 1", "Set Watlow Temp 2", "Get Pressure", "Write Tare Pressure", "Adjust Controls", "Reinit ADC", "Write Initial Times", "Write Pumps Present", "HMI Command", "Save Pump Times", "Check Pump Stop Time", "Save LS App Config", "Init Data File", "Reset LS Cycles", "Reset Anomalies", "Reset Opens", "Save LS Data", "Save LS Test Data", "Check Serial Numbers", "Main Tab", "Allow Data Note"]
        # "Power and Ignition relays can only turn of if pumps are present."
        n819 = Unbundle By Name(w1856) -> ("App Config.Pumps Present"=w1859:T8, "Power Relay"=w1863:T8, "Ignition Relay"=w1862:T8)
        n820 = Cluster To Array(cluster=w1859) -> (array=w1852:bool[])
        n821 = Cluster To Array(cluster=w1863) -> (array=w1861:bool[])
        n822 = Cluster To Array(cluster=w1862) -> (array=w1860:bool[])
        n823 = call "Tank Data Global.vi"("Pump Data Mode"=Pump_Data_Mode."Write Pumps Present", "Pumps Present"=w1852) -> ()  [unwired: 10 in, 4 out]
        n824 = And(x=w1861, y=w1852) -> (x .and. y?=w1858:bool[])
        n825 = And(x=w1860, y=w1852) -> (x .and. y?=w1857:bool[])
        n826 = Array To Cluster(array=w1858) -> (cluster=w1854:T51)
        n827 = Array To Cluster(array=w1857) -> (cluster=w1853:T51)
        n828 = Bundle By Name(cluster=w1856, "Power Relay"=w1854, "Ignition Relay"=w1853) -> (w1855:T26)
        n829 = Insert Into Array(array=w1865, index=0, new element=w1867) -> (w1864:T15[])
      }
      frame "HMI Command" {
        w1870 = T15[] [] items=["Main", "Init Files", "Init", "Unused", "Save As", "Start Profile", "Check Step Time", "Alarm", "Alarm Dismiss", "Run Step", "Stop Profile", "Cycle Reset", "Time Reset", "Time Reset All", "Time Set", "Tare CTs", "Save Profile", "Open Profile", "Get Profiles", "Update Screen", "Update Controls", "Save App Config", "Write Outputs", "Disable Background", "Enable Background", "Get/Release Control", "Log Fuel Change", "Fuel Change Popup", "Read Inputs", "Remote Timer Reset", "Controller Change", "Get Alarms", "Init Alarms", "Save Alarms", "Voltage Selection", "Set Watlow Temp 1", "Set Watlow Temp 2", "Get Pressure", "Write Tare Pressure", "Adjust Controls", "Reinit ADC", "Write Initial Times", "Write Pumps Present", "HMI Command", "Save Pump Times", "Check Pump Stop Time", "Save LS App Config", "Init Data File", "Reset LS Cycles", "Reset Anomalies", "Reset Opens", "Save LS Data", "Save LS Test Data", "Check Serial Numbers", "Main Tab", "Allow Data Note"]
        n830 = flat-sequence {
          tunnel: [w1884] -> w1871
          frame #0 {
            n831 = call "RPi HMI Global.vi"("Mode"=HMI_Global_Mode."Reset Cmd") -> ()  [unwired: 10 in, 1 out]
          }
          frame #1 {
            n832 = call "RPi HMI Global.vi"("Mode"=HMI_Global_Mode."Read") -> ("HMI Cluster OUT"=w1884:T17)  [unwired: 10 in]
          }
        }
        n833 = Unbundle By Name(w1871) -> ("Power Relays"=w1880:T8, "Pump CMDs"=w1879:dbl[], "Tank CMDs.PS CMD"=w1878:dbl, "Tank CMDs.Press CMD"=w1877:dbl, "Tank CMDs.Temp 1 CMD"=w1876:dbl, "Tank CMDs.Temp 2 CMD"=w1875:dbl, "HMI Tog Buttons.Start Test"=w1874:bool)
        n834 = local write "Power Relay"(w1880) -> ()
        n835 = local write "Controller\nCMD"(w1879) -> ()
        n836 = local write "Power Supply Cmd:"(w1878) -> ()
        n837 = local write "PressureCMD"(w1877) -> ()
        n838 = local write "Tank 1 Temp Cmd:"(w1876) -> ()
        n839 = local write "Tank 2 Temp Cmd:"(w1875) -> ()
        n840 = local write "pb.Run Profile"(w1874) -> ()
        n841 = Insert Into Array(array=w1881, index=0, new element=w1870) -> (w1869:T15[])
        n842 = Bundle By Name(cluster=w1873, "HMI"=w1871) -> (w1872:T26)
      }
      frame "Init Data File" {
        n843 = Get Date/Time In Seconds() -> (seconds since 1Jan1904=w1887:timestamp)
        n844 = Unbundle By Name(w1901) -> ("App Config.CA Number"=w1896:string, "LS App Config.Data File Name:"=w1897:string, "LS App Config.Serial Numbers"=w1892:string[])
        n845 = Format Date/Time String(time format string (%c)="_%m%d%y.csv", seconds (now)=w1887) -> (date/time string=w1886:string)  [unwired: 1 in]
        n846 = Empty String/Path?(string/path=w1897) -> (empty?=w1895:bool)
        n847 = Empty String/Path?(string/path=w1896) -> (empty?=w1894:bool)
        n848 = call "Remove illegal file characters.vi"("Filename In"=w1896) -> ("Filename Out"=w1890:string)  [unwired: 10 in]
        n849 = call "Remove illegal file characters.vi"("Filename In"=w1897) -> ("Filename Out"=w1889:string)  [unwired: 10 in]
        n850 = Or(x=w1895, y=w1894) -> (x .or. y?=w1891:bool)
        n851 = Build Path(base path=path "u:/CA Numbers", name or relative path=w1890) -> (appended path=w1898:path)
        n852 = case shown="False" w1891 {
          tunnel: w1898 -> [_ w1918]
          tunnel: w1886 -> [_ w1913]
          tunnel: w1889 -> [_ w1911]
          tunnel: [path "" ("LS Data Filepath") w1906] -> w1893
          tunnel: w1892 -> [_ w1904]
          frame True {
          }
          frame False {
            n853 = call <vilib>:"Check if File or Folder Exists.vi"("path"=w1918) -> ("error out"=w1915:errorcluster, "file or folder exists?"=w1916:bool, "dup path"=w1917:path)  [unwired: 8 in]
            n854 = Concatenate Strings(w1911, w1913) -> (w1912:string)
            n855 = case shown="False" w1916 {
              tunnel: w1917 -> [w1938 w1939]
              tunnel: w1915 -> [w1935 w1940]
              tunnel: [w1936 w1940] -> _
              tunnel: [w1937 w1939] -> w1914
              frame False {
                n856 = Create Folder(path (use dialog)=w1938, error in=w1935) -> (created path=w1937:path, error out=w1936:errorcluster)  [unwired: 1 in, 1 out]
              }
              frame True {
              }
            }
            n857 = Build Path(base path=w1914, name or relative path=w1912) -> (appended path=w1910:path)
            n858 = call <vilib>:"Check if File or Folder Exists.vi"("path"=w1910) -> ("error out"=w1907:errorcluster, "file or folder exists?"=w1908:bool, "dup path"=w1909:path)  [unwired: 8 in]
            n859 = case shown="False" w1908 {
              tunnel: w1909 -> [w1933 w1934]
              tunnel: w1907 -> [w1932 _]
              tunnel: [w1930 w1934] -> w1906
              tunnel: "Timestamp,Pos 1 Voltage,Pos 2 Voltage,Pos 3 Voltage,Pos 4 Voltage,Pos 5 Voltage,Pos 6 Voltage,Pos 7 Voltage,Pos 8 Voltage,Pos 9 Voltage,Pos 10 Voltage,Pos 11 Voltage,Pos 12 Voltage,PS Voltage,Bank 1 State,Bank 2 State\n" -> [w1924 _]
              tunnel: w1904 -> [w1920 _]
              frame False {
                n860 = Array To Spreadsheet String(delimiter (Tab)=",", array=w1920, 3:"%s" ("format string")) -> (spreadsheet string=w1919:string)
                n861 = Open/Create/Replace File(file path (use dialog)=w1933, error in=w1932, operation (0:open)=T32."create") -> (refnum out=w1927:refnum<file>, error out=w1929:errorcluster)  [unwired: 3 in, 1 out]
                n862 = Concatenate Strings("Serial Numbers," ("string"), w1919, w1924) -> (w1923:string)
                n863 = Write to Text File(file (use dialog)=w1927, text=w1923, error in=w1929) -> (refnum out=w1926:refnum<file>, error out=w1928:errorcluster)  [unwired: 1 in, 1 out]
                n864 = Close File(refnum=w1926, error in=w1928) -> (path=w1930:path)  [unwired: 1 out]
              }
              frame True {
              }
            }
          }
        }
        n865 = local write "CA Number:"(w1890) -> ()
        n866 = local write "Data File Name:"(w1889) -> ()
        n867 = Bundle By Name(cluster=w1901, "App Config.CA Number"=w1890, "LS App Config.Data File Name:"=w1889, "LS Data Filepath"=w1893) -> (w1900:T26)
      }
      frame "Save LS Data" {
        n868 = Unbundle By Name(w1945) -> ("LS Data"=w1943:T16)
        n869 = Unbundle By Name(w1943) -> ("Opens"=w1942:i32[])
        n870 = Array Size(array=w1942) -> (size(s)=w1941:i32)
        n871 = case shown="12" w1941 {
          tunnel: w1943 -> [_ w1948]
          frame Default {
          }
          frame 12 {
            n872 = Write to Binary File(file (use dialog)=path "c:/Monitored Statistics" ("Path"), data=w1948) -> (refnum out=w1947:refnum<file>, error out=w1946:errorcluster)  [unwired: 4 in, 1 out]
            n873 = Close File(refnum=w1947, error in=w1946) -> ()  [unwired: 2 out]
          }
        }
      }
      frame "Save LS Test Data" {
        n874 = Unbundle By Name(w1959) -> ("LS App Config.Serial Numbers"=w1956:string[], "LS Data"=w1957:T16, "App Config.CA Number"=w1951:string, "LS App Config.Data File Name:"=w1952:string, "LS App Config.DetectionMode"=w1958:i32)
        n875 = Empty String/Path?(string/path=w1951) -> (empty?=w1954:bool)
        n876 = Empty String/Path?(string/path=w1952) -> (empty?=w1953:bool)
        n877 = Or(x=w1954, y=w1953) -> (x .or. y?=w1950:bool)
        n878 = case shown="False" w1950 {
          tunnel: w1951 -> [_ w1968]
          tunnel: w1952 -> [_ w1967]
          tunnel: w1958 -> [_ w1963]
          tunnel: w1957 -> [_ w1961]
          tunnel: w1956 -> [_ w1960]
          frame True {
          }
          frame False {
            n879 = Build Path(base path=path "u:/CA Numbers", name or relative path=w1968) -> (appended path=w1965:path)
            n880 = List Folder(path=w1965) -> (filenames=w1966:string[])  [unwired: 3 in, 3 out]
            n881 = while {
              tunnel: w1967 -> [w2011]
              tunnel: [w2009] -> w1964
              shift-right: [w2008] -> _
              shift-left: w1966 -> [w2008]
              i -> [w2013]
              stop <- w2006 stop-if-true
              n882 = Increment(x=w2013) -> (x+1=w2010:i32)
              n883 = Format Into String(format string="%s_Statistics%#f.csv", w2011, w2010) -> (resulting string=w2009:string)  [unwired: 2 in, 1 out]
              n884 = Search 1D Array(1D array=w2008, element=w2009) -> (index of element=w2007:i32)  [unwired: 1 in]
              n885 = Less Than 0?(x=w2007) -> (x < 0?=w2006:bool)
            }
            n886 = Build Path(base path=w1965, name or relative path=w1964) -> (appended path=w1962:path)
            n887 = case shown="1" w1963 {
              tunnel: w1962 -> [_ w1971]
              tunnel: w1961 -> [_ w2004]
              tunnel: w1960 -> [_ w2003]
              frame 0, Default {
                # "Anomalies"
              }
              frame 1 {
                # "Opens"
                n888 = Unbundle By Name(w2004) -> ("Opens"=w2002:i32[])
                n889 = Index Array(array=w2002) -> (element #1=w1989:i32, element #2=w1987:i32, element #3=w1986:i32, element #4=w1985:i32, element #5=w1984:i32, element #6=w1983:i32, element #7=w1982:i32, element #8=w1981:i32, element #9=w1980:i32, element #10=w1979:i32, element #11=w1978:i32, element #12=w1988:i32)  [unwired: 12 in]
                n890 = Index Array(array=w2003) -> (element #1=w2001:string, element #2=w2000:string, element #3=w1999:string, element #4=w1998:string, element #5=w1996:string, element #6=w1997:string, element #7=w1995:string, element #8=w1994:string, element #9=w1992:string, element #10=w1993:string, element #11=w1991:string, element #12=w1990:string)  [unwired: 12 in]
                n891 = Format Into String(format string=",Position 1,Position 2,Position 3,Position 4,Position 5,Position 6,Position 7,Position 8,Position 9,Position 10,Position 11,Position 12\nSerial Numbers,%s,%s,%s,%s,%s,%s,%s,%s,%s,%s,%s,%s\nOpens Detected,%f,%f,%f,%f,%f,%f,%f,%f,%f,%f,%f,%f", w2001, w2000, w1999, w1998, w1996, w1997, w1995, w1994, w1992, w1993, w1991, w1990, w1989, w1987, w1986, w1985, w1984, w1983, w1982, w1981, w1980, w1979, w1978, w1988) -> (resulting string=w1973:string, error out=w1972:errorcluster)  [unwired: 2 in]
                n892 = Open/Create/Replace File(file path (use dialog)=w1971, error in=w1972, operation (0:open)=T32."open or create") -> (refnum out=w1977:refnum<file>, error out=w1975:errorcluster)  [unwired: 3 in, 1 out]
                n893 = Write to Text File(file (use dialog)=w1977, text=w1973, error in=w1975) -> (refnum out=w1976:refnum<file>, error out=w1974:errorcluster)  [unwired: 1 in, 1 out]
                n894 = Close File(refnum=w1976, error in=w1974) -> ()  [unwired: 2 out]
              }
            }
          }
        }
      }
      frame "Check Serial Numbers" {
        n895 = Unbundle By Name(w2019) -> ("LS App Config.Serial Numbers"=w2015:string[])
        n896 = for {
          tunnel: w2015 -> [w2021] mode=indexing
          tunnel: [w2020] -> w2014 mode=indexing
          n897 = call "Remove illegal file characters.vi"("Filename In"=w2021) -> ("Filename Out"=w2020:string)  [unwired: 10 in]
        }
        n898 = Array To Cluster(array=w2014) -> (cluster=w2016:T52)
        n899 = Bundle By Name(cluster=w2019, "LS App Config.Serial Numbers"=w2014) -> (w2018:T26)
        n900 = local write "LS Serial Numbers"(w2016) -> ()
      }
      frame "Main Tab" {
        # "Justin wants Start Test, Stop Test, and Data File Name always unlocked\n\nSo moved Data File Name to where it wouldn't sit on top of another\ncontrol on another page when I made it float like the stop button"
        n901 = Unbundle By Name(w2025) -> ("Main Tab"=w2024:T9)
        n902 = case shown="Default" w2024 {
          tunnel: [T31."Enabled" ("Disabled") T31."Disabled" ("Disabled")] -> w2023
          tunnel: [TRUE ("Visible") FALSE ("Visible")] -> w2022
          frame "Main" {
          }
          frame Default {
          }
        }
        n903 = property on="pb.Run Profile" class="Bool (strict)"("Visible"=w2022, "DisabledEnum"=w2023) -> ()  [unwired: 2 in, 2 out]
        n904 = property on="Data File Name:" class="Str"("Visible"=w2022, "DisabledEnum"=w2023) -> ()  [unwired: 2 in, 2 out]
      }
      frame "Allow Data Note" {
        w2036 = T15[] [enum."Enable Background"] items=["Main", "Init Files", "Init", "Unused", "Save As", "Start Profile", "Check Step Time", "Alarm", "Alarm Dismiss", "Run Step", "Stop Profile", "Cycle Reset", "Time Reset", "Time Reset All", "Time Set", "Tare CTs", "Save Profile", "Open Profile", "Get Profiles", "Update Screen", "Update Controls", "Save App Config", "Write Outputs", "Disable Background", "Enable Background", "Get/Release Control", "Log Fuel Change", "Fuel Change Popup", "Read Inputs", "Remote Timer Reset", "Controller Change", "Get Alarms", "Init Alarms", "Save Alarms", "Voltage Selection", "Set Watlow Temp 1", "Set Watlow Temp 2", "Get Pressure", "Write Tare Pressure", "Adjust Controls", "Reinit ADC", "Write Initial Times", "Write Pumps Present", "HMI Command", "Save Pump Times", "Check Pump Stop Time", "Save LS App Config", "Init Data File", "Reset LS Cycles", "Reset Anomalies", "Reset Opens", "Save LS Data", "Save LS Test Data", "Check Serial Numbers", "Main Tab", "Allow Data Note"]
        n905 = flat-sequence {
          tunnel: [w2046] -> w2035
          tunnel: [w2045] -> w2034
          tunnel: w2033 -> [w2044]
          tunnel: [w2043] -> w2032
          tunnel: w2035 -> [w2058]
          tunnel: w2034 -> [w2059]
          tunnel: w2032 -> [w2057]
          tunnel: [w2054] -> w2031
          tunnel: w2031 -> [w2075]
          frame #0 {
            w2040 = FALSE ("Visible")
            n906 = property on="Note Tab" class="TabCtl (strict)"("Visible"=TRUE) -> ()  [unwired: 2 in, 2 out]
            n907 = property on="Normal Steps:" class="DigNum (strict)"("Visible"=w2040) -> ()  [unwired: 2 in, 2 out]
            n908 = property on="Step Threshold:" class="DigNum (strict)"("Visible"=w2040) -> ()  [unwired: 2 in, 2 out]
            n909 = property on="Cycle Pts to Avg:" class="DigNum (strict)"("Visible"=w2040) -> ()  [unwired: 2 in, 2 out]
            n910 = property on="Cycle Threshold:" class="DigNum (strict)"("Visible"=w2040) -> ()  [unwired: 2 in, 2 out]
            n911 = property on="pb.Stop Profile" class="Bool"("Visible"=w2040) -> ()  [unwired: 2 in, 2 out]
            n912 = property on="Data File Name:" class="Str"("Visible"=w2040) -> ()  [unwired: 2 in, 2 out]
            n913 = property on="pb.Run Profile" class="Bool (strict)"("Visible"=w2040) -> ()  [unwired: 2 in, 2 out]
            n914 = property on="Anomaly Threshold:" class="DigNum (strict)"("Visible"=w2040) -> ()  [unwired: 2 in, 2 out]
            n915 = property on="Second Step Check" class="Bool (strict)"("Visible"=w2040) -> ()  [unwired: 2 in, 2 out]
            n916 = property on="Main Tab" class="TabCtl (strict)"("DisabledEnum"=T31."Enabled" ("Disabled")) -> ()  [unwired: 2 in, 2 out]
          }
          frame #1 {
            n917 = while {
              tunnel: ["pb.Note OK"] -> w2048
              stop <- w2052 stop-if-true
              n918 = Wait (ms)(milliseconds to wait=u32 10) -> ()  [unwired: 1 out]
              n919 = local write "Main Tab"(T9."Configure" ("Main Tab")) -> ()
              n920 = Or(x="pb.Note Cancel", y="pb.Note OK") -> (x .or. y?=w2052:bool)
            }
            n921 = Unbundle By Name(w2044) -> ("Login"=w2043:bool, "LS Data Filepath"=w2045:path, "LS App Config.Record Bursts"=w2047:bool)
            n922 = And(x=w2047, y=w2048) -> (x .and. y?=w2046:bool)
          }
          frame #2 {
            n923 = case shown="True" w2058 {
              tunnel: w2059 -> [_ w2061]
              frame False {
              }
              frame True {
                n924 = Open/Create/Replace File(file path (use dialog)=w2061, operation (0:open)=T32."open or create") -> (refnum out=w2069:refnum<file>, error out=w2070:errorcluster)  [unwired: 4 in, 1 out]
                n925 = Concatenate Strings("Note:,", "Stop Profile Note", "\n") -> (w2062:string)
                n926 = Set File Position(refnum=w2069, from (0:start)=enum16{"start", "end", "current"}."end", error in=w2070) -> (refnum out=w2073:refnum<file>, error out=w2072:errorcluster)  [unwired: 1 in]
                n927 = Write to Text File(file (use dialog)=w2073, text=w2062, error in=w2072) -> (refnum out=w2066:refnum<file>, error out=w2065:errorcluster)  [unwired: 1 in, 1 out]
                n928 = Close File(refnum=w2066, error in=w2065) -> (error out=w2067:errorcluster)  [unwired: 1 out]
                n929 = call <vilib>:"Clear Errors.vi"("error in (no error)"=w2067) -> ()  [unwired: 6 in, 1 out]
              }
            }
            n930 = Select(t=T31."Enabled" ("Disabled"), s=w2057, f=T31."Disabled" ("Disabled")) -> (s? t:f=w2054:T31)
          }
          frame #3 {
            w2074 = TRUE ("Visible")
            n931 = local write "Stop Profile Note"("" ("Stop Profile Note")) -> ()
            n932 = local write "Main Tab"(T9."Main" ("Main Tab")) -> ()
            n933 = property on="Main Tab" class="TabCtl (strict)"("DisabledEnum"=w2075) -> ()  [unwired: 2 in, 2 out]
            n934 = property on="Note Tab" class="TabCtl (strict)"("Visible"=FALSE) -> ()  [unwired: 2 in, 2 out]
            n935 = property on="Normal Steps:" class="DigNum (strict)"("Visible"=w2074) -> ()  [unwired: 2 in, 2 out]
            n936 = property on="Step Threshold:" class="DigNum (strict)"("Visible"=w2074) -> ()  [unwired: 2 in, 2 out]
            n937 = property on="Cycle Pts to Avg:" class="DigNum (strict)"("Visible"=w2074) -> ()  [unwired: 2 in, 2 out]
            n938 = property on="Cycle Threshold:" class="DigNum (strict)"("Visible"=w2074) -> ()  [unwired: 2 in, 2 out]
            n939 = property on="pb.Stop Profile" class="Bool"("Visible"=w2074) -> ()  [unwired: 2 in, 2 out]
            n940 = property on="Data File Name:" class="Str"("Visible"=w2074) -> ()  [unwired: 2 in, 2 out]
            n941 = property on="pb.Run Profile" class="Bool (strict)"("Visible"=w2074) -> ()  [unwired: 2 in, 2 out]
            n942 = property on="Anomaly Threshold:" class="DigNum (strict)"("Visible"=w2074) -> ()  [unwired: 2 in, 2 out]
            n943 = property on="Second Step Check" class="Bool (strict)"("Visible"=w2074) -> ()  [unwired: 2 in, 2 out]
          }
        }
        n944 = Insert Into Array(array=w2039, index=0, new element=w2036) -> (w2038:T15[])
      }
    }
  }
  n945 = flat-sequence {
    tunnel: w4 -> [_]
    tunnel: w3 -> [w2079]
    frame #0 {
      n946 = disable-structure shown="Disabled" {
        disable-tunnel: w2079 -> [w2081 _]
        frame Disabled {
          n947 = call "Data Loop.vi"("FPGA Ref"=w2081) -> ()  [unwired: 10 in, 1 out]
        }
        frame Enabled {
        }
      }
      n948 = disable-structure shown="Disabled" {
        disable-tunnel: w2079 -> [w2080 _]
        frame Disabled {
          n949 = call "Power Supply Loop.vi"("FPGA Ref"=w2080) -> ()  [unwired: 11 in]
          n950 = call "Data Logger Loop.vi"() -> ()  [unwired: 20 in]
          n951 = call "CAN Loop.vi"() -> ()  [unwired: 12 in]
        }
        frame Enabled {
        }
      }
      n952 = call "Email Loop.vi"() -> ()  [unwired: 12 in]
      n953 = disable-structure shown="Disabled" {
        frame Disabled {
          n954 = call "Watlow Loop.vi"() -> ()  [unwired: 12 in]
        }
        frame Enabled {
        }
      }
      n955 = call "App Loop.vi"() -> ()  [unwired: 12 in]
      n956 = disable-structure shown="Disabled" {
        frame Disabled {
          n957 = call "RPi HMI Loop.vi"() -> ()  [unwired: 20 in]
        }
        frame Enabled {
        }
      }
      n958 = call "LS One Hour Data Loop.vi"("FPGA OneHour Ref"=w2079) -> ()  [unwired: 11 in]
    }
  }
  n959 = disable-structure shown="Disabled" {
    disable-tunnel: w3 -> [w2082 _]
    frame Disabled {
      n960 = while {
        tunnel: w2082 -> [w2085]
        stop <- FALSE stop-if-true
        n961 = local read "Main Tab"() -> (w2083:T9)
        n962 = case shown="\"Live Graph\"" w2083 {
          tunnel: w2085 -> [_ w2088]
          frame Default {
            n963 = Wait (ms)(milliseconds to wait=u32 10) -> ()  [unwired: 1 out]
          }
          frame "Live Graph" {
            n964 = case shown="False" "Pause" {
              tunnel: w2088 -> [w2097 _]
              frame False {
                n965 = xnode "Read/Write Control"("FPGA VI Reference In"=w2097) -> ("Analog Inputs"=w2090:fxp<+/-,28,17>[])  [unwired: 1 in, 2 out]
                n966 = Decrement(x="Position") -> (x-1=w2094:i32)
                n967 = In Range and Coerce(upper limit=11, x=w2094, lower limit=0) -> (coerced(x)=w2093:i32)  [unwired: 1 out]
                n968 = Index Array(array=w2090, index=w2093) -> (element=→"Waveform Chart":fxp<+/-,28,17>)
                n969 = Wait (ms)(milliseconds to wait=u32 1) -> ()  [unwired: 1 out]
              }
              frame True {
                n970 = Wait (ms)(milliseconds to wait=u32 10) -> ()  [unwired: 1 out]
              }
            }
          }
        }
      }
    }
    frame Enabled {
    }
  }
